vi "main.vi"() -> ()   [LabVIEW 2019]
uses:
  <vilib>/Utility/error.llb/DialogType.ctl
  <vilib>/userDefined/High Color/IMAQdx.ctl
  <vilib>/measure/mamon.llb/Trigger Detection for 1 Channel.vi
  <userlib>/DAQNavi Polymorphic VI/create/DAQNavi Create Channel(AO-Voltage).vi
  <userlib>/DAQNavi Polymorphic VI/create/DAQNavi Create Channel(DO-Digital Output).vi
  <userlib>/DAQNavi Polymorphic VI/create/DAQNavi Create Channel(DI-Digital Input).vi
  <userlib>/DAQNavi Polymorphic VI/read/DAQNavi Read (Digital 1D U8 NChan 1Samp).vi
  Setting Lib.lvlib
  detectedPellet.lvlib
  D03.lvlib
  D04.lvlib
  D05.lvlib
  database.lvlib
  <vilib>/measure/NI_MAPro.lvlib
  User Lib.lvlib
  <vilib>/addons/Fuzzy Logic/NI_Fuzzy_Logic_API.lvlib
  Maintenance.lvlib
  D01.lvlib
  D02.lvlib
  D06.lvlib
panel:
  out "error out 2":errorcluster
  out "task out digital":i32
  out "task out analog":i32
  out "last error 06":dbl
  out "slope D06":dbl
  out "decrease D06":bool
  out "no change D06":bool
  out "increase D06":bool
  out "sudden change D06":bool
  out "In Range":dbl format="%#.2g"
  out "Warning array 06":bool[](array[boolean])
  out "speed  min 06":bool
  out "speed max 06":bool
  out "10-14 6":dbl(slide) caption="10-14 mm" scale=0.0..100.0 scale format="%#.1f"
  out "8-16mm 6":dbl format="%.1g"
  out "AUTO/MAN 06":bool
  out "DISC 06":bool
  out "SPEED 07":dbl caption="SPEED" format="%#.2g"
  out "AVG 07":dbl caption="AVG" format="%#.2g"
  in  "Info 07":bool
  out "Warning 07":bool
  out "disc name 07":string="DISC 07"
  in  "Graph 07":bool
  in  "Live 07":bool
  out "AUTO/MAN 07":bool
  out "projector 07":bool
  out "cam 07":bool
  out "8-12.5 32":dbl(slide) caption="9-12.5 mm" scale=0.0..100.0 scale format="%#.1f"
  out "12.5-16 32":dbl(slide) caption="12.5-16 mm" scale=0.0..100.0 scale format="%#.1f"
  out "DISC 07":bool
  out "SPEED 06":dbl caption="SPEED" format="%.2g"
  out "AVG 06":dbl caption="AVG" format="%#.2g"
  in  "Info 06":bool
  out "Warning 06":bool
  out "disc name 06":string="DISC 06"
  in  "Graph 06":bool
  in  "Live 06":bool
  out "projector 06":bool
  out "cam 06":bool
  out "9.5-12.7 06":dbl(slide) caption="9.5-12.7 mm" scale=0.0..100.0 scale format="%#.1f"
  out "12.7-16 06":dbl(slide) caption="12.7-16 mm" scale=0.0..100.0 scale format="%#.1f"
  out "sudden change D05":bool
  out "slope D05":dbl
  out "increase D05":bool
  out "decrease D05":bool
  out "sudden change D04":bool
  out "slope D04":dbl
  out "increase D04":bool
  out "decrease D04":bool
  out "slope D03":dbl
  out "sudden change D03":bool
  out "increase D03":bool
  out "decrease D03":bool
  out "sudden change D02":bool
  out "slope D02":dbl
  out "increase D02":bool
  out "decrease D02":bool
  out "decrease D01":bool
  out "increase D01":bool
  out "last error 05":dbl
  out "no change D05":bool
  out "last error 04":dbl
  out "no change D04":bool
  out "last error 03":dbl
  out "no change D03":bool
  out "last error 02":dbl
  out "no change D02":bool
  out "sudden change D01":bool
  out "speed  min 05":bool
  out "speed max 05":bool
  out "speed  min 03":bool
  out "speed max 03":bool
  out "speed  min 04":bool
  out "speed max 04":bool
  out "speed  min 02":bool
  out "speed max 02":bool
  out "speed max 01":bool
  out "speed  min 01":bool
  out "no change D01":bool
  out "SPEED 05":dbl caption="SPEED" format="%.2g"
  out "SPEED 04":dbl caption="SPEED" format="%.2g"
  out "SPEED 03":dbl caption="SPEED" format="%.2g"
  out "SPEED 02":dbl caption="SPEED" format="%.2g"
  out "SPEED 01":dbl caption="SPEED" format="%.2g"
  out "AVG 05":dbl caption="AVG" format="%#.2g"
  out "AVG 04":dbl caption="AVG" format="%#.2g"
  out "AVG 03":dbl caption="AVG" format="%#.2g"
  out "AVG 02":dbl caption="AVG" format="%#.2g"
  out "AVG 01":dbl caption="AVG" format="%#.2g"
  out "8-16mm 05":dbl format="%.1g"
  out "8-16mm 04":dbl format="%.1g"
  out "8-16mm 03":dbl format="%.1g"
  out "8-16mm 27":dbl format="%.1g"
  out "8-16mm 26":dbl format="%.1g"
  out "10-14 05":dbl(slide) caption="10-14 mm" scale=0.0..100.0 scale format="%#.1f"
  out "10-14 04":dbl(slide) caption="10-14 mm" scale=0.0..100.0 scale format="%#.1f"
  out "10-14 03":dbl(slide) caption="10-14 mm" scale=0.0..100.0 scale format="%#.1f"
  out "10-14 02":dbl(slide) caption="10-14 mm" scale=0.0..100.0 scale format="%#.1f"
  out "10-14 01":dbl(slide) caption="10-14 mm" scale=0.0..100.0 scale format="%#.1f"
  out "error out 14":errorcluster
  out "error out 12":errorcluster
  in  "Info 05":bool
  in  "Info 04":bool
  in  "Info 03":bool
  in  "Info 02":bool
  in  "Info 01":bool
  out "error out":errorcluster
  out "avg grading array size":i32=4000
  out "live grading array size":i32=2000
  out "2D array out":dbl[][](array[numeric])
  out "Warning array 01":bool[](array[boolean])
  out "Warning array 02":bool[](array[boolean])
  out "Warning array 03":bool[](array[boolean])
  out "Warning array 04":bool[](array[boolean])
  out "Warning array 05":bool[](array[boolean])
  out "Warning 05":bool
  in  "speed disc 30":i32
  in  "speed disc 29":i32
  in  "Error in 18":errorcluster
  in  "speed disc 28":i32
  in  "speed disc 27":i32
  in  "speed disc 26":i32
  out "Warning 04":bool
  out "Warning 03":bool
  out "Warning 02":bool
  out "Warning 01":bool
  out "overal result":string="Overal Result"
  out "disc name 05":string="DISC 05"
  out "disc name 04":string="DISC 04"
  out "disc name 03":string="DISC 03"
  out "disc name 02":string="DISC 02"
  in  "Setting":bool
  out "disc name 01":string="DISC 01"
  in  "Graph 05":bool
  in  "Live 05":bool
  in  "Graph 04":bool
  in  "Live 04":bool
  in  "Graph 03":bool
  in  "Live 03":bool
  in  "Graph 02":bool
  in  "Live 02":bool
  out "Software name":string="DORSA Smart Grading System (DSGS)"
  out "time&date":string="2020/11/22"
  in  "Maintenance":bool
  in  "Shutdown":bool
  in  "Restart":bool
  in  "Close":bool
  in  "View":bool
  in  "Report":bool
  in  "Login":bool=TRUE
  in  "Graph 01":bool
  in  "Live 01":bool
  out "9.5-12.7 02":dbl(slide) caption="9.5-12.7 mm" scale=0.0..100.0 scale format="%#.1f"
  out "12.7-16 02":dbl(slide) caption="12.7-16 mm" scale=0.0..100.0 scale format="%#.1f"
  out "AUTO/MAN 05":bool
  out "projector 05":bool
  out "cam 05":bool
  out "9.5-12.7 05":dbl(slide) caption="9.5-12.7 mm" scale=0.0..100.0 scale format="%#.1f"
  out "12.7-16 05":dbl(slide) caption="12.7-16 mm" scale=0.0..100.0 scale format="%#.1f"
  out "DISC 05":bool
  out "AUTO/MAN 04":bool
  out "projector 04":bool
  out "cam 04":bool
  out "9.5-12.7 04":dbl(slide) caption="9.5-12.7 mm" scale=0.0..100.0 scale format="%#.1f"
  out "12.7-16 04":dbl(slide) caption="12.7-16 mm" scale=0.0..100.0 scale format="%#.1f"
  out "DISC 04":bool
  out "AUTO/MAN 03":bool
  out "projector 03":bool
  out "cam 03":bool
  out "9.5-12.7 03":dbl(slide) caption="9.5-12.7 mm" scale=0.0..100.0 scale format="%#.1f"
  out "12.7-16 03":dbl(slide) caption="12.7-16 mm" scale=0.0..100.0 scale format="%#.1f"
  out "DISC 03":bool
  out "AUTO/MAN 02":bool
  out "projector 02":bool
  out "cam 02":bool
  out "DISC 02":bool
  out "AUTO/MAN 01":bool
  out "projector 01":bool
  out "cam 01":bool
  out "9.5-12.7 01":dbl(slide) caption="9.5-12.7 mm" scale=0.0..100.0 scale format="%#.1f"
  out "12.7-16 01":dbl(slide) caption="12.7-16 mm" scale=0.0..100.0 scale format="%#.1f"
  out "DISC 01":bool
  out "12.7-16 total":dbl(slide) caption="12.7-16 mm" scale=0.0..100.0 scale format="%#.1f"
  out "9.5-12.7 total":dbl(slide) caption="9.5-12.7mm" scale=0.0..100.0 scale format="%#.1f"
  out "Over Size":dbl format="%#.2g"
  out "AVG":dbl format="%#.2g"
  out "Under Size":dbl format="%#.2g"
types:
  T1 = typedef "Image Type" = u32
  T2 = cluster{"disc 06":bool, "auto/man 06":bool, "projector 06":bool, "cam 06":bool}
  T3 = cluster{"disc 05":bool, "auto/man 05":bool, "projector 05":bool, "cam 05":bool}
  T4 = cluster{"disc 04":bool, "auto/man 04":bool, "projector 04":bool, "cam 04":bool}
  T5 = cluster{"disc 03":bool, "auto/man 03":bool, "projector 03":bool, "cam 03":bool}
  T6 = cluster{"disc 02":bool, "auto/man 02":bool, "projector 02":bool, "cam 02":bool}
  T7 = cluster{"disc 01":bool, "auto/man 01":bool, "projector 01":bool, "cam 01":bool}
  T8 = typedef "DialogType.ctl" = u16
  T9 = typedef "IMAQ Image.ctl" = refnum<image>
  T10 = cluster{"disc 01":bool, "auto/man 01":bool, "projector 01":bool, "cam 01":bool}[]
  T11 = cluster{"disc 02":bool, "auto/man 02":bool, "projector 02":bool, "cam 02":bool}[]
  T12 = cluster{"disc 06":bool, "auto/man 06":bool, "projector 06":bool, "cam 06":bool}[]
  T13 = cluster{"disc 05":bool, "auto/man 05":bool, "projector 05":bool, "cam 05":bool}[]
  T14 = cluster{"disc 03":bool, "auto/man 03":bool, "projector 03":bool, "cam 03":bool}[]
  T15 = cluster{"disc 04":bool, "auto/man 04":bool, "projector 04":bool, "cam 04":bool}[]
  T16 = enum32{"Invalid", "Standard", "Closed", "Hidden", "Minimized", "Maximized"}
  T17 = typedef "IMAQdx.ctl" = refnum<k21>
  T18 = enum8{"Enabled", "Disabled", "Disabled and Grayed Out"}
  T19 = cluster{string, "date/time string":string, "date/time string":string, string}
  T20 = cluster{i32, "date/time string":string, "date/time string":string, string}
  T21 = typedef "NI_Fuzzy_Logic_API.lvlib/FL System.ctl" = cluster{"input variables":T22[], "output variables":T22[], "rules":T25[], "defuzzification method":T31, "description":string, "user MF interpolating polynomials":T32[]}
  T22 = typedef "NI_Fuzzy_Logic_API.lvlib/FL Variable.ctl" = cluster{"name":string, "range":dbl[], "MFs":T23[]}
  T23 = typedef "NI_Fuzzy_Logic_API.lvlib/FL Membership Function.ctl" = cluster{"name":string, "shape":T24, "points":dbl[], "color":u32, "user-defined shape index":i32}
  T24 = typedef "NI_Fuzzy_Logic_API.lvlib/FL Membership Function Shape.ctl" = u16
  T25 = typedef "NI_Fuzzy_Logic_API.lvlib/FL Rule.ctl" = cluster{"antecedents":T26[], "antecedent connective":T28, "consequents":T29[], "consequent implication":T30, "degree of support":dbl}
  T26 = typedef "NI_Fuzzy_Logic_API.lvlib/FL Antecedent.ctl" = cluster{"Var Index":i32, "MF Index":i32, "Cond":T27}
  T27 = typedef "NI_Fuzzy_Logic_API.lvlib/FL Modifier.ctl" = u16
  T28 = typedef "NI_Fuzzy_Logic_API.lvlib/FL Antecedent Connective.ctl" = u16
  T29 = typedef "NI_Fuzzy_Logic_API.lvlib/FL Consequent.ctl" = cluster{"Var Index":i32, "MF Index":i32, "Cond":T27}
  T30 = typedef "NI_Fuzzy_Logic_API.lvlib/FL Consequent Implication.ctl" = u16
  T31 = typedef "NI_Fuzzy_Logic_API.lvlib/FL Defuzzification.ctl" = u16
  T32 = typedef "NI_Fuzzy_Logic_API.lvlib/FL Interpolating polynomials.ctl" = cluster{"X":dbl[], "Y":dbl[], "Y(x) coeff":dbl[][], "X(y) coeff":dbl[][], "Area(y) coeff":dbl[][], "coa_x(y) coeff":dbl[][]}
  T33 = cluster{"dec":bool, "inc":bool, "no change":bool, "Value":bool, "last error ":dbl, "Value":dbl, "output value":dbl, "slope ":dbl}
  T34 = cluster{"dec":bool, "inc":bool, "no change":bool, "sudden change":bool, "last error ":dbl, "Value":dbl, "output value":dbl, "slope ":dbl}
  T35 = typedef "LVDateTimeRec.ctl" = cluster{"fractional second":dbl, "second":i32, "minute":i32, "hour":i32, "day of month":i32, "month":i32, "year":i32, "day of week":i32, "day of year":i32, "DST":i32}
  T36 = cluster{"date/time string":string, "date/time string":string, dbl, dbl, dbl, dbl, dbl, dbl, dbl, dbl, "f":string, "f":string, "time format string (%c)":string, "time format string (%c)":string}
  T37 = cluster{"date/time string":string, "date/time string":string, dbl, dbl, "f":string, "f":string, "time format string (%c)":string, "time format string (%c)":string}
  T38 = cluster{"date/time string":string, "date/time string":string, string, "spreadsheet string":string}
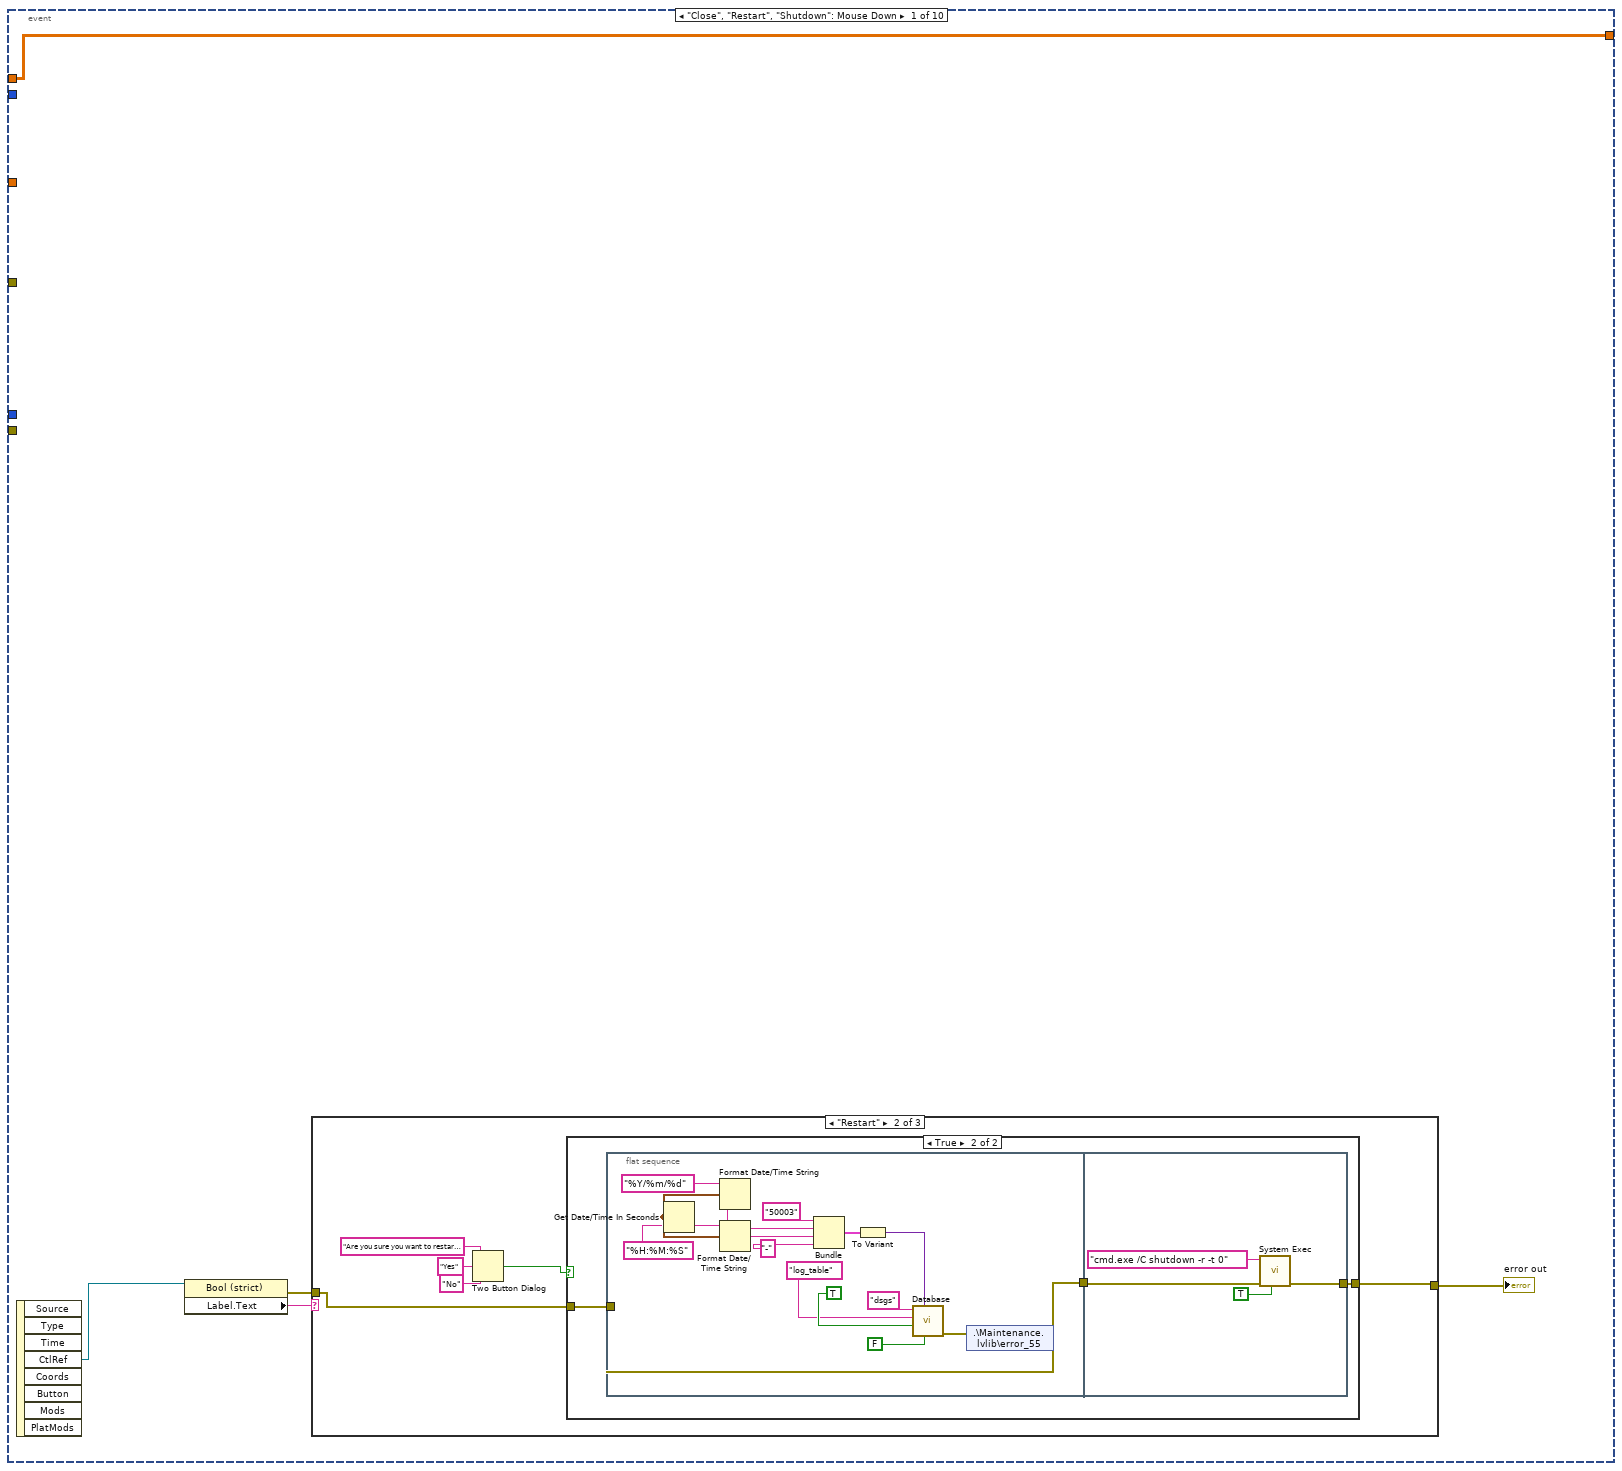
[diagram p14: hidden frame]
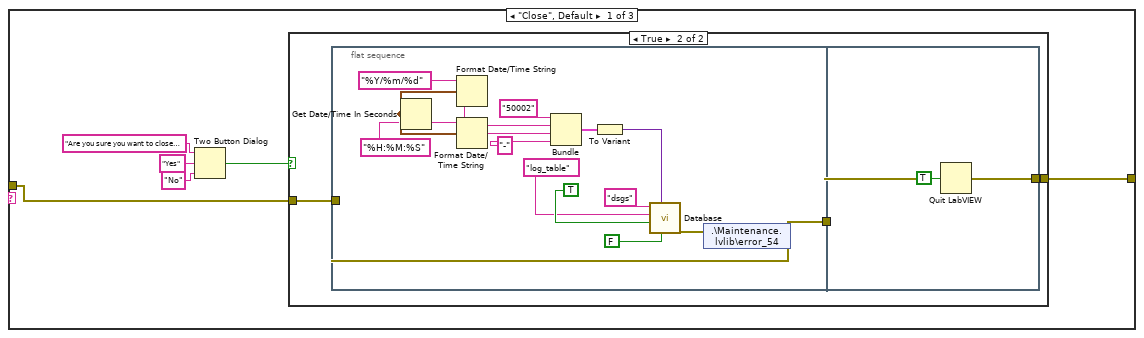
[diagram p15: hidden frame]
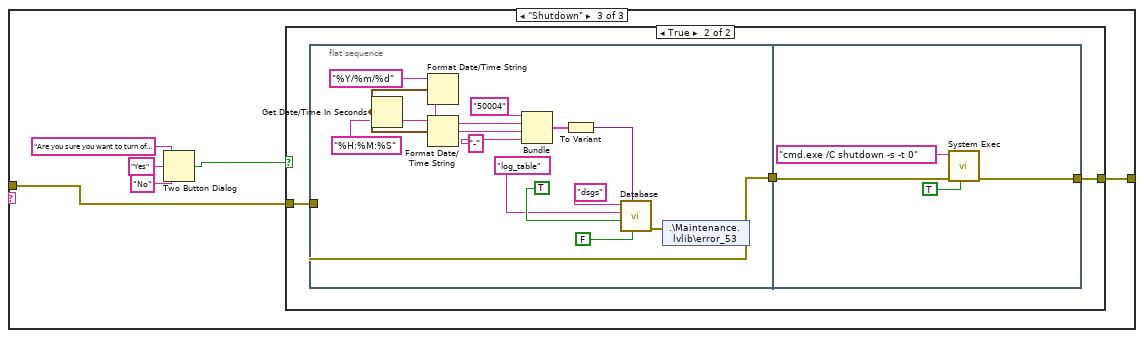
[diagram p18: hidden frame]
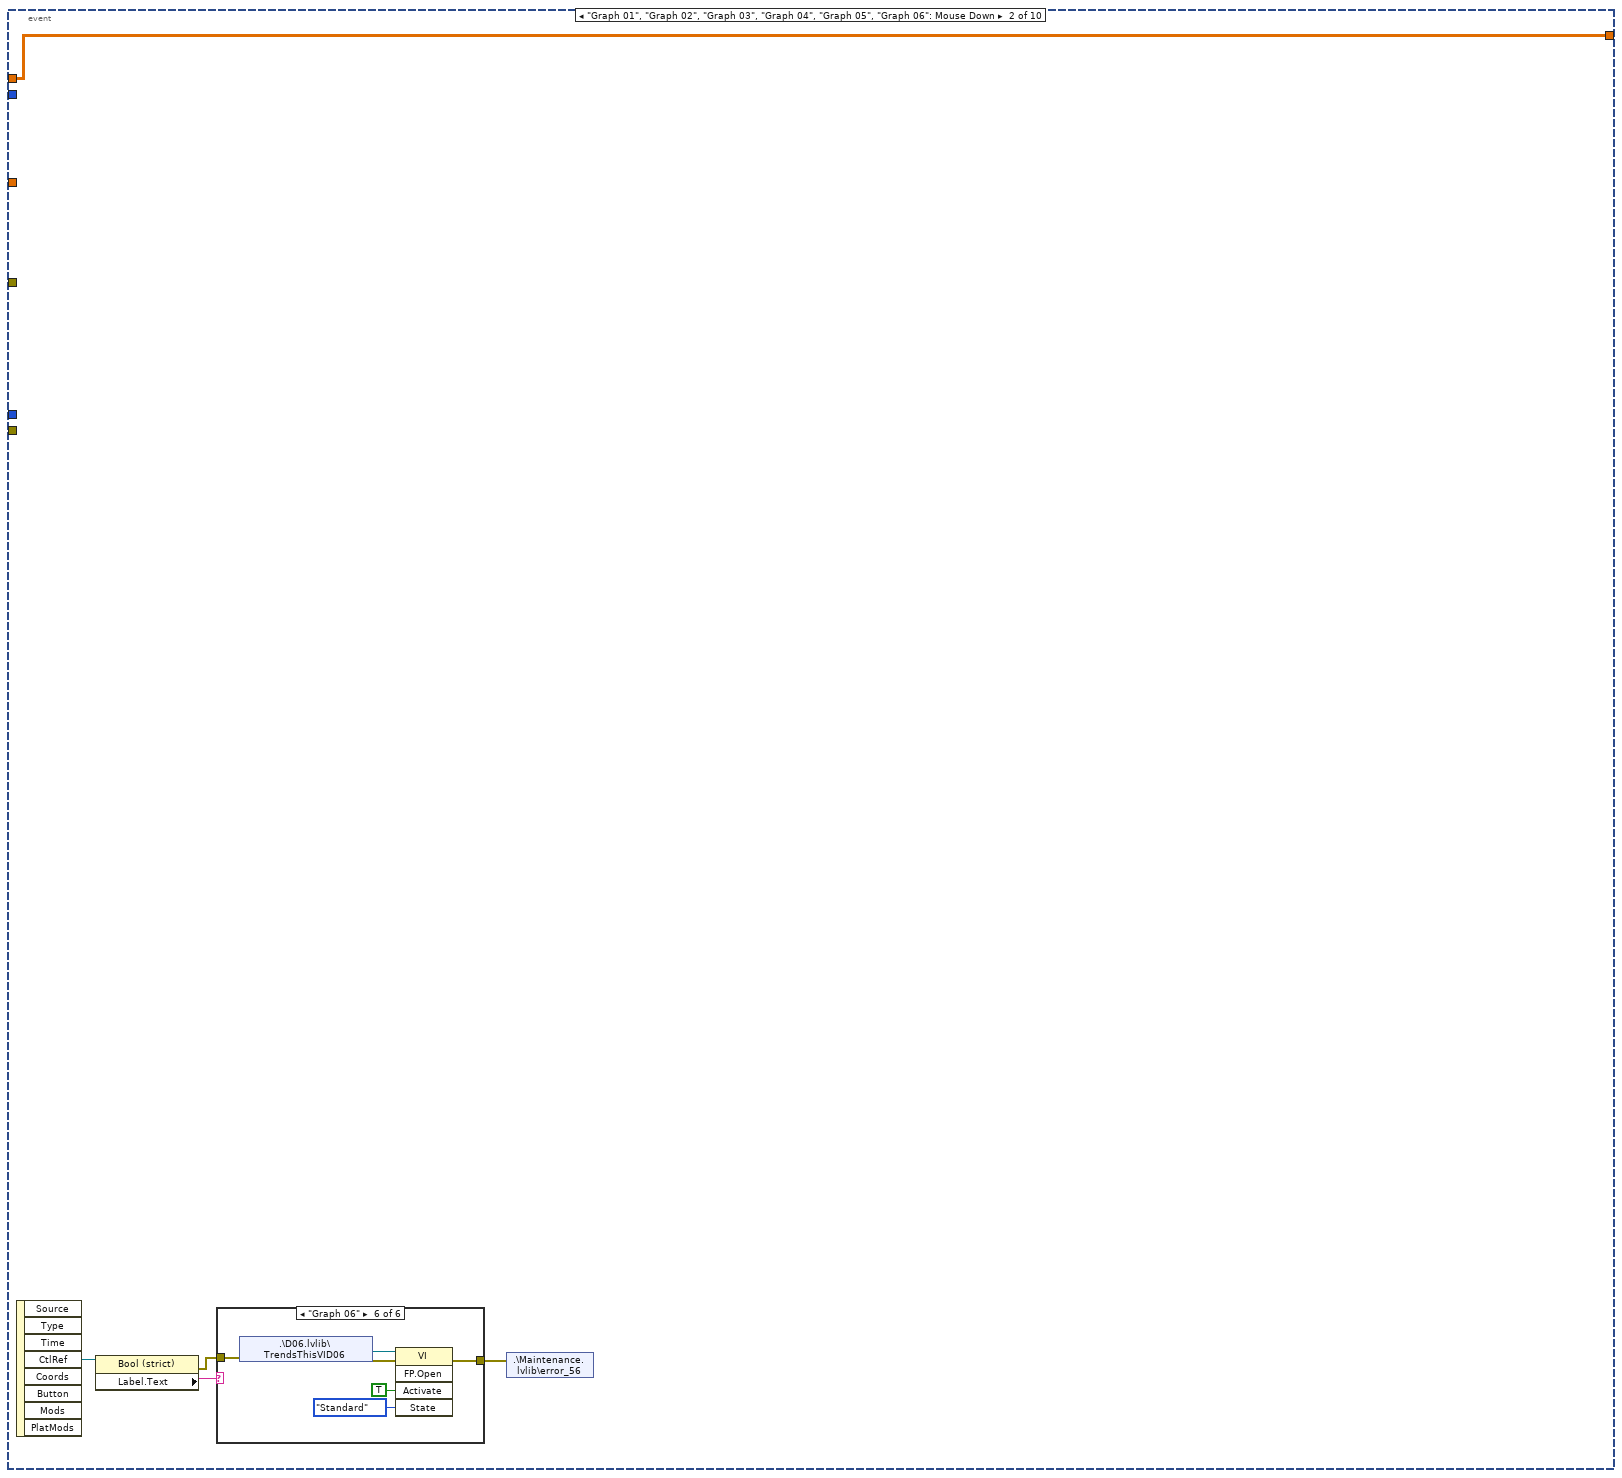
[diagram p20: hidden frame]
diagram:
  w25 = 200 ("dimension size")
  w29 = T1 0 items=["Grayscale (U8)", "Grayscale (I16)", "Grayscale (SGL)", "Complex (CSG)", "RGB (U32)", "HSL (U32)", "RGB (U64)", "Grayscale (U16)"] ("Image Type")
  w30 = T1 0 items=["Grayscale (U8)", "Grayscale (I16)", "Grayscale (SGL)", "Complex (CSG)", "RGB (U32)", "HSL (U32)", "RGB (U64)", "Grayscale (U16)"] ("Image Type")
  w31 = T1 0 items=["Grayscale (U8)", "Grayscale (I16)", "Grayscale (SGL)", "Complex (CSG)", "RGB (U32)", "HSL (U32)", "RGB (U64)", "Grayscale (U16)"] ("Image Type")
  w32 = T1 0 items=["Grayscale (U8)", "Grayscale (I16)", "Grayscale (SGL)", "Complex (CSG)", "RGB (U32)", "HSL (U32)", "RGB (U64)", "Grayscale (U16)"] ("Image Type")
  w33 = T1 0 items=["Grayscale (U8)", "Grayscale (I16)", "Grayscale (SGL)", "Complex (CSG)", "RGB (U32)", "HSL (U32)", "RGB (U64)", "Grayscale (U16)"] ("Image Type")
  w34 = T1 0 items=["Grayscale (U8)", "Grayscale (I16)", "Grayscale (SGL)", "Complex (CSG)", "RGB (U32)", "HSL (U32)", "RGB (U64)", "Grayscale (U16)"] ("Image Type")
  w100 = 4000 ("dimension size")
  w105 = 1000 ("dimension size")
  n1 = while {
    tunnel: [w137] -> w28
    tunnel: [w136] -> w23
    stop <- w125 stop-if-true
    w132 = T8 0 items=["no dialog", "OK message", "continue or stop message", "OK message + warnings", "continue/stop + warnings"] ("type of dialog (OK msg:1)")
    n2 = TCP Open Connection(address="169.254.114.6", remote port or service name=u16 502, timeout ms (60000)=-1, error in (no error)=errorcluster {"status"=FALSE, "code"=0, "source"=""}) -> (connection ID=w137:refnum<k5>, error out=w134:errorcluster)  [unwired: 1 in]
    n3 = call <vilib>:"Simple Error Handler.vi"("type of dialog (OK msg:1)"=w132, "error in (no error)"=w134) -> ("error?"=w133:bool, "error out"=w136:errorcluster)  [unwired: 3 in, 3 out]
    n4 = Not(x=w133) -> (.not. x?=w130:bool)
    n5 = Or(x=FALSE, y=w130) -> (x .or. y?=w125:bool)
    n6 = Wait (ms)(milliseconds to wait=u32 5) -> ()  [unwired: 1 out]
  }
  n7 = call "DAQNavi_Property_Assistant"() -> ("property value"=w12:string)  [unwired: 1 in]
  n8 = call "IMAQ Create"("Image Name"="img in D01", "Image Type"=w34) -> ("New Image"=w74:T9, "error out"=w65:errorcluster)  [unwired: 3 in]
  n9 = shared-variable ".\\Maintenance.lvlib\\error_2"(w65) -> ()  [unwired: 1 in, 1 out]
  n10 = call "IMAQ Create"("Image Name"="img in D02", "Image Type"=w33) -> ("New Image"=w51:T9, "error out"=w64:errorcluster)  [unwired: 3 in]
  n11 = shared-variable ".\\Maintenance.lvlib\\error_3"(w64) -> ()  [unwired: 1 in, 1 out]
  n12 = call-poly <userlib>:"DAQNavi Create Channel.vi"("physical channels"="PCI-1710,BID#0/ao0", "value range"=w12, "error in (no error)"=errorcluster {"status"=FALSE, "code"=0, "source"=""}) -> ("task out"=→"task out analog":i32, "error out"=w14:errorcluster)  [unwired: 11 in]
  n13 = call "IMAQ Create"("Image Name"="img in D03", "Image Type"=w32) -> ("New Image"=w69:T9, "error out"=w63:errorcluster)  [unwired: 3 in]
  n14 = shared-variable ".\\Maintenance.lvlib\\error_4"(w63) -> ()  [unwired: 1 in, 1 out]
  n15 = call "IMAQ Create"("Image Name"="img in D04", "Image Type"=w31) -> ("New Image"=w68:T9, "error out"=w62:errorcluster)  [unwired: 3 in]
  n16 = shared-variable ".\\Maintenance.lvlib\\error_5"(w62) -> ()  [unwired: 1 in, 1 out]
  n17 = call "IMAQ Create"("Image Name"="img in D05", "Image Type"=w30) -> ("New Image"=w67:T9, "error out"=w61:errorcluster)  [unwired: 3 in]
  n18 = call "IMAQ Create"("Image Name"="img out D01") -> ("New Image"=w116:T9, "error out"=w60:errorcluster)  [unwired: 4 in]
  n19 = shared-variable ".\\Maintenance.lvlib\\error_6"(w61) -> ()  [unwired: 1 in, 1 out]
  n20 = shared-variable ".\\Maintenance.lvlib\\error_7"(w60) -> ()  [unwired: 1 in, 1 out]
  n21 = call-poly <userlib>:"DAQNavi Create Channel.vi"("physical channels"="PCI-1710,BID#0/port0", "error in (no error)"=w14) -> ("task out"=→"task out digital":i32, "error out"=w17:errorcluster)  [unwired: 12 in]
  n22 = call "IMAQ Create"("Image Name"="img out D02") -> ("New Image"=w114:T9, "error out"=w59:errorcluster)  [unwired: 4 in]
  n23 = call "IMAQ Create"("Image Name"="img in D06", "Image Type"=w29) -> ("New Image"=w49:T9)  [unwired: 3 in, 1 out]
  n24 = shared-variable ".\\Maintenance.lvlib\\error_8"(w59) -> ()  [unwired: 1 in, 1 out]
  n25 = call "IMAQ Create"("Image Name"="img out D03") -> ("New Image"=w112:T9, "error out"=w58:errorcluster)  [unwired: 4 in]
  n26 = shared-variable ".\\Maintenance.lvlib\\error_9"(w58) -> ()  [unwired: 1 in, 1 out]
  n27 = call "IMAQ Create"("Image Name"="img out D04") -> ("New Image"=w109:T9, "error out"=w57:errorcluster)  [unwired: 4 in]
  n28 = shared-variable ".\\Maintenance.lvlib\\error_10"(w57) -> ()  [unwired: 1 in, 1 out]
  n29 = Initialize Array(0.0 ("element"), w100, 6 ("dimension size")) -> (w101:dbl[][])
  n30 = call "IMAQ Create"("Image Name"="img out D05") -> ("New Image"=w108:T9, "error out"=w56:errorcluster)  [unwired: 4 in]
  n31 = call-poly <userlib>:"DAQNavi Create Channel.vi"("physical channels"="PCI-1710,BID#0/port0:1", "error in (no error)"=w17) -> ("task out"=w18:i32, "error out"=w7:errorcluster)  [unwired: 12 in]
  n32 = shared-variable ".\\Maintenance.lvlib\\error_11"(w56) -> ()  [unwired: 1 in, 1 out]
  n33 = Wait (ms)(milliseconds to wait=u32 5) -> ()  [unwired: 1 out]
  n34 = Initialize Array(0.0 ("element"), w105, 6 ("dimension size")) -> (w106:dbl[][])
  n35 = Open Python Session(python version="3.6" ("Python version"), 3:errorcluster {"status"=FALSE, "code"=0, "source"=""} ("error in (no error)")) -> (session out=w123:refnum<k35>, error out=w66:errorcluster)  [unwired: 1 in]
  n36 = shared-variable ".\\Maintenance.lvlib\\error_1"(w66) -> ()  [unwired: 1 in, 1 out]
  n37 = Initialize Array(12.0 ("element"), 60 ("dimension size"), 6 ("dimension size")) -> (w99:dbl[][])
  n38 = Initialize Array(0.0 ("element"), 600 ("dimension size"), 3 ("dimension size")) -> (w118:dbl[][])
  n39 = call "IMAQ Create"("Image Name"="img out D06") -> ("New Image"=w47:T9)  [unwired: 4 in, 1 out]
  n40 = Initialize Array(T7 {"disc 01"=FALSE, "auto/man 01"=FALSE, "projector 01"=FALSE, "cam 01"=FALSE}, 2 ("dimension size")) -> (w92:T10)
  n41 = Initialize Array(T6 {"disc 02"=FALSE, "auto/man 02"=FALSE, "projector 02"=FALSE, "cam 02"=FALSE}, 2 ("dimension size")) -> (w89:T11)
  n42 = Initialize Array(T2 {"disc 06"=FALSE, "auto/man 06"=FALSE, "projector 06"=FALSE, "cam 06"=FALSE}, 2 ("dimension size")) -> (w44:T12)
  n43 = Initialize Array(T3 {"disc 05"=FALSE, "auto/man 05"=FALSE, "projector 05"=FALSE, "cam 05"=FALSE}, 2 ("dimension size")) -> (w80:T13)
  n44 = Initialize Array(T5 {"disc 03"=FALSE, "auto/man 03"=FALSE, "projector 03"=FALSE, "cam 03"=FALSE}, 2 ("dimension size")) -> (w84:T14)
  n45 = Initialize Array(T4 {"disc 04"=FALSE, "auto/man 04"=FALSE, "projector 04"=FALSE, "cam 04"=FALSE}, 2 ("dimension size")) -> (w83:T15)
  n46 = Initialize Array(0.0 ("element"), w25, 6 ("dimension size")) -> (w24:dbl[][])
  n47 = while {
    tunnel: w23 -> [w145]
    tunnel: w18 -> [w142]
    tunnel: w28 -> [w146]
    shift-right: [w148] -> _
    shift-left: w24 -> [w147]
    tunnel: w25 -> [w149]
    tunnel: w7 -> [w139]
    tunnel: [w138] -> w6
    stop <- FALSE stop-if-true
    n48 = call "adamread.vi"("TCP Connection Refnum in"=w146, "error in (no error)"=w145) -> ("Slave Input Registers 2"=w144:dbl[], "error out 2"=w143:errorcluster)  [unwired: 11 in, 1 out]
    n49 = call-poly <userlib>:"DAQNavi Read.vi"("error in (no error)"=w139, "task in"=w142) -> ("error out"=w140:errorcluster, "data"=w141:u8[], "task out"=w138:i32)  [unwired: 7 in]
    n50 = event shown="[9] Timeout" {
      selector: _ -> [_ _ _ _ _ _ _ _ _ _]
      dyn-events: _ -> [_ _ _ _ _ _ _ _ _ _]
      timeout: 0 -> [_ _ _ _ _ _ _ _ _ _]
      tunnel: w147 -> [w153 w243 w284 w328 w336 w344 w354 w403 w418 w646]
      tunnel: w149 -> [_ _ _ _ _ _ _ _ _ w645]
      tunnel: [w153 w243 w284 w328 w336 w344 w354 w403 w418 w643] -> w148
      tunnel: w144 -> [_ _ _ _ _ _ _ _ _ w642]
      tunnel: w143 -> [_ _ _ _ _ _ _ _ _ w641]
      tunnel: w141 -> [_ _ _ _ _ _ _ _ _ w640]
      tunnel: w140 -> [_ _ _ _ _ _ _ _ _ w639]
      event "Close", "Restart", "Shutdown": Mouse Down {
        n51 = event-data() -> ("CtlRef"=w156:refnum<vi>)  [unwired: 1 in, 7 out]
        n52 = property class="Bool (strict)"(reference=w156) -> (error out=w155:errorcluster, "Label.Text"=w157:string)  [unwired: 1 in, 1 out]
        n53 = case shown="\"Restart\"" w157 {
          tunnel: [w158 w185 w215] -> w154
          tunnel: w155 -> [w159 w186 w214]
          frame "Close", Default {
            n54 = Two Button Dialog(message="Are you sure you want to close the application?", 1:"No" ("F button name (\"Cancel\")"), 2:"Yes" ("T button name (\"OK\")")) -> (T button?=w160:bool)
            n55 = case shown="True" w160 {
              tunnel: w159 -> [w164 w165]
              tunnel: [w164 w167] -> w158
              frame False {
              }
              frame True {
                n56 = flat-sequence {
                  tunnel: [w168] -> w166
                  tunnel: w165 -> [w168]
                  tunnel: [w183] -> w167
                  tunnel: w166 -> [w183]
                  frame #0 {
                    n57 = Get Date/Time In Seconds() -> (seconds since 1Jan1904=w178:timestamp)
                    n58 = Format Date/Time String(time format string (%c)="%Y/%m/%d", seconds (now)=w178) -> (date/time string=w179:string)  [unwired: 1 in]
                    n59 = Format Date/Time String(time format string (%c)="%H:%M:%S", seconds (now)=w178) -> (date/time string=w180:string)  [unwired: 1 in]
                    n60 = Bundle("50002", "date/time string"=w179, "date/time string"=w180, "-") -> (w181:T19)  [unwired: 1 in]
                    n61 = To Variant(anything=w181) -> (Variant=w182:variant)
                    n62 = call "Database.vi"("Delete row?"=FALSE, "Data"=w182, "Auto Increment ID?"=TRUE, "Table"="log_table", "Connection"="dsgs") -> ("Error out"=w169:errorcluster)  [unwired: 6 in]
                    n63 = shared-variable ".\\Maintenance.lvlib\\error_54"(w169) -> ()  [unwired: 1 in, 1 out]
                  }
                  frame #1 {
                    n64 = Quit LabVIEW(quit? (T)=TRUE) -> ()
                  }
                }
              }
            }
          }
          frame "Restart" {
            n65 = Two Button Dialog(message="Are you sure you want to restart the system?", 1:"No" ("F button name (\"Cancel\")"), 2:"Yes" ("T button name (\"OK\")")) -> (T button?=w187:bool)
            n66 = case shown="True" w187 {
              tunnel: w186 -> [w191 w194]
              tunnel: [w191 w192] -> w185
              frame False {
              }
              frame True {
                n67 = flat-sequence {
                  tunnel: w194 -> [w196]
                  tunnel: [w196] -> w193
                  tunnel: w193 -> [w211]
                  tunnel: [w210] -> w192
                  frame #0 {
                    n68 = Get Date/Time In Seconds() -> (seconds since 1Jan1904=w205:timestamp)
                    n69 = Format Date/Time String(time format string (%c)="%Y/%m/%d", seconds (now)=w205) -> (date/time string=w206:string)  [unwired: 1 in]
                    n70 = Format Date/Time String(time format string (%c)="%H:%M:%S", seconds (now)=w205) -> (date/time string=w207:string)  [unwired: 1 in]
                    n71 = Bundle("50003", "date/time string"=w206, "date/time string"=w207, "-") -> (w208:T19)  [unwired: 1 in]
                    n72 = To Variant(anything=w208) -> (Variant=w209:variant)
                    n73 = call "Database.vi"("Delete row?"=FALSE, "Data"=w209, "Auto Increment ID?"=TRUE, "Table"="log_table", "Connection"="dsgs") -> ("Error out"=w195:errorcluster)  [unwired: 6 in]
                    n74 = shared-variable ".\\Maintenance.lvlib\\error_55"(w195) -> ()  [unwired: 1 in, 1 out]
                  }
                  frame #1 {
                    n75 = call <vilib>:"System Exec.vi"("run minimized? (F)"=TRUE, "error in (no error)"=w211, "command line"="cmd.exe /C shutdown -r -t 0") -> ("error out"=w210:errorcluster)  [unwired: 5 in, 3 out]
                  }
                }
              }
            }
          }
          frame "Shutdown" {
            n76 = Two Button Dialog(message="Are you sure you want to turn off the system?", 1:"No" ("F button name (\"Cancel\")"), 2:"Yes" ("T button name (\"OK\")")) -> (T button?=w216:bool)
            n77 = case shown="True" w216 {
              tunnel: [w220 w223] -> w215
              tunnel: w214 -> [w220 w222]
              frame False {
              }
              frame True {
                n78 = flat-sequence {
                  tunnel: w222 -> [w224]
                  tunnel: [w224] -> w221
                  tunnel: [w240] -> w223
                  tunnel: w221 -> [w239]
                  frame #0 {
                    n79 = Get Date/Time In Seconds() -> (seconds since 1Jan1904=w234:timestamp)
                    n80 = Format Date/Time String(time format string (%c)="%Y/%m/%d", seconds (now)=w234) -> (date/time string=w235:string)  [unwired: 1 in]
                    n81 = Format Date/Time String(time format string (%c)="%H:%M:%S", seconds (now)=w234) -> (date/time string=w236:string)  [unwired: 1 in]
                    n82 = Bundle("50004", "date/time string"=w235, "date/time string"=w236, "-") -> (w237:T19)  [unwired: 1 in]
                    n83 = To Variant(anything=w237) -> (Variant=w238:variant)
                    n84 = call "Database.vi"("Delete row?"=FALSE, "Data"=w238, "Auto Increment ID?"=TRUE, "Table"="log_table", "Connection"="dsgs") -> ("Error out"=w225:errorcluster)  [unwired: 6 in]
                    n85 = shared-variable ".\\Maintenance.lvlib\\error_53"(w225) -> ()  [unwired: 1 in, 1 out]
                  }
                  frame #1 {
                    n86 = call <vilib>:"System Exec.vi"("run minimized? (F)"=TRUE, "error in (no error)"=w239, "command line"="cmd.exe /C shutdown -s -t 0") -> ("error out"=w240:errorcluster)  [unwired: 5 in, 3 out]
                  }
                }
              }
            }
          }
        }
        "error out" <- w154
      }
      event "Graph 01", "Graph 02", "Graph 03", "Graph 04", "Graph 05", "Graph 06": Mouse Down {
        n87 = event-data() -> ("CtlRef"=w245:refnum<vi>)  [unwired: 1 in, 7 out]
        n88 = property class="Bool (strict)"(reference=w245) -> (error out=w246:errorcluster, "Label.Text"=w247:string)  [unwired: 1 in, 1 out]
        n89 = case shown="\"Graph 06\"" w247 {
          tunnel: w246 -> [w250 w255 w261 w267 w273 w279]
          tunnel: [w248 w254 w260 w266 w272 w278] -> w244
          frame "Graph 01", Default {
            n90 = shared-variable ".\\D01.lvlib\\TrendsThisVID01"(error in=w250) -> (w253:refnum<vi>, error out=w249:errorcluster)
            n91 = invoke class="VI" method="FP.Open"(reference=w253, error in=w249, "Activate"=TRUE ("Activate?"), "State"=T16."Standard") -> (error out=w248:errorcluster)  [unwired: 1 in, 4 out]
          }
          frame "Graph 02" {
            n92 = shared-variable ".\\D02.lvlib\\TrendsThisVID02"(error in=w255) -> (w258:refnum<vi>, error out=w259:errorcluster)
            n93 = invoke class="VI" method="FP.Open"(reference=w258, error in=w259, "Activate"=TRUE ("Activate?"), "State"=T16."Standard") -> (error out=w254:errorcluster)  [unwired: 1 in, 4 out]
          }
          frame "Graph 03" {
            n94 = shared-variable ".\\D03.lvlib\\TrendsThisVID03"(error in=w261) -> (w264:refnum<vi>, error out=w265:errorcluster)
            n95 = invoke class="VI" method="FP.Open"(reference=w264, error in=w265, "Activate"=TRUE ("Activate?"), "State"=T16."Standard") -> (error out=w260:errorcluster)  [unwired: 1 in, 4 out]
          }
          frame "Graph 04" {
            n96 = shared-variable ".\\D04.lvlib\\TrendsThisVID04"(error in=w267) -> (w270:refnum<vi>, error out=w271:errorcluster)
            n97 = invoke class="VI" method="FP.Open"(reference=w270, error in=w271, "Activate"=TRUE ("Activate?"), "State"=T16."Standard") -> (error out=w266:errorcluster)  [unwired: 1 in, 4 out]
          }
          frame "Graph 05" {
            n98 = shared-variable ".\\D05.lvlib\\TrendsThisVID05"(error in=w273) -> (w276:refnum<vi>, error out=w277:errorcluster)
            n99 = invoke class="VI" method="FP.Open"(reference=w276, error in=w277, "Activate"=TRUE ("Activate?"), "State"=T16."Standard") -> (error out=w272:errorcluster)  [unwired: 1 in, 4 out]
          }
          frame "Graph 06" {
            n100 = shared-variable ".\\D06.lvlib\\TrendsThisVID06"(error in=w279) -> (w282:refnum<vi>, error out=w283:errorcluster)
            n101 = invoke class="VI" method="FP.Open"(reference=w282, error in=w283, "Activate"=TRUE ("Activate?"), "State"=T16."Standard") -> (error out=w278:errorcluster)  [unwired: 1 in, 4 out]
          }
        }
        n102 = shared-variable ".\\Maintenance.lvlib\\error_56"(w244) -> ()  [unwired: 1 in, 1 out]
      }
      event "Login": Mouse Down {
        n103 = event-data() -> ("CtlRef"=w287:refnum<vi>)  [unwired: 1 in, 7 out]
        n104 = property class="Bool (strict)"(reference=w287) -> (error out=w285:errorcluster, "Value"=w286:bool)  [unwired: 1 in, 1 out]
        n105 = case shown="True" w286 {
          tunnel: w285 -> [w288 w297]
          frame True {
            n106 = flat-sequence {
              tunnel: w288 -> [w293]
              frame #0 {
                n107 = shared-variable ".\\User Lib.lvlib\\Login"() -> (w292:refnum<vi>)  [unwired: 1 in, 1 out]
                n108 = invoke class="VI" method="FP.Open"(reference=w292, error in=w293, "Activate"=FALSE ("Activate?"), "State"=T16."Standard") -> (error out=w289:errorcluster)  [unwired: 1 in, 4 out]
                n109 = shared-variable ".\\Maintenance.lvlib\\error_58"(w289) -> ()  [unwired: 1 in, 1 out]
              }
              frame #1 {
                n110 = shared-variable ".\\User Lib.lvlib\\focus"() -> (w295:refnum<vi>)  [unwired: 1 in, 1 out]
                n111 = property class="Str"(reference=w295, "Key Focus"=TRUE) -> ()  [unwired: 1 in, 2 out]
              }
            }
          }
          frame False {
            n112 = flat-sequence {
              tunnel: w297 -> [w299]
              tunnel: [w316] -> w296
              tunnel: w296 -> [w323]
              frame #0 {
                n113 = shared-variable ".\\User Lib.lvlib\\Username"() -> (w315:string)  [unwired: 1 in, 1 out]
                n114 = Get Date/Time In Seconds() -> (seconds since 1Jan1904=w313:timestamp)
                n115 = Format Date/Time String(time format string (%c)="%Y/%m/%d", seconds (now)=w313) -> (date/time string=w312:string)  [unwired: 1 in]
                n116 = Format Date/Time String(time format string (%c)="%H:%M:%S", seconds (now)=w313) -> (date/time string=w311:string)  [unwired: 1 in]
                n117 = Concatenate Strings("Username = \"" ("string"), w315, "\" is logged out." ("string")) -> (w314:string)
                n118 = Bundle(50006, "date/time string"=w312, "date/time string"=w311, w314) -> (w310:T20)  [unwired: 1 in]
                n119 = To Variant(anything=w310) -> (Variant=w309:variant)
                n120 = call "Database.vi"("Delete row?"=FALSE, "Data"=w309, "Error in"=w299, "Auto Increment ID?"=TRUE, "Table"="log_table" ("table"), "Connection"="dsgs" ("table")) -> ("Error out"=w298:errorcluster)  [unwired: 5 in]
                n121 = shared-variable ".\\Maintenance.lvlib\\error_57"(w298) -> ()  [unwired: 1 in, 1 out]
              }
              frame #1 {
                n122 = shared-variable ".\\User Lib.lvlib\\Username"() -> (w318:string, error out=w316:errorcluster)  [unwired: 1 in]
                n123 = Concatenate Strings(w318, " is logout." ("string")) -> (w319:string)
                n124 = One Button Dialog(message=w319) -> ()  [unwired: 1 in, 1 out]
              }
              frame #2 {
                n125 = shared-variable ".\\User Lib.lvlib\\Is Admin?"(FALSE ("Is Admin?"), error in=w323) -> (error out=w322:errorcluster)
                n126 = shared-variable ".\\User Lib.lvlib\\Is Dorsa?"(FALSE ("Is Admin?")) -> ()  [unwired: 1 in, 1 out]
                n127 = property on="Login" class="Bool (strict)"("Value"=TRUE ("Login")) -> ()  [unwired: 2 in, 2 out]
                n128 = shared-variable ".\\User Lib.lvlib\\User Flag"(FALSE ("User Flag"), error in=w322) -> (error out=w321:errorcluster)
                n129 = shared-variable ".\\User Lib.lvlib\\Username"("" ("Username"), error in=w321) -> ()  [unwired: 1 out]
              }
            }
          }
        }
      }
      event "Maintenance": Mouse Down {
        n130 = event-data() -> ("CtlRef"=w330:refnum<vi>)  [unwired: 1 in, 7 out]
        n131 = property class="Bool (strict)"(reference=w330) -> ("DisabledEnum"=w329:T18)  [unwired: 1 in, 2 out]
        n132 = case shown="\"Enabled\"" w329 {
          frame "Enabled" {
            n133 = shared-variable ".\\Maintenance.lvlib\\MaintenanceThisVI"() -> (w335:refnum<vi>, error out=w334:errorcluster)  [unwired: 1 in]
            n134 = invoke class="VI" method="FP.Open"(reference=w335, error in=w334, "Activate"=FALSE ("Activate?"), "State"=T16."Standard") -> (error out=w333:errorcluster)  [unwired: 1 in, 4 out]
            n135 = shared-variable ".\\Maintenance.lvlib\\error_59"(w333) -> ()  [unwired: 1 in, 1 out]
          }
          frame "Disabled", Default {
          }
        }
      }
      event "Report": Mouse Down {
        n136 = event-data() -> ("CtlRef"=w338:refnum<vi>)  [unwired: 1 in, 7 out]
        n137 = property class="Bool (strict)"(reference=w338) -> ("DisabledEnum"=w337:T18)  [unwired: 1 in, 2 out]
        n138 = case shown="\"Enabled\"" w337 {
          frame "Enabled" {
            n139 = shared-variable ".\\database.lvlib\\ReportThisVI"() -> (w341:refnum<vi>, error out=w343:errorcluster)  [unwired: 1 in]
            n140 = invoke class="VI" method="FP.Open"(reference=w341, error in=w343, "Activate"=FALSE ("Activate?"), "State"=T16."Standard") -> (error out=w342:errorcluster)  [unwired: 1 in, 4 out]
            n141 = shared-variable ".\\Maintenance.lvlib\\error_60"(w342) -> ()  [unwired: 1 in, 1 out]
          }
          frame "Disabled", Default {
          }
        }
      }
      event "Setting": Mouse Down {
        n142 = event-data() -> ("CtlRef"=w347:refnum<vi>)  [unwired: 1 in, 7 out]
        n143 = property class="Bool (strict)"(reference=w347) -> (error out=w345:errorcluster, "DisabledEnum"=w346:T18)  [unwired: 1 in, 1 out]
        n144 = case shown="\"Enabled\"" w346 {
          tunnel: w345 -> [w348 _]
          frame "Enabled" {
            n145 = shared-variable ".\\Setting Lib.lvlib\\settingthisVI"(error in=w348) -> (w352:refnum<vi>, error out=w351:errorcluster)
            n146 = invoke class="VI" method="FP.Open"(reference=w352, error in=w351, "Activate"=FALSE ("Activate?"), "State"=T16."Standard") -> (error out=w353:errorcluster)  [unwired: 1 in, 4 out]
            n147 = shared-variable ".\\Maintenance.lvlib\\error_61"(w353) -> ()  [unwired: 1 in, 1 out]
          }
          frame "Disabled", Default {
          }
        }
      }
      event "View", "Live 01", "Live 02", "Live 03", "Live 04", "Live 05", "Live 06": Mouse Down {
        n148 = event-data() -> ("CtlRef"=w356:refnum<vi>)  [unwired: 1 in, 7 out]
        n149 = property class="Bool (strict)"(reference=w356) -> (error out=w357:errorcluster, "Label.Text"=w358:string)  [unwired: 1 in, 1 out]
        n150 = case shown="\"Live 06\"" w358 {
          tunnel: w357 -> [w361 w370 w372 w378 w384 w390 w397]
          tunnel: [w359 w365 w371 w377 w383 w389 w398] -> w355
          frame "Live 01", Default {
            n151 = shared-variable ".\\D01.lvlib\\D01thisVI"(error in=w361) -> (w364:refnum<vi>, error out=w360:errorcluster)
            n152 = invoke class="VI" method="FP.Open"(reference=w364, error in=w360, "Activate"=FALSE ("Activate?"), "State"=T16."Standard") -> (error out=w359:errorcluster)  [unwired: 1 in, 4 out]
          }
          frame "Live 02" {
            n153 = shared-variable ".\\D02.lvlib\\D02thisVI"(error in=w370) -> (w369:refnum<vi>, error out=w368:errorcluster)
            n154 = invoke class="VI" method="FP.Open"(reference=w369, error in=w368, "Activate"=TRUE ("Activate?"), "State"=T16."Standard") -> (error out=w365:errorcluster)  [unwired: 1 in, 4 out]
          }
          frame "Live 03" {
            n155 = shared-variable ".\\D03.lvlib\\D03thisVI"(error in=w372) -> (w374:refnum<vi>, error out=w373:errorcluster)
            n156 = invoke class="VI" method="FP.Open"(reference=w374, error in=w373, "Activate"=TRUE ("Activate?"), "State"=T16."Standard") -> (error out=w371:errorcluster)  [unwired: 1 in, 4 out]
          }
          frame "Live 04" {
            n157 = shared-variable ".\\D04.lvlib\\D04thisVI"(error in=w378) -> (w380:refnum<vi>, error out=w379:errorcluster)
            n158 = invoke class="VI" method="FP.Open"(reference=w380, error in=w379, "Activate"=TRUE ("Activate?"), "State"=T16."Standard") -> (error out=w377:errorcluster)  [unwired: 1 in, 4 out]
          }
          frame "Live 05" {
            n159 = shared-variable ".\\D05.lvlib\\D05thisVI"(error in=w384) -> (w388:refnum<vi>, error out=w387:errorcluster)
            n160 = invoke class="VI" method="FP.Open"(reference=w388, error in=w387, "Activate"=TRUE ("Activate?"), "State"=T16."Standard") -> (error out=w383:errorcluster)  [unwired: 1 in, 4 out]
          }
          frame "Live 06" {
            n161 = shared-variable ".\\D06.lvlib\\D06thisVI"(error in=w390) -> (w394:refnum<vi>, error out=w393:errorcluster)
            n162 = invoke class="VI" method="FP.Open"(reference=w394, error in=w393, "Activate"=TRUE ("Activate?"), "State"=T16."Standard") -> (error out=w389:errorcluster)  [unwired: 1 in, 4 out]
          }
          frame "View" {
            n163 = shared-variable ".\\detectedPellet.lvlib\\open flag"(TRUE ("open flag"), error in=w397) -> (error out=w396:errorcluster)
            n164 = shared-variable ".\\detectedPellet.lvlib\\DetectedPelletThisVi"(error in=w396) -> (w399:refnum<vi>, error out=w400:errorcluster)
            n165 = invoke class="VI" method="FP.Open"(reference=w399, error in=w400, "Activate"=TRUE ("Activate?"), "State"=T16."Standard") -> (error out=w398:errorcluster)  [unwired: 1 in, 4 out]
          }
        }
        n166 = shared-variable ".\\Maintenance.lvlib\\error_62"(w355) -> ()  [unwired: 1 in, 1 out]
      }
      event "Info 01", "Info 02", "Info 03", "Info 04", "Info 05", "Info 06": Mouse Down {
        n167 = event-data() -> ("CtlRef"=w405:refnum<vi>)  [unwired: 1 in, 7 out]
        n168 = property class="Bool (strict)"(reference=w405) -> ("Label.Text"=w404:string)  [unwired: 1 in, 2 out]
        n169 = case shown="\"Info 01\", Default" w404 {
          frame "Info 01", Default {
            n170 = call "camera info.vi"("Disc Number"="Disc 01", "Camera Name"=T17 "cam0" ("Session In")) -> ()  [unwired: 10 in]
          }
          frame "Info 02" {
            n171 = call "camera info.vi"("Disc Number"="Disc 02", "Camera Name"=T17 "cam1" ("Session In")) -> ()  [unwired: 10 in]
          }
          frame "Info 03" {
            n172 = call "camera info.vi"("Disc Number"="Disc 03", "Camera Name"=T17 "cam2" ("Session In")) -> ()  [unwired: 10 in]
          }
          frame "Info 04" {
            n173 = call "camera info.vi"("Disc Number"="Disc 04", "Camera Name"=T17 "cam3" ("Session In")) -> ()  [unwired: 10 in]
          }
          frame "Info 05" {
            n174 = call "camera info.vi"("Disc Number"="Disc 05", "Camera Name"=T17 "cam4" ("Session In")) -> ()  [unwired: 10 in]
          }
          frame "Info 06" {
            n175 = call "camera info.vi"("Disc Number"="Disc 06", "Camera Name"=T17 "cam5" ("Session In")) -> ()  [unwired: 10 in]
          }
        }
      }
      event "Warning 01", "Warning 02", "Warning 03", "Warning 04", "Warning 05", "Warning 06": Mouse Down {
        n176 = event-data() -> ("CtlRef"=w421:refnum<vi>)  [unwired: 1 in, 7 out]
        n177 = property class="Bool (strict)"(reference=w421) -> (error out=w419:errorcluster, "Label.Text"=w420:string)  [unwired: 1 in, 1 out]
        n178 = case shown="\"Warning 06\"" w420 {
          tunnel: w419 -> [w422 w457 w492 w527 w562 w598]
          frame "Warning 01", Default {
            n179 = property on="Warning array 01" class="Arr (strict)"(error in=w422) -> ("Value"=w424:bool[])  [unwired: 1 in, 2 out]
            n180 = Boolean Array To Number(Boolean array=w424) -> (number=w423:u32)
            n181 = case shown="15" w423 {
              frame 0, Default {
              }
              frame 1 {
                n182 = One Button Dialog(message="Warning1: Camera of disc 1 is off.") -> ()  [unwired: 1 in, 1 out]
              }
              frame 2 {
                n183 = One Button Dialog(message="Warning2: Projector of disc 1 is off.") -> ()  [unwired: 1 in, 1 out]
              }
              frame 3 {
                n184 = flat-sequence {
                  frame #0 {
                    n185 = One Button Dialog(message="Warning1: Camera of disc 1 is off.") -> ()  [unwired: 1 in, 1 out]
                  }
                  frame #1 {
                    n186 = One Button Dialog(message="Warning2: Projector of disc 1 is off.") -> ()  [unwired: 1 in, 1 out]
                  }
                }
              }
              frame 4 {
                n187 = One Button Dialog(message="Warning3: control mode of disc 1 is manual.") -> ()  [unwired: 1 in, 1 out]
              }
              frame 5 {
                n188 = flat-sequence {
                  frame #0 {
                    n189 = One Button Dialog(message="Warning1: Camera of disc 1 is off.") -> ()  [unwired: 1 in, 1 out]
                  }
                  frame #1 {
                    n190 = One Button Dialog(message="Warning3: Control mode of disc 1 is manual.") -> ()  [unwired: 1 in, 1 out]
                  }
                }
              }
              frame 6 {
                n191 = flat-sequence {
                  frame #0 {
                    n192 = One Button Dialog(message="Warning2: Projector of disc 1 is off.") -> ()  [unwired: 1 in, 1 out]
                  }
                  frame #1 {
                    n193 = One Button Dialog(message="Warning3: Control mode of disc 1 is manual.") -> ()  [unwired: 1 in, 1 out]
                  }
                }
              }
              frame 7 {
                n194 = flat-sequence {
                  frame #0 {
                    n195 = One Button Dialog(message="Warning1: Camera of disc 1 is off.") -> ()  [unwired: 1 in, 1 out]
                  }
                  frame #1 {
                    n196 = One Button Dialog(message="Warning2: Projector of disc 1 is off.") -> ()  [unwired: 1 in, 1 out]
                  }
                  frame #2 {
                    n197 = One Button Dialog(message="Warning3: Control mode of disc 1 is manual.") -> ()  [unwired: 1 in, 1 out]
                  }
                }
              }
              frame 8 {
                n198 = One Button Dialog(message="Warning4: Disc 1 is stop.") -> ()  [unwired: 1 in, 1 out]
              }
              frame 9 {
                n199 = flat-sequence {
                  frame #0 {
                    n200 = One Button Dialog(message="Warning1: Camera of disc 1 is off.") -> ()  [unwired: 1 in, 1 out]
                  }
                  frame #1 {
                    n201 = One Button Dialog(message="Warning4: Disc 1 is stop.") -> ()  [unwired: 1 in, 1 out]
                  }
                }
              }
              frame 10 {
                n202 = flat-sequence {
                  frame #0 {
                    n203 = One Button Dialog(message="Warning2: Projector of disc 1 is off.") -> ()  [unwired: 1 in, 1 out]
                  }
                  frame #1 {
                    n204 = One Button Dialog(message="Warning4: Disc 1 is stop.") -> ()  [unwired: 1 in, 1 out]
                  }
                }
              }
              frame 11 {
                n205 = flat-sequence {
                  frame #0 {
                    n206 = One Button Dialog(message="Warning1: Camera of disc 1 is off.") -> ()  [unwired: 1 in, 1 out]
                  }
                  frame #1 {
                    n207 = One Button Dialog(message="Warning2: Projector of disc 1 is off.") -> ()  [unwired: 1 in, 1 out]
                  }
                  frame #2 {
                    n208 = One Button Dialog(message="Warning4: Disc 1 is stop.") -> ()  [unwired: 1 in, 1 out]
                  }
                }
              }
              frame 12 {
                n209 = flat-sequence {
                  frame #0 {
                    n210 = One Button Dialog(message="Warning3: control mode of disc 1 is manual.") -> ()  [unwired: 1 in, 1 out]
                  }
                  frame #1 {
                    n211 = One Button Dialog(message="Warning4: Disc 1 is stop.") -> ()  [unwired: 1 in, 1 out]
                  }
                }
              }
              frame 13 {
                n212 = flat-sequence {
                  frame #0 {
                    n213 = One Button Dialog(message="Warning1: Camera of disc 1 is off.") -> ()  [unwired: 1 in, 1 out]
                  }
                  frame #1 {
                    n214 = One Button Dialog(message="Warning3: control mode of disc 1 is manual.") -> ()  [unwired: 1 in, 1 out]
                  }
                  frame #2 {
                    n215 = One Button Dialog(message="Warning4: Disc 1 is stop.") -> ()  [unwired: 1 in, 1 out]
                  }
                }
              }
              frame 14 {
                n216 = flat-sequence {
                  frame #0 {
                    n217 = One Button Dialog(message="Warning2: Projector of disc 1 is off.") -> ()  [unwired: 1 in, 1 out]
                  }
                  frame #1 {
                    n218 = One Button Dialog(message="Warning3: control mode of disc 1 is manual.") -> ()  [unwired: 1 in, 1 out]
                  }
                  frame #2 {
                    n219 = One Button Dialog(message="Warning4: Disc 1 is stop.") -> ()  [unwired: 1 in, 1 out]
                  }
                }
              }
              frame 15 {
                n220 = flat-sequence {
                  frame #0 {
                    n221 = One Button Dialog(message="Warning1: Camera of disc 1 is off.") -> ()  [unwired: 1 in, 1 out]
                  }
                  frame #1 {
                    n222 = One Button Dialog(message="Warning2: Projector of disc 1 is off.") -> ()  [unwired: 1 in, 1 out]
                  }
                  frame #2 {
                    n223 = One Button Dialog(message="Warning3: control mode of disc 1 is manual.") -> ()  [unwired: 1 in, 1 out]
                  }
                  frame #3 {
                    n224 = One Button Dialog(message="Warning4: Disc 1 is stop.") -> ()  [unwired: 1 in, 1 out]
                  }
                }
              }
            }
          }
          frame "Warning 02" {
            n225 = property on="Warning array 02" class="Arr (strict)"(error in=w457) -> ("Value"=w459:bool[])  [unwired: 1 in, 2 out]
            n226 = Boolean Array To Number(Boolean array=w459) -> (number=w458:u32)
            n227 = case shown="0, Default" w458 {
              frame 0, Default {
              }
              frame 1 {
                n228 = One Button Dialog(message="Warning1: Camera of disc 2 is off.") -> ()  [unwired: 1 in, 1 out]
              }
              frame 2 {
                n229 = One Button Dialog(message="Warning2: Projector of disc 2 is off.") -> ()  [unwired: 1 in, 1 out]
              }
              frame 3 {
                n230 = flat-sequence {
                  frame #0 {
                    n231 = One Button Dialog(message="Warning1: Camera of disc 2 is off.") -> ()  [unwired: 1 in, 1 out]
                  }
                  frame #1 {
                    n232 = One Button Dialog(message="Warning2: Projector of disc 2 is off.") -> ()  [unwired: 1 in, 1 out]
                  }
                }
              }
              frame 4 {
                n233 = One Button Dialog(message="Warning3: control mode of disc 2 is manual.") -> ()  [unwired: 1 in, 1 out]
              }
              frame 5 {
                n234 = flat-sequence {
                  frame #0 {
                    n235 = One Button Dialog(message="Warning1: Camera of disc 2 is off.") -> ()  [unwired: 1 in, 1 out]
                  }
                  frame #1 {
                    n236 = One Button Dialog(message="Warning3: Control mode of disc 2 is manual.") -> ()  [unwired: 1 in, 1 out]
                  }
                }
              }
              frame 6 {
                n237 = flat-sequence {
                  frame #0 {
                    n238 = One Button Dialog(message="Warning2: Projector of disc 2 is off.") -> ()  [unwired: 1 in, 1 out]
                  }
                  frame #1 {
                    n239 = One Button Dialog(message="Warning3: Control mode of disc 2 is manual.") -> ()  [unwired: 1 in, 1 out]
                  }
                }
              }
              frame 7 {
                n240 = flat-sequence {
                  frame #0 {
                    n241 = One Button Dialog(message="Warning1: Camera of disc 2 is off.") -> ()  [unwired: 1 in, 1 out]
                  }
                  frame #1 {
                    n242 = One Button Dialog(message="Warning2: Projector of disc 2 is off.") -> ()  [unwired: 1 in, 1 out]
                  }
                  frame #2 {
                    n243 = One Button Dialog(message="Warning3: Control mode of disc 2 is manual.") -> ()  [unwired: 1 in, 1 out]
                  }
                }
              }
              frame 8 {
                n244 = One Button Dialog(message="Warning4: Disc 2 is stop.") -> ()  [unwired: 1 in, 1 out]
              }
              frame 9 {
                n245 = flat-sequence {
                  frame #0 {
                    n246 = One Button Dialog(message="Warning1: Camera of disc 2 is off.") -> ()  [unwired: 1 in, 1 out]
                  }
                  frame #1 {
                    n247 = One Button Dialog(message="Warning4: Disc 2 is stop.") -> ()  [unwired: 1 in, 1 out]
                  }
                }
              }
              frame 10 {
                n248 = flat-sequence {
                  frame #0 {
                    n249 = One Button Dialog(message="Warning2: Projector of disc 2 is off.") -> ()  [unwired: 1 in, 1 out]
                  }
                  frame #1 {
                    n250 = One Button Dialog(message="Warning4: Disc 2 is stop.") -> ()  [unwired: 1 in, 1 out]
                  }
                }
              }
              frame 11 {
                n251 = flat-sequence {
                  frame #0 {
                    n252 = One Button Dialog(message="Warning1: Camera of disc 2 is off.") -> ()  [unwired: 1 in, 1 out]
                  }
                  frame #1 {
                    n253 = One Button Dialog(message="Warning2: Projector of disc 2 is off.") -> ()  [unwired: 1 in, 1 out]
                  }
                  frame #2 {
                    n254 = One Button Dialog(message="Warning4: Disc 2 is stop.") -> ()  [unwired: 1 in, 1 out]
                  }
                }
              }
              frame 12 {
                n255 = flat-sequence {
                  frame #0 {
                    n256 = One Button Dialog(message="Warning3: control mode of disc 2 is manual.") -> ()  [unwired: 1 in, 1 out]
                  }
                  frame #1 {
                    n257 = One Button Dialog(message="Warning4: Disc 2 is stop.") -> ()  [unwired: 1 in, 1 out]
                  }
                }
              }
              frame 13 {
                n258 = flat-sequence {
                  frame #0 {
                    n259 = One Button Dialog(message="Warning1: Camera of disc 2 is off.") -> ()  [unwired: 1 in, 1 out]
                  }
                  frame #1 {
                    n260 = One Button Dialog(message="Warning3: control mode of disc 2 is manual.") -> ()  [unwired: 1 in, 1 out]
                  }
                  frame #2 {
                    n261 = One Button Dialog(message="Warning4: Disc 2 is stop.") -> ()  [unwired: 1 in, 1 out]
                  }
                }
              }
              frame 14 {
                n262 = flat-sequence {
                  frame #0 {
                    n263 = One Button Dialog(message="Warning2: Projector of disc 2 is off.") -> ()  [unwired: 1 in, 1 out]
                  }
                  frame #1 {
                    n264 = One Button Dialog(message="Warning3: control mode of disc 2 is manual.") -> ()  [unwired: 1 in, 1 out]
                  }
                  frame #2 {
                    n265 = One Button Dialog(message="Warning4: Disc 2 is stop.") -> ()  [unwired: 1 in, 1 out]
                  }
                }
              }
              frame 15 {
                n266 = flat-sequence {
                  frame #0 {
                    n267 = One Button Dialog(message="Warning1: Camera of disc 2 is off.") -> ()  [unwired: 1 in, 1 out]
                  }
                  frame #1 {
                    n268 = One Button Dialog(message="Warning2: Projector of disc 2 is off.") -> ()  [unwired: 1 in, 1 out]
                  }
                  frame #2 {
                    n269 = One Button Dialog(message="Warning3: control mode of disc 2 is manual.") -> ()  [unwired: 1 in, 1 out]
                  }
                  frame #3 {
                    n270 = One Button Dialog(message="Warning4: Disc 2 is stop.") -> ()  [unwired: 1 in, 1 out]
                  }
                }
              }
            }
          }
          frame "Warning 03" {
            n271 = property on="Warning array 03" class="Arr (strict)"(error in=w492) -> ("Value"=w494:bool[])  [unwired: 1 in, 2 out]
            n272 = Boolean Array To Number(Boolean array=w494) -> (number=w493:u32)
            n273 = case shown="0, Default" w493 {
              frame 0, Default {
              }
              frame 1 {
                n274 = One Button Dialog(message="Warning1: Camera of disc 3 is off.") -> ()  [unwired: 1 in, 1 out]
              }
              frame 2 {
                n275 = One Button Dialog(message="Warning2: Projector of disc 3 is off.") -> ()  [unwired: 1 in, 1 out]
              }
              frame 3 {
                n276 = flat-sequence {
                  frame #0 {
                    n277 = One Button Dialog(message="Warning1: Camera of disc 3 is off.") -> ()  [unwired: 1 in, 1 out]
                  }
                  frame #1 {
                    n278 = One Button Dialog(message="Warning2: Projector of disc 3 is off.") -> ()  [unwired: 1 in, 1 out]
                  }
                }
              }
              frame 4 {
                n279 = One Button Dialog(message="Warning3: control mode of disc 3 is manual.") -> ()  [unwired: 1 in, 1 out]
              }
              frame 5 {
                n280 = flat-sequence {
                  frame #0 {
                    n281 = One Button Dialog(message="Warning1: Camera of disc 3 is off.") -> ()  [unwired: 1 in, 1 out]
                  }
                  frame #1 {
                    n282 = One Button Dialog(message="Warning3: Control mode of disc 3 is manual.") -> ()  [unwired: 1 in, 1 out]
                  }
                }
              }
              frame 6 {
                n283 = flat-sequence {
                  frame #0 {
                    n284 = One Button Dialog(message="Warning2: Projector of disc 3 is off.") -> ()  [unwired: 1 in, 1 out]
                  }
                  frame #1 {
                    n285 = One Button Dialog(message="Warning3: Control mode of disc 3 is manual.") -> ()  [unwired: 1 in, 1 out]
                  }
                }
              }
              frame 7 {
                n286 = flat-sequence {
                  frame #0 {
                    n287 = One Button Dialog(message="Warning1: Camera of disc 3 is off.") -> ()  [unwired: 1 in, 1 out]
                  }
                  frame #1 {
                    n288 = One Button Dialog(message="Warning2: Projector of disc 3 is off.") -> ()  [unwired: 1 in, 1 out]
                  }
                  frame #2 {
                    n289 = One Button Dialog(message="Warning3: Control mode of disc 3 is manual.") -> ()  [unwired: 1 in, 1 out]
                  }
                }
              }
              frame 8 {
                n290 = One Button Dialog(message="Warning4: Disc 3 is stop.") -> ()  [unwired: 1 in, 1 out]
              }
              frame 9 {
                n291 = flat-sequence {
                  frame #0 {
                    n292 = One Button Dialog(message="Warning1: Camera of disc 3 is off.") -> ()  [unwired: 1 in, 1 out]
                  }
                  frame #1 {
                    n293 = One Button Dialog(message="Warning4: Disc 3 is stop.") -> ()  [unwired: 1 in, 1 out]
                  }
                }
              }
              frame 10 {
                n294 = flat-sequence {
                  frame #0 {
                    n295 = One Button Dialog(message="Warning2: Projector of disc 3 is off.") -> ()  [unwired: 1 in, 1 out]
                  }
                  frame #1 {
                    n296 = One Button Dialog(message="Warning4: Disc 3 is stop.") -> ()  [unwired: 1 in, 1 out]
                  }
                }
              }
              frame 11 {
                n297 = flat-sequence {
                  frame #0 {
                    n298 = One Button Dialog(message="Warning1: Camera of disc 3 is off.") -> ()  [unwired: 1 in, 1 out]
                  }
                  frame #1 {
                    n299 = One Button Dialog(message="Warning2: Projector of disc 3 is off.") -> ()  [unwired: 1 in, 1 out]
                  }
                  frame #2 {
                    n300 = One Button Dialog(message="Warning4: Disc 3 is stop.") -> ()  [unwired: 1 in, 1 out]
                  }
                }
              }
              frame 12 {
                n301 = flat-sequence {
                  frame #0 {
                    n302 = One Button Dialog(message="Warning3: control mode of disc 3 is manual.") -> ()  [unwired: 1 in, 1 out]
                  }
                  frame #1 {
                    n303 = One Button Dialog(message="Warning4: Disc 3 is stop.") -> ()  [unwired: 1 in, 1 out]
                  }
                }
              }
              frame 13 {
                n304 = flat-sequence {
                  frame #0 {
                    n305 = One Button Dialog(message="Warning1: Camera of disc 3 is off.") -> ()  [unwired: 1 in, 1 out]
                  }
                  frame #1 {
                    n306 = One Button Dialog(message="Warning3: control mode of disc 3 is manual.") -> ()  [unwired: 1 in, 1 out]
                  }
                  frame #2 {
                    n307 = One Button Dialog(message="Warning4: Disc 3 is stop.") -> ()  [unwired: 1 in, 1 out]
                  }
                }
              }
              frame 14 {
                n308 = flat-sequence {
                  frame #0 {
                    n309 = One Button Dialog(message="Warning2: Projector of disc 3 is off.") -> ()  [unwired: 1 in, 1 out]
                  }
                  frame #1 {
                    n310 = One Button Dialog(message="Warning3: control mode of disc 3 is manual.") -> ()  [unwired: 1 in, 1 out]
                  }
                  frame #2 {
                    n311 = One Button Dialog(message="Warning4: Disc 3 is stop.") -> ()  [unwired: 1 in, 1 out]
                  }
                }
              }
              frame 15 {
                n312 = flat-sequence {
                  frame #0 {
                    n313 = One Button Dialog(message="Warning1: Camera of disc 3 is off.") -> ()  [unwired: 1 in, 1 out]
                  }
                  frame #1 {
                    n314 = One Button Dialog(message="Warning2: Projector of disc 3 is off.") -> ()  [unwired: 1 in, 1 out]
                  }
                  frame #2 {
                    n315 = One Button Dialog(message="Warning3: control mode of disc 3 is manual.") -> ()  [unwired: 1 in, 1 out]
                  }
                  frame #3 {
                    n316 = One Button Dialog(message="Warning4: Disc 3 is stop.") -> ()  [unwired: 1 in, 1 out]
                  }
                }
              }
            }
          }
          frame "Warning 04" {
            n317 = property on="Warning array 04" class="Arr (strict)"(error in=w527) -> ("Value"=w529:bool[])  [unwired: 1 in, 2 out]
            n318 = Boolean Array To Number(Boolean array=w529) -> (number=w528:u32)
            n319 = case shown="15" w528 {
              frame 0, Default {
              }
              frame 1 {
                n320 = One Button Dialog(message="Warning1: Camera of disc 4 is off.") -> ()  [unwired: 1 in, 1 out]
              }
              frame 2 {
                n321 = One Button Dialog(message="Warning2: Projector of disc 4 is off.") -> ()  [unwired: 1 in, 1 out]
              }
              frame 3 {
                n322 = flat-sequence {
                  frame #0 {
                    n323 = One Button Dialog(message="Warning1: Camera of disc 4 is off.") -> ()  [unwired: 1 in, 1 out]
                  }
                  frame #1 {
                    n324 = One Button Dialog(message="Warning2: Projector of disc 4 is off.") -> ()  [unwired: 1 in, 1 out]
                  }
                }
              }
              frame 4 {
                n325 = One Button Dialog(message="Warning3: control mode of disc 4 is manual.") -> ()  [unwired: 1 in, 1 out]
              }
              frame 5 {
                n326 = flat-sequence {
                  frame #0 {
                    n327 = One Button Dialog(message="Warning1: Camera of disc 4 is off.") -> ()  [unwired: 1 in, 1 out]
                  }
                  frame #1 {
                    n328 = One Button Dialog(message="Warning3: Control mode of disc 4 is manual.") -> ()  [unwired: 1 in, 1 out]
                  }
                }
              }
              frame 6 {
                n329 = flat-sequence {
                  frame #0 {
                    n330 = One Button Dialog(message="Warning2: Projector of disc 4 is off.") -> ()  [unwired: 1 in, 1 out]
                  }
                  frame #1 {
                    n331 = One Button Dialog(message="Warning3: Control mode of disc 4 is manual.") -> ()  [unwired: 1 in, 1 out]
                  }
                }
              }
              frame 7 {
                n332 = flat-sequence {
                  frame #0 {
                    n333 = One Button Dialog(message="Warning1: Camera of disc 4 is off.") -> ()  [unwired: 1 in, 1 out]
                  }
                  frame #1 {
                    n334 = One Button Dialog(message="Warning2: Projector of disc 4 is off.") -> ()  [unwired: 1 in, 1 out]
                  }
                  frame #2 {
                    n335 = One Button Dialog(message="Warning3: Control mode of disc 4 is manual.") -> ()  [unwired: 1 in, 1 out]
                  }
                }
              }
              frame 8 {
                n336 = One Button Dialog(message="Warning4: Disc 4 is stop.") -> ()  [unwired: 1 in, 1 out]
              }
              frame 9 {
                n337 = flat-sequence {
                  frame #0 {
                    n338 = One Button Dialog(message="Warning1: Camera of disc 4 is off.") -> ()  [unwired: 1 in, 1 out]
                  }
                  frame #1 {
                    n339 = One Button Dialog(message="Warning4: Disc 4 is stop.") -> ()  [unwired: 1 in, 1 out]
                  }
                }
              }
              frame 10 {
                n340 = flat-sequence {
                  frame #0 {
                    n341 = One Button Dialog(message="Warning2: Projector of disc 4 is off.") -> ()  [unwired: 1 in, 1 out]
                  }
                  frame #1 {
                    n342 = One Button Dialog(message="Warning4: Disc 4 is stop.") -> ()  [unwired: 1 in, 1 out]
                  }
                }
              }
              frame 11 {
                n343 = flat-sequence {
                  frame #0 {
                    n344 = One Button Dialog(message="Warning1: Camera of disc 4 is off.") -> ()  [unwired: 1 in, 1 out]
                  }
                  frame #1 {
                    n345 = One Button Dialog(message="Warning2: Projector of disc 4 is off.") -> ()  [unwired: 1 in, 1 out]
                  }
                  frame #2 {
                    n346 = One Button Dialog(message="Warning4: Disc 4 is stop.") -> ()  [unwired: 1 in, 1 out]
                  }
                }
              }
              frame 12 {
                n347 = flat-sequence {
                  frame #0 {
                    n348 = One Button Dialog(message="Warning3: control mode of disc 4 is manual.") -> ()  [unwired: 1 in, 1 out]
                  }
                  frame #1 {
                    n349 = One Button Dialog(message="Warning4: Disc 4 is stop.") -> ()  [unwired: 1 in, 1 out]
                  }
                }
              }
              frame 13 {
                n350 = flat-sequence {
                  frame #0 {
                    n351 = One Button Dialog(message="Warning1: Camera of disc 4 is off.") -> ()  [unwired: 1 in, 1 out]
                  }
                  frame #1 {
                    n352 = One Button Dialog(message="Warning3: control mode of disc 4 is manual.") -> ()  [unwired: 1 in, 1 out]
                  }
                  frame #2 {
                    n353 = One Button Dialog(message="Warning4: Disc 4 is stop.") -> ()  [unwired: 1 in, 1 out]
                  }
                }
              }
              frame 14 {
                n354 = flat-sequence {
                  frame #0 {
                    n355 = One Button Dialog(message="Warning2: Projector of disc 4 is off.") -> ()  [unwired: 1 in, 1 out]
                  }
                  frame #1 {
                    n356 = One Button Dialog(message="Warning3: control mode of disc 4 is manual.") -> ()  [unwired: 1 in, 1 out]
                  }
                  frame #2 {
                    n357 = One Button Dialog(message="Warning4: Disc 4 is stop.") -> ()  [unwired: 1 in, 1 out]
                  }
                }
              }
              frame 15 {
                n358 = flat-sequence {
                  frame #0 {
                    n359 = One Button Dialog(message="Warning1: Camera of disc 4 is off.") -> ()  [unwired: 1 in, 1 out]
                  }
                  frame #1 {
                    n360 = One Button Dialog(message="Warning2: Projector of disc 4 is off.") -> ()  [unwired: 1 in, 1 out]
                  }
                  frame #2 {
                    n361 = One Button Dialog(message="Warning3: control mode of disc 4 is manual.") -> ()  [unwired: 1 in, 1 out]
                  }
                  frame #3 {
                    n362 = One Button Dialog(message="Warning4: Disc 4 is stop.") -> ()  [unwired: 1 in, 1 out]
                  }
                }
              }
            }
          }
          frame "Warning 05" {
            n363 = property on="Warning array 05" class="Arr (strict)"(error in=w562) -> ("Value"=w564:bool[])  [unwired: 1 in, 2 out]
            n364 = Boolean Array To Number(Boolean array=w564) -> (number=w563:u32)
            n365 = case shown="15" w563 {
              frame 0, Default {
              }
              frame 1 {
                n366 = One Button Dialog(message="Warning1: Camera of disc 5 is off.") -> ()  [unwired: 1 in, 1 out]
              }
              frame 2 {
                n367 = One Button Dialog(message="Warning2: Projector of disc 5 is off.") -> ()  [unwired: 1 in, 1 out]
              }
              frame 3 {
                n368 = flat-sequence {
                  frame #0 {
                    n369 = One Button Dialog(message="Warning1: Camera of disc 5 is off.") -> ()  [unwired: 1 in, 1 out]
                  }
                  frame #1 {
                    n370 = One Button Dialog(message="Warning2: Projector of disc 5 is off.") -> ()  [unwired: 1 in, 1 out]
                  }
                }
              }
              frame 4 {
                n371 = One Button Dialog(message="Warning3: control mode of disc 5 is manual.") -> ()  [unwired: 1 in, 1 out]
              }
              frame 5 {
                n372 = flat-sequence {
                  frame #0 {
                    n373 = One Button Dialog(message="Warning1: Camera of disc 5 is off.") -> ()  [unwired: 1 in, 1 out]
                  }
                  frame #1 {
                    n374 = One Button Dialog(message="Warning3: Control mode of disc 5 is manual.") -> ()  [unwired: 1 in, 1 out]
                  }
                }
              }
              frame 6 {
                n375 = flat-sequence {
                  frame #0 {
                    n376 = One Button Dialog(message="Warning2: Projector of disc 5 is off.") -> ()  [unwired: 1 in, 1 out]
                  }
                  frame #1 {
                    n377 = One Button Dialog(message="Warning3: Control mode of disc 5 is manual.") -> ()  [unwired: 1 in, 1 out]
                  }
                }
              }
              frame 7 {
                n378 = flat-sequence {
                  frame #0 {
                    n379 = One Button Dialog(message="Warning1: Camera of disc 5 is off.") -> ()  [unwired: 1 in, 1 out]
                  }
                  frame #1 {
                    n380 = One Button Dialog(message="Warning2: Projector of disc 5 is off.") -> ()  [unwired: 1 in, 1 out]
                  }
                  frame #2 {
                    n381 = One Button Dialog(message="Warning3: Control mode of disc 5 is manual.") -> ()  [unwired: 1 in, 1 out]
                  }
                }
              }
              frame 8 {
                n382 = One Button Dialog(message="Warning4: Disc 5 is stop.") -> ()  [unwired: 1 in, 1 out]
              }
              frame 9 {
                n383 = flat-sequence {
                  frame #0 {
                    n384 = One Button Dialog(message="Warning1: Camera of disc 5 is off.") -> ()  [unwired: 1 in, 1 out]
                  }
                  frame #1 {
                    n385 = One Button Dialog(message="Warning4: Disc 5 is stop.") -> ()  [unwired: 1 in, 1 out]
                  }
                }
              }
              frame 10 {
                n386 = flat-sequence {
                  frame #0 {
                    n387 = One Button Dialog(message="Warning2: Projector of disc 5 is off.") -> ()  [unwired: 1 in, 1 out]
                  }
                  frame #1 {
                    n388 = One Button Dialog(message="Warning4: Disc 5 is stop.") -> ()  [unwired: 1 in, 1 out]
                  }
                }
              }
              frame 11 {
                n389 = flat-sequence {
                  frame #0 {
                    n390 = One Button Dialog(message="Warning1: Camera of disc 5 is off.") -> ()  [unwired: 1 in, 1 out]
                  }
                  frame #1 {
                    n391 = One Button Dialog(message="Warning2: Projector of disc 5 is off.") -> ()  [unwired: 1 in, 1 out]
                  }
                  frame #2 {
                    n392 = One Button Dialog(message="Warning4: Disc 5 is stop.") -> ()  [unwired: 1 in, 1 out]
                  }
                }
              }
              frame 12 {
                n393 = flat-sequence {
                  frame #0 {
                    n394 = One Button Dialog(message="Warning3: control mode of disc 5 is manual.") -> ()  [unwired: 1 in, 1 out]
                  }
                  frame #1 {
                    n395 = One Button Dialog(message="Warning4: Disc 5 is stop.") -> ()  [unwired: 1 in, 1 out]
                  }
                }
              }
              frame 13 {
                n396 = flat-sequence {
                  frame #0 {
                    n397 = One Button Dialog(message="Warning1: Camera of disc 5 is off.") -> ()  [unwired: 1 in, 1 out]
                  }
                  frame #1 {
                    n398 = One Button Dialog(message="Warning3: control mode of disc 5 is manual.") -> ()  [unwired: 1 in, 1 out]
                  }
                  frame #2 {
                    n399 = One Button Dialog(message="Warning4: Disc 5 is stop.") -> ()  [unwired: 1 in, 1 out]
                  }
                }
              }
              frame 14 {
                n400 = flat-sequence {
                  frame #0 {
                    n401 = One Button Dialog(message="Warning2: Projector of disc 5 is off.") -> ()  [unwired: 1 in, 1 out]
                  }
                  frame #1 {
                    n402 = One Button Dialog(message="Warning3: control mode of disc 5 is manual.") -> ()  [unwired: 1 in, 1 out]
                  }
                  frame #2 {
                    n403 = One Button Dialog(message="Warning4: Disc 5 is stop.") -> ()  [unwired: 1 in, 1 out]
                  }
                }
              }
              frame 15 {
                n404 = flat-sequence {
                  frame #0 {
                    n405 = One Button Dialog(message="Warning1: Camera of disc 5 is off.") -> ()  [unwired: 1 in, 1 out]
                  }
                  frame #1 {
                    n406 = One Button Dialog(message="Warning2: Projector of disc 5 is off.") -> ()  [unwired: 1 in, 1 out]
                  }
                  frame #2 {
                    n407 = One Button Dialog(message="Warning3: control mode of disc 5 is manual.") -> ()  [unwired: 1 in, 1 out]
                  }
                  frame #3 {
                    n408 = One Button Dialog(message="Warning4: Disc 5 is stop.") -> ()  [unwired: 1 in, 1 out]
                  }
                }
              }
            }
          }
          frame "Warning 06" {
            n409 = property on="Warning array 06" class="Arr (strict)"(error in=w598) -> ("Value"=w599:bool[])  [unwired: 1 in, 2 out]
            n410 = Boolean Array To Number(Boolean array=w599) -> (number=w597:u32)
            n411 = case shown="15" w597 {
              frame 0, Default {
              }
              frame 1 {
                n412 = One Button Dialog(message="Warning1: Camera of disc 6 is off.") -> ()  [unwired: 1 in, 1 out]
              }
              frame 2 {
                n413 = One Button Dialog(message="Warning2: Projector of disc 6 is off.") -> ()  [unwired: 1 in, 1 out]
              }
              frame 3 {
                n414 = flat-sequence {
                  frame #0 {
                    n415 = One Button Dialog(message="Warning1: Camera of disc 6 is off.") -> ()  [unwired: 1 in, 1 out]
                  }
                  frame #1 {
                    n416 = One Button Dialog(message="Warning2: Projector of disc 6 is off.") -> ()  [unwired: 1 in, 1 out]
                  }
                }
              }
              frame 4 {
                n417 = One Button Dialog(message="Warning3: control mode of disc 6 is manual.") -> ()  [unwired: 1 in, 1 out]
              }
              frame 5 {
                n418 = flat-sequence {
                  frame #0 {
                    n419 = One Button Dialog(message="Warning1: Camera of disc 6 is off.") -> ()  [unwired: 1 in, 1 out]
                  }
                  frame #1 {
                    n420 = One Button Dialog(message="Warning3: Control mode of disc 6 is manual.") -> ()  [unwired: 1 in, 1 out]
                  }
                }
              }
              frame 6 {
                n421 = flat-sequence {
                  frame #0 {
                    n422 = One Button Dialog(message="Warning2: Projector of disc 6 is off.") -> ()  [unwired: 1 in, 1 out]
                  }
                  frame #1 {
                    n423 = One Button Dialog(message="Warning3: Control mode of disc 6 is manual.") -> ()  [unwired: 1 in, 1 out]
                  }
                }
              }
              frame 7 {
                n424 = flat-sequence {
                  frame #0 {
                    n425 = One Button Dialog(message="Warning1: Camera of disc 6 is off.") -> ()  [unwired: 1 in, 1 out]
                  }
                  frame #1 {
                    n426 = One Button Dialog(message="Warning2: Projector of disc 6 is off.") -> ()  [unwired: 1 in, 1 out]
                  }
                  frame #2 {
                    n427 = One Button Dialog(message="Warning3: Control mode of disc 6 is manual.") -> ()  [unwired: 1 in, 1 out]
                  }
                }
              }
              frame 8 {
                n428 = One Button Dialog(message="Warning4: Disc 6 is stop.") -> ()  [unwired: 1 in, 1 out]
              }
              frame 9 {
                n429 = flat-sequence {
                  frame #0 {
                    n430 = One Button Dialog(message="Warning1: Camera of disc 6 is off.") -> ()  [unwired: 1 in, 1 out]
                  }
                  frame #1 {
                    n431 = One Button Dialog(message="Warning4: Disc 6 is stop.") -> ()  [unwired: 1 in, 1 out]
                  }
                }
              }
              frame 10 {
                n432 = flat-sequence {
                  frame #0 {
                    n433 = One Button Dialog(message="Warning2: Projector of disc 6 is off.") -> ()  [unwired: 1 in, 1 out]
                  }
                  frame #1 {
                    n434 = One Button Dialog(message="Warning4: Disc 6 is stop.") -> ()  [unwired: 1 in, 1 out]
                  }
                }
              }
              frame 11 {
                n435 = flat-sequence {
                  frame #0 {
                    n436 = One Button Dialog(message="Warning1: Camera of disc 6 is off.") -> ()  [unwired: 1 in, 1 out]
                  }
                  frame #1 {
                    n437 = One Button Dialog(message="Warning2: Projector of disc 6 is off.") -> ()  [unwired: 1 in, 1 out]
                  }
                  frame #2 {
                    n438 = One Button Dialog(message="Warning4: Disc 6 is stop.") -> ()  [unwired: 1 in, 1 out]
                  }
                }
              }
              frame 12 {
                n439 = flat-sequence {
                  frame #0 {
                    n440 = One Button Dialog(message="Warning3: control mode of disc 6 is manual.") -> ()  [unwired: 1 in, 1 out]
                  }
                  frame #1 {
                    n441 = One Button Dialog(message="Warning4: Disc 6 is stop.") -> ()  [unwired: 1 in, 1 out]
                  }
                }
              }
              frame 13 {
                n442 = flat-sequence {
                  frame #0 {
                    n443 = One Button Dialog(message="Warning1: Camera of disc 6 is off.") -> ()  [unwired: 1 in, 1 out]
                  }
                  frame #1 {
                    n444 = One Button Dialog(message="Warning3: control mode of disc 6 is manual.") -> ()  [unwired: 1 in, 1 out]
                  }
                  frame #2 {
                    n445 = One Button Dialog(message="Warning4: Disc 6 is stop.") -> ()  [unwired: 1 in, 1 out]
                  }
                }
              }
              frame 14 {
                n446 = flat-sequence {
                  frame #0 {
                    n447 = One Button Dialog(message="Warning2: Projector of disc 6 is off.") -> ()  [unwired: 1 in, 1 out]
                  }
                  frame #1 {
                    n448 = One Button Dialog(message="Warning3: control mode of disc 6 is manual.") -> ()  [unwired: 1 in, 1 out]
                  }
                  frame #2 {
                    n449 = One Button Dialog(message="Warning4: Disc 6 is stop.") -> ()  [unwired: 1 in, 1 out]
                  }
                }
              }
              frame 15 {
                n450 = flat-sequence {
                  frame #0 {
                    n451 = One Button Dialog(message="Warning1: Camera of disc 6 is off.") -> ()  [unwired: 1 in, 1 out]
                  }
                  frame #1 {
                    n452 = One Button Dialog(message="Warning2: Projector of disc 6 is off.") -> ()  [unwired: 1 in, 1 out]
                  }
                  frame #2 {
                    n453 = One Button Dialog(message="Warning3: control mode of disc 6 is manual.") -> ()  [unwired: 1 in, 1 out]
                  }
                  frame #3 {
                    n454 = One Button Dialog(message="Warning4: Disc 6 is stop.") -> ()  [unwired: 1 in, 1 out]
                  }
                }
              }
            }
          }
        }
      }
      event Timeout {
        w635 = 0 ("index")
        w649 = 100.0 ("y")
        n455 = event-data() -> ()  [unwired: 1 in, 3 out]
        n456 = call "speed average.vi"("initialized array"=w646, "window size"=w645, "array speed in"=w642) -> ("1D array speed"=w644:dbl[], "2D average speed"=w643:dbl[][])  [unwired: 11 in]
        n457 = shared-variable ".\\User Lib.lvlib\\Cancel Login"() -> (w698:bool, error out=w697:errorcluster)  [unwired: 1 in]
        n458 = Get Date/Time In Seconds() -> (seconds since 1Jan1904=w666:timestamp)
        n459 = Format Date/Time String(time format string (%c)="%Y/%m/%d  %H:%M", seconds (now)=w666) -> (date/time string=→"time&date":string)  [unwired: 1 in]
        n460 = Multiply(x=w644, y=0.000116) -> (x*y=w647:dbl[])
        n461 = case shown="True" w698 {
          tunnel: w697 -> [_ w705]
          frame False {
          }
          frame True {
            n462 = property on="Login" class="Bool (strict)"(error in=w705, "Value"=TRUE ("Login")) -> ()  [unwired: 1 in, 2 out]
          }
        }
        n463 = Multiply(x=w647, y=w649) -> (x*y=w650:dbl[])
        n464 = Index Array(array=w640, index #1=0 ("index")) -> (element #1=w689:u8, element #2=w693:u8)  [unwired: 1 in]
        n465 = Round To Nearest(number=w650) -> (nearest integer value=w648:dbl[])
        n466 = Number To Boolean Array(number=w689) -> (Boolean array=w692:bool[])
        n467 = Number To Boolean Array(number=w693) -> (Boolean array=w690:bool[])
        n468 = Divide(x=w648, y=w649) -> (x/y=w638:dbl[])
        n469 = shared-variable ".\\User Lib.lvlib\\Is Dorsa?"() -> (w695:bool)  [unwired: 1 in, 1 out]
        n470 = shared-variable ".\\User Lib.lvlib\\User Flag"() -> (w696:bool)  [unwired: 1 in, 1 out]
        n471 = Index Array(array=w690) -> (element #1=→"DISC 05":bool, element #2=→"AUTO/MAN 05":bool, element #3=→"DISC 06":bool, element #4=→"AUTO/MAN 06":bool)  [unwired: 4 in]
        n472 = Index Array(array=w692, index #1=0 ("index")) -> (element #1=→"DISC 01":bool, element #2=→"AUTO/MAN 01":bool, element #3=→"DISC 02":bool, element #4=→"AUTO/MAN 02":bool, element #5=→"DISC 03":bool, element #6=→"AUTO/MAN 03":bool, element #7=→"DISC 04":bool, element #8=→"AUTO/MAN 04":bool)  [unwired: 7 in]
        n473 = Index Array(array=w638, index=w635) -> (element=w634:dbl)
        n474 = Multiply(x=w634, y=1.03) -> (x*y=w633:dbl)
        n475 = case shown="False" w696 {
          frame False {
            n476 = property on="Setting" class="Bool (strict)"("DisabledEnum"=T18."Disabled and Grayed Out" ("Disabled")) -> ()  [unwired: 2 in, 2 out]
            n477 = property on="Report" class="Bool (strict)"("DisabledEnum"=T18."Disabled and Grayed Out" ("Disabled")) -> ()  [unwired: 2 in, 2 out]
          }
          frame True {
            n478 = property on="Report" class="Bool (strict)"("DisabledEnum"=T18."Enabled" ("Disabled")) -> ()  [unwired: 2 in, 2 out]
            n479 = property on="Setting" class="Bool (strict)"("DisabledEnum"=T18."Enabled" ("Disabled")) -> ()  [unwired: 2 in, 2 out]
          }
        }
        n480 = case shown="False" w695 {
          frame False {
            n481 = property on="Maintenance" class="Bool (strict)"("DisabledEnum"=T18."Disabled and Grayed Out" ("Disabled")) -> ()  [unwired: 2 in, 2 out]
          }
          frame True {
            n482 = property on="Maintenance" class="Bool (strict)"("DisabledEnum"=T18."Enabled" ("Disabled")) -> ()  [unwired: 2 in, 2 out]
          }
        }
        n483 = Replace Array Subset(array=w638, new element=w633, index=w635) -> (w632:dbl[])
        n484 = shared-variable ".\\trends.lvlib\\SpeedArray"(w632) -> ()  [unwired: 1 in, 1 out]
        n485 = Index Array(array=w632, index #1=0 ("index")) -> (element #1=w636:dbl, element #2=w683:dbl, element #3=w682:dbl, element #4=w681:dbl, element #5=w680:dbl, element #6=w669:dbl)  [unwired: 5 in]
        "SPEED 01" <- w636
        "SPEED 02" <- w683
        "SPEED 03" <- w682
        "SPEED 04" <- w681
        "SPEED 05" <- w680
        "SPEED 06" <- w669
        n486 = shared-variable ".\\control setting.lvlib\\SpeedLimit"() -> (w687:dbl[])  [unwired: 1 in, 1 out]
        n487 = Index Array(array=w687, index #1=0 ("index")) -> (element #1=w667:dbl, element #2=w668:dbl)  [unwired: 1 in]
        n488 = Less Or Equal?(x=w636, y=w668) -> (x <= y?=→"speed  min 01":bool)
        n489 = Greater Or Equal?(x=w636, y=w667) -> (x >= y?=→"speed max 01":bool)
        n490 = Less Or Equal?(x=w683, y=w668) -> (x <= y?=→"speed  min 02":bool)
        n491 = Greater Or Equal?(x=w683, y=w667) -> (x >= y?=→"speed max 02":bool)
        n492 = Less Or Equal?(x=w682, y=w668) -> (x <= y?=→"speed  min 03":bool)
        n493 = Greater Or Equal?(x=w682, y=w667) -> (x >= y?=→"speed max 03":bool)
        n494 = Less Or Equal?(x=w681, y=w668) -> (x <= y?=→"speed  min 04":bool)
        n495 = Greater Or Equal?(x=w681, y=w667) -> (x >= y?=→"speed max 04":bool)
        n496 = Less Or Equal?(x=w680, y=w668) -> (x <= y?=→"speed  min 05":bool)
        n497 = Greater Or Equal?(x=w680, y=w667) -> (x >= y?=→"speed max 05":bool)
        n498 = Less Or Equal?(x=w669, y=w668) -> (x <= y?=→"speed  min 06":bool)
        n499 = Greater Or Equal?(x=w669, y=w667) -> (x >= y?=→"speed max 06":bool)
        "error out 14" <- w639
        "error out 12" <- w641
      }
    }
    n500 = Wait (ms)(milliseconds to wait=u32 10) -> ()  [unwired: 1 out]
  }
  n501 = while {
    tunnel: [w708] -> w19
    stop <- w709 stop-if-true
    n502 = Wait (ms)(milliseconds to wait=u32 5) -> ()  [unwired: 1 out]
    n503 = call "Elapsed Time3"() -> ("Elapsed Time (s)"=w711:dbl, "error out"=w708:errorcluster)  [unwired: 12 in, 6 out]
    n504 = Greater Or Equal?(x=w711, y=60.0) -> (x >= y?=w709:bool)
  }
  n505 = call "maintenance.vi"() -> ()  [unwired: 12 in]
  n506 = call "report.vi"() -> ()  [unwired: 12 in]
  n507 = call "DetectedPelletPage.vi"() -> ()  [unwired: 12 in]
  n508 = call "setting.vi"() -> ()  [unwired: 12 in]
  n509 = property on="Login" class="Bool (strict)"("Value"=TRUE ("Login")) -> ()  [unwired: 2 in, 2 out]
  n510 = call "live view D01.vi"() -> ()  [unwired: 16 in]
  n511 = call "live view D02.vi"() -> ()  [unwired: 16 in]
  n512 = call "live view D03.vi"() -> ()  [unwired: 16 in]
  n513 = call "live view D04.vi"() -> ()  [unwired: 16 in]
  n514 = Initialize Array(i8 0 ("element"), 60 ("dimension size")) -> (w76:i8[])
  n515 = call "live view D05.vi"() -> ()  [unwired: 16 in]
  n516 = call <vilib>:"FL Load Fuzzy System.vi"("error in (no error)"=w19, "file path"=path "C:/Users/Dorsa co/Desktop/dsgs pasargad siterun/software/fuzzy pasargad.fs") -> ("error out"=w20:errorcluster, "fuzzy system out"=w53:T21)  [unwired: 8 in]
  n517 = for {
    tunnel: w76 -> [w715] mode=indexing
    tunnel: [w712] -> w52 mode=indexing
    i -> [w714]
    n518 = Increment(x=w714) -> (x+1=w713:i32)
    n519 = Add(x=w715, y=w713) -> (x+y=w712:i32)
  }
  n520 = call "live view D06.vi"() -> ()  [unwired: 16 in]
  n521 = call "TrendsD01.vi"() -> ()  [unwired: 12 in]
  n522 = property on="task out analog" class="DigNum (strict)"() -> ("Value"=w22:i32)  [unwired: 2 in, 2 out]
  n523 = call "TrendsD02.vi"() -> ()  [unwired: 12 in]
  n524 = call "TrendsD03.vi"() -> ()  [unwired: 12 in]
  n525 = property on="task out digital" class="DigNum (strict)"() -> ("Value"=w21:i32)  [unwired: 2 in, 2 out]
  n526 = call "TrendsD04.vi"() -> ()  [unwired: 12 in]
  n527 = call "TrendsD05.vi"() -> ()  [unwired: 12 in]
  n528 = call "TrendsD06.vi"() -> ()  [unwired: 12 in]
  n529 = call <userlib>:"DAQNavi Stop Task.vi"("task in"=w6) -> ()  [unwired: 1 in, 2 out]
  n530 = call "Login.vi"() -> ()  [unwired: 12 in]
  n531 = while {
    tunnel: w53 -> [w747]
    tunnel: w52 -> [w746]
    tunnel: w21 -> [w718]
    tunnel: w20 -> [w719]
    tunnel: w22 -> [w745]
    tunnel: [w718] -> w5
    tunnel: [w717] -> w4
    tunnel: [w716] -> w3
    stop <- FALSE stop-if-true
    # "Control Loop"
    n532 = flat-sequence {
      tunnel: w719 -> [w760]
      tunnel: w747 -> [w759]
      tunnel: w746 -> [w758]
      tunnel: w718 -> [w757]
      tunnel: w745 -> [w751]
      tunnel: [w756] -> w744
      tunnel: [w755] -> w743
      tunnel: [w754] -> w742
      tunnel: [w753] -> w741
      tunnel: [w752] -> w740
      tunnel: [w751] -> w717
      tunnel: w744 -> [w907]
      tunnel: w743 -> [w906]
      tunnel: w742 -> [w905]
      tunnel: w741 -> [w904]
      tunnel: w740 -> [w903]
      tunnel: [w900] -> w739
      tunnel: [w899] -> w738
      tunnel: [w898] -> w737
      tunnel: [w897] -> w736
      tunnel: [w896] -> w735
      tunnel: w739 -> [w1056]
      tunnel: w738 -> [w1055]
      tunnel: w737 -> [w1054]
      tunnel: w736 -> [w1053]
      tunnel: w735 -> [w1052]
      tunnel: [w1049] -> w734
      tunnel: [w1048] -> w733
      tunnel: [w1047] -> w732
      tunnel: [w1046] -> w731
      tunnel: [w1045] -> w730
      tunnel: w734 -> [w1205]
      tunnel: w733 -> [w1204]
      tunnel: w732 -> [w1203]
      tunnel: w731 -> [w1202]
      tunnel: w730 -> [w1201]
      tunnel: [w1198] -> w729
      tunnel: [w1197] -> w728
      tunnel: [w1196] -> w727
      tunnel: [w1195] -> w726
      tunnel: [w1194] -> w725
      tunnel: w729 -> [w1354]
      tunnel: w728 -> [w1353]
      tunnel: w727 -> [w1352]
      tunnel: w726 -> [w1351]
      tunnel: w725 -> [w1350]
      tunnel: [w1346] -> w724
      tunnel: [w1345] -> w723
      tunnel: [w1344] -> w722
      tunnel: [w1343] -> w721
      tunnel: [w1342] -> w720
      tunnel: w724 -> [w1499]
      tunnel: w723 -> [w1498]
      tunnel: w722 -> [w1497]
      tunnel: w721 -> [w1496]
      tunnel: w720 -> [w1495]
      tunnel: [w1491] -> w716
      frame #0 {
        n533 = property on="AUTO/MAN 01" class="Bool (strict)"() -> ("Value"=w750:bool)  [unwired: 2 in, 2 out]
        n534 = property on="DISC 01" class="Bool (strict)"() -> ("Value"=w762:bool)  [unwired: 2 in, 2 out]
        n535 = And(x=w750, y=w762) -> (x .and. y?=w761:bool)
        n536 = case shown="True" w761 {
          tunnel: w759 -> [w764 w800]
          tunnel: w760 -> [w767 w799]
          tunnel: w758 -> [w763 w791]
          tunnel: w757 -> [w765 w787]
          tunnel: w751 -> [w766 w785]
          tunnel: [w767 w783] -> w753
          tunnel: [w766 w781] -> w756
          tunnel: [w765 w779] -> w755
          tunnel: [w764 w777] -> w754
          tunnel: [w763 w775] -> w752
          frame False {
          }
          frame True {
            n537 = flat-sequence {
              tunnel: w800 -> [w815]
              tunnel: w799 -> [w816]
              tunnel: w791 -> [w817]
              tunnel: [w817] -> w798
              tunnel: [w816] -> w797
              tunnel: [w815] -> w796
              tunnel: [w804] -> w790
              tunnel: [w803] -> w788
              tunnel: w787 -> [w803]
              tunnel: [w802] -> w786
              tunnel: w785 -> [w802]
              tunnel: [w826] -> w795
              tunnel: [w820] -> w794
              tunnel: [w832] -> w793
              tunnel: [w819] -> w792
              tunnel: w798 -> [w819]
              tunnel: w797 -> [w834]
              tunnel: w796 -> [w820]
              tunnel: w790 -> [w823]
              tunnel: [w821] -> w789
              tunnel: w788 -> [w821]
              tunnel: w786 -> [w822]
              tunnel: [w822] -> w784
              tunnel: [w822] -> w782
              tunnel: [w821] -> w780
              tunnel: [w820] -> w778
              tunnel: [w819] -> w776
              tunnel: [w818] -> w774
              tunnel: w795 -> [w851]
              tunnel: w794 -> [w849]
              tunnel: w793 -> [w850]
              tunnel: w792 -> [w848]
              tunnel: w789 -> [w847]
              tunnel: w784 -> [w846]
              tunnel: w782 -> [w844]
              tunnel: w780 -> [w843]
              tunnel: w778 -> [w842]
              tunnel: w776 -> [w841]
              tunnel: w774 -> [w840]
              tunnel: [w845] -> w773
              tunnel: [w844] -> w772
              tunnel: [w843] -> w771
              tunnel: [w842] -> w770
              tunnel: [w841] -> w769
              tunnel: [w839] -> w768
              tunnel: [w890] -> w775
              tunnel: [w891] -> w777
              tunnel: [w892] -> w779
              tunnel: [w893] -> w781
              tunnel: [w894] -> w783
              tunnel: w773 -> [w894]
              tunnel: w772 -> [w893]
              tunnel: w771 -> [w892]
              tunnel: w770 -> [w891]
              tunnel: w769 -> [w890]
              tunnel: w768 -> [w889]
              frame #0 {
                n538 = shared-variable ".\\control setting.lvlib\\SetPoints"() -> (w810:dbl[])  [unwired: 1 in, 1 out]
                n539 = property on="2D array out" class="Arr (strict)"() -> ("Value"=w814:dbl[][])  [unwired: 2 in, 2 out]
                n540 = shared-variable ".\\control setting.lvlib\\ErrorThr"() -> (w801:dbl)  [unwired: 1 in, 1 out]
                n541 = property on="speed max 01" class="Bool (strict)"() -> ("Value"=w806:bool)  [unwired: 2 in, 2 out]
                n542 = property on="no change D01" class="Bool (strict)"() -> ("Value"=w805:bool)  [unwired: 2 in, 2 out]
                n543 = property on="speed  min 01" class="Bool (strict)"() -> ("Value"=w807:bool)  [unwired: 2 in, 2 out]
                n544 = Index Array(array=w814, index (row)=0, index (col)=0 ("disabled index (col)")) -> (element=w809:dbl)
                n545 = Index Array(array=w810, index=0) -> (element=w808:dbl)
                n546 = call "sudden change.vi"("error in"=w809, "set point"=w808, "speed min"=w807, "speed max"=w806, "no change"=w805, "sudden threshould"=w801) -> ("sudden change"=w804:bool)  [unwired: 13 in]
                "sudden change D01" <- w804
              }
              frame #1 {
                # "D26 Tick count to reach the pulse time (defult : 5min)"
                n547 = Boolean To (0,1)(Boolean=w823) -> (0, 1=w827:i16)
                n548 = shared-variable ".\\control setting.lvlib\\PlsePeriod"() -> (w830:i16)  [unwired: 1 in, 1 out]
                n549 = Build Array(w827) -> (w828:i16[])
                n550 = call-poly <vilib>:"Basic Level Trigger Detection.vi"("signal in"=w828, "level"=0.5) -> ("trigger detected?"=w824:bool)  [unwired: 11 in, 2 out]
                n551 = call "Elapsed Time"("Time Target (s)"=w830, "Reset"=w824, "error in (no error)"=w834) -> ("Elapsed Time (s)"=w825:dbl, "error out"=w833:errorcluster)  [unwired: 9 in, 6 out]
                n552 = In Range and Coerce(upper limit=10.0, x=w825, lower limit=0.1) -> (In Range?=w818:bool)  [unwired: 1 out]
                n553 = Boolean To (0,1)(Boolean=w818) -> (0, 1=w831:i16)
                n554 = Build Array(w831) -> (w838:i16[])
                n555 = call-poly <vilib>:"Basic Level Trigger Detection.vi"("signal in"=w838, "level"=0.5, "error in (no error)"=w833) -> ("trigger detected?"=w826:bool, "error out"=w832:errorcluster)  [unwired: 10 in, 1 out]
              }
              frame #2 {
                n556 = case shown="True" w851 {
                  tunnel: w849 -> [_ w881]
                  tunnel: w850 -> [w853 w887]
                  tunnel: [w853 w865] -> w845
                  tunnel: w848 -> [_ w864]
                  tunnel: w847 -> [_ w876]
                  tunnel: w846 -> [_ w867]
                  tunnel: w840 -> [w852 w854]
                  tunnel: [w852 w854] -> w839
                  frame False {
                  }
                  frame True {
                    n557 = property on="2D array out" class="Arr (strict)"(error in=w887) -> (error out=w877:errorcluster, "Value"=w883:dbl[][])  [unwired: 1 in, 1 out]
                    n558 = shared-variable ".\\control setting.lvlib\\SetPoints"() -> (w885:dbl[])  [unwired: 1 in, 1 out]
                    n559 = Index Array(array=w885, index=0) -> (element=w879:dbl)
                    n560 = Index Array(array=w883, index (row)=0 ("disabled index (row)"), index (col)=0 ("disabled index (col)")) -> (element=w880:dbl)
                    n561 = Index Array(array=w883, index (col)=0 ("disabled index (col)")) -> (element=w878:dbl[])  [unwired: 1 in]
                    n562 = shared-variable ".\\control setting.lvlib\\SpeedLimit"() -> (w872:dbl[])  [unwired: 1 in, 1 out]
                    n563 = call "fuzzy rules.vi"("error"=w880, "set point"=w879, "error array"=w878, "X"=w864, "error in (no error)"=w877, "fuzzy system in"=w881) -> ("last error"=w859:dbl, "slope"=w856:dbl, "output value"=w857:dbl, "error out"=w866:errorcluster)  [unwired: 9 in, 1 out]
                    n564 = property on="SPEED 01" class="DigNum (strict)"() -> ("Value"=w858:dbl)  [unwired: 2 in, 2 out]
                    n565 = Index Array(array=w872, index #1=0 ("index")) -> (element #1=w870:dbl, element #2=w869:dbl)  [unwired: 1 in]
                    n566 = Build Array(1) -> (w874:i32[])
                    n567 = property on="sudden change D01" class="Bool (strict)"() -> ("Value"=w860:bool)  [unwired: 2 in, 2 out]
                    n568 = call "speed to disc.vi"("task in digital"=w876, "data"=w874, "speed change"=w857, "change limit"=0.025, "speed max limit"=w870, "speed min limit"=w869, "speed in"=w858, "wait time"=u32 1000, "task inAnalog"=w867, "error in (no error)"=w866) -> ("inc"=w862:bool, "dec"=w863:bool, "no change"=w861:bool, "error out"=w865:errorcluster)  [unwired: 13 in, 1 out]
                    "no change D01" <- w861
                    "increase D01" <- w862
                    "decrease D01" <- w863
                    n569 = Bundle("dec"=w863, "inc"=w862, "no change"=w861, "Value"=w860, "last error"=w859, "Value"=w858, "output value"=w857, "slope"=w856) -> (w855:T33)  [unwired: 1 in]
                    n570 = shared-variable ".\\control setting.lvlib\\ControlInfoD01"(w855) -> ()  [unwired: 1 in, 1 out]
                  }
                }
              }
              frame #3 {
                n571 = shared-variable ".\\D01.lvlib\\change D01"(w889) -> ()  [unwired: 1 in, 1 out]
              }
            }
          }
        }
      }
      frame #1 {
        n572 = property on="DISC 02" class="Bool (strict)"() -> ("Value"=w902:bool)  [unwired: 2 in, 2 out]
        n573 = property on="AUTO/MAN 02" class="Bool (strict)"() -> ("Value"=w895:bool)  [unwired: 2 in, 2 out]
        n574 = And(x=w895, y=w902) -> (x .and. y?=w901:bool)
        n575 = case shown="True" w901 {
          tunnel: w905 -> [w909 w947]
          tunnel: w904 -> [w912 w946]
          tunnel: w903 -> [w908 w938]
          tunnel: w906 -> [w910 w934]
          tunnel: w907 -> [w911 w932]
          tunnel: [w912 w930] -> w897
          tunnel: [w911 w928] -> w900
          tunnel: [w910 w926] -> w899
          tunnel: [w909 w924] -> w898
          tunnel: [w908 w922] -> w896
          frame False {
          }
          frame True {
            n576 = flat-sequence {
              tunnel: w947 -> [w962]
              tunnel: w946 -> [w963]
              tunnel: w938 -> [w964]
              tunnel: [w964] -> w945
              tunnel: [w963] -> w944
              tunnel: [w962] -> w943
              tunnel: [w948] -> w937
              tunnel: [w952] -> w935
              tunnel: w934 -> [w952]
              tunnel: [w951] -> w933
              tunnel: w932 -> [w951]
              tunnel: [w948] -> w920
              tunnel: [w974] -> w942
              tunnel: [w968] -> w941
              tunnel: [w980] -> w940
              tunnel: [w967] -> w939
              tunnel: w945 -> [w967]
              tunnel: w944 -> [w982]
              tunnel: w943 -> [w968]
              tunnel: w937 -> [w971]
              tunnel: [w969] -> w936
              tunnel: w935 -> [w969]
              tunnel: w933 -> [w970]
              tunnel: [w970] -> w931
              tunnel: [w970] -> w929
              tunnel: [w969] -> w927
              tunnel: [w968] -> w925
              tunnel: [w967] -> w923
              tunnel: [w966] -> w921
              tunnel: w920 -> [w966]
              tunnel: [w965] -> w919
              tunnel: w942 -> [w1000]
              tunnel: w941 -> [w998]
              tunnel: w940 -> [w999]
              tunnel: w939 -> [w997]
              tunnel: w936 -> [w996]
              tunnel: w931 -> [w995]
              tunnel: w929 -> [w993]
              tunnel: w927 -> [w992]
              tunnel: w925 -> [w991]
              tunnel: w923 -> [w990]
              tunnel: w921 -> [w989]
              tunnel: w919 -> [w988]
              tunnel: [w994] -> w918
              tunnel: [w993] -> w917
              tunnel: [w992] -> w916
              tunnel: [w991] -> w915
              tunnel: [w990] -> w914
              tunnel: [w987] -> w913
              tunnel: [w1039] -> w922
              tunnel: [w1040] -> w924
              tunnel: [w1041] -> w926
              tunnel: [w1042] -> w928
              tunnel: [w1043] -> w930
              tunnel: w918 -> [w1043]
              tunnel: w917 -> [w1042]
              tunnel: w916 -> [w1041]
              tunnel: w915 -> [w1040]
              tunnel: w914 -> [w1039]
              tunnel: w913 -> [w1038]
              frame #0 {
                n577 = shared-variable ".\\control setting.lvlib\\SetPoints"() -> (w957:dbl[])  [unwired: 1 in, 1 out]
                n578 = property on="2D array out" class="Arr (strict)"() -> ("Value"=w961:dbl[][])  [unwired: 2 in, 2 out]
                n579 = shared-variable ".\\control setting.lvlib\\ErrorThr"() -> (w949:dbl)  [unwired: 1 in, 1 out]
                n580 = property on="speed max 02" class="Bool (strict)"() -> ("Value"=w953:bool)  [unwired: 2 in, 2 out]
                n581 = property on="speed  min 02" class="Bool (strict)"() -> ("Value"=w954:bool)  [unwired: 2 in, 2 out]
                n582 = property on="no change D02" class="Bool (strict)"() -> ("Value"=w950:bool)  [unwired: 2 in, 2 out]
                n583 = Index Array(array=w961, index (row)=0, index (col)=1 ("disabled index (col)")) -> (element=w956:dbl)
                n584 = Index Array(array=w957, index=1) -> (element=w955:dbl)
                n585 = call "sudden change.vi"("error in"=w956, "set point"=w955, "speed min"=w954, "speed max"=w953, "no change"=w950, "sudden threshould"=w949) -> ("sudden change"=w948:bool)  [unwired: 13 in]
                "sudden change D02" <- w948
              }
              frame #1 {
                # "D26 Tick count to reach the pulse time (defult : 5min)"
                n586 = Boolean To (0,1)(Boolean=w971) -> (0, 1=w975:i16)
                n587 = shared-variable ".\\control setting.lvlib\\PlsePeriod"() -> (w978:i16)  [unwired: 1 in, 1 out]
                n588 = Build Array(w975) -> (w976:i16[])
                n589 = call-poly <vilib>:"Basic Level Trigger Detection.vi"("signal in"=w976, "level"=0.5) -> ("trigger detected?"=w972:bool)  [unwired: 11 in, 2 out]
                n590 = call "Elapsed Time2"("Time Target (s)"=w978, "Reset"=w972, "error in (no error)"=w982) -> ("Elapsed Time (s)"=w973:dbl, "error out"=w981:errorcluster)  [unwired: 9 in, 6 out]
                n591 = In Range and Coerce(upper limit=10.0, x=w973, lower limit=0.1) -> (In Range?=w965:bool)  [unwired: 1 out]
                n592 = Boolean To (0,1)(Boolean=w965) -> (0, 1=w979:i16)
                n593 = Build Array(w979) -> (w986:i16[])
                n594 = call-poly <vilib>:"Basic Level Trigger Detection.vi"("signal in"=w986, "level"=0.5, "error in (no error)"=w981) -> ("trigger detected?"=w974:bool, "error out"=w980:errorcluster)  [unwired: 10 in, 1 out]
              }
              frame #2 {
                n595 = case shown="True" w1000 {
                  tunnel: w998 -> [_ w1030]
                  tunnel: w999 -> [w1002 w1036]
                  tunnel: [w1002 w1015] -> w994
                  tunnel: w997 -> [_ w1014]
                  tunnel: w996 -> [_ w1025]
                  tunnel: w995 -> [_ w1016]
                  tunnel: w989 -> [_ w1010]
                  tunnel: w988 -> [w1001 w1003]
                  tunnel: [w1001 w1003] -> w987
                  frame False {
                  }
                  frame True {
                    n596 = property on="2D array out" class="Arr (strict)"(error in=w1036) -> (error out=w1026:errorcluster, "Value"=w1032:dbl[][])  [unwired: 1 in, 1 out]
                    n597 = shared-variable ".\\control setting.lvlib\\SetPoints"() -> (w1034:dbl[])  [unwired: 1 in, 1 out]
                    n598 = Index Array(array=w1034, index=1) -> (element=w1028:dbl)
                    n599 = Index Array(array=w1032, index (row)=0 ("disabled index (row)"), index (col)=1 ("disabled index (col)")) -> (element=w1029:dbl)
                    n600 = Index Array(array=w1032, index (col)=1 ("disabled index (col)")) -> (element=w1027:dbl[])  [unwired: 1 in]
                    n601 = shared-variable ".\\control setting.lvlib\\SpeedLimit"() -> (w1021:dbl[])  [unwired: 1 in, 1 out]
                    n602 = call "fuzzy rules.vi"("error"=w1029, "set point"=w1028, "error array"=w1027, "X"=w1014, "error in (no error)"=w1026, "fuzzy system in"=w1030) -> ("last error"=w1009:dbl, "slope"=w1006:dbl, "output value"=w1007:dbl, "error out"=w1013:errorcluster)  [unwired: 9 in, 1 out]
                    "last error 02" <- w1009
                    "slope D02" <- w1006
                    n603 = property on="SPEED 02" class="DigNum (strict)"() -> ("Value"=w1008:dbl)  [unwired: 2 in, 2 out]
                    n604 = Index Array(array=w1021, index #1=0 ("index")) -> (element #1=w1019:dbl, element #2=w1018:dbl)  [unwired: 1 in]
                    n605 = Build Array(2) -> (w1023:i32[])
                    n606 = call "speed to disc.vi"("task in digital"=w1025, "data"=w1023, "speed change"=w1007, "change limit"=0.025, "speed max limit"=w1019, "speed min limit"=w1018, "speed in"=w1008, "wait time"=u32 1000, "task inAnalog"=w1016, "error in (no error)"=w1013) -> ("inc"=w1004:bool, "dec"=w1012:bool, "no change"=w1011:bool, "error out"=w1015:errorcluster)  [unwired: 13 in, 1 out]
                    "increase D02" <- w1004
                    "decrease D02" <- w1012
                    "no change D02" <- w1011
                    n607 = Bundle("dec"=w1012, "inc"=w1004, "no change"=w1011, "sudden change"=w1010, "last error"=w1009, "Value"=w1008, "output value"=w1007, "slope"=w1006) -> (w1005:T34)  [unwired: 1 in]
                    n608 = shared-variable ".\\control setting.lvlib\\ControlInfoD02"(w1005) -> ()  [unwired: 1 in, 1 out]
                  }
                }
              }
              frame #3 {
                n609 = shared-variable ".\\D02.lvlib\\change D02"(w1038) -> ()  [unwired: 1 in, 1 out]
              }
            }
          }
        }
      }
      frame #2 {
        n610 = property on="AUTO/MAN 03" class="Bool (strict)"() -> ("Value"=w1044:bool)  [unwired: 2 in, 2 out]
        n611 = property on="DISC 03" class="Bool (strict)"() -> ("Value"=w1051:bool)  [unwired: 2 in, 2 out]
        n612 = And(x=w1044, y=w1051) -> (x .and. y?=w1050:bool)
        n613 = case shown="True" w1050 {
          tunnel: w1054 -> [w1058 w1096]
          tunnel: w1053 -> [w1061 w1095]
          tunnel: w1052 -> [w1057 w1087]
          tunnel: w1055 -> [w1059 w1083]
          tunnel: w1056 -> [w1060 w1081]
          tunnel: [w1061 w1079] -> w1046
          tunnel: [w1060 w1077] -> w1049
          tunnel: [w1059 w1075] -> w1048
          tunnel: [w1058 w1073] -> w1047
          tunnel: [w1057 w1071] -> w1045
          frame False {
          }
          frame True {
            n614 = flat-sequence {
              tunnel: w1096 -> [w1111]
              tunnel: w1095 -> [w1112]
              tunnel: w1087 -> [w1113]
              tunnel: [w1113] -> w1094
              tunnel: [w1112] -> w1093
              tunnel: [w1111] -> w1092
              tunnel: [w1097] -> w1086
              tunnel: [w1101] -> w1084
              tunnel: w1083 -> [w1101]
              tunnel: [w1100] -> w1082
              tunnel: w1081 -> [w1100]
              tunnel: [w1097] -> w1069
              tunnel: [w1123] -> w1091
              tunnel: [w1117] -> w1090
              tunnel: [w1129] -> w1089
              tunnel: [w1116] -> w1088
              tunnel: w1094 -> [w1116]
              tunnel: w1093 -> [w1131]
              tunnel: w1092 -> [w1117]
              tunnel: w1086 -> [w1120]
              tunnel: [w1118] -> w1085
              tunnel: w1084 -> [w1118]
              tunnel: w1082 -> [w1119]
              tunnel: [w1119] -> w1080
              tunnel: [w1119] -> w1078
              tunnel: [w1118] -> w1076
              tunnel: [w1117] -> w1074
              tunnel: [w1116] -> w1072
              tunnel: [w1115] -> w1070
              tunnel: w1069 -> [w1115]
              tunnel: [w1114] -> w1068
              tunnel: w1091 -> [w1149]
              tunnel: w1090 -> [w1147]
              tunnel: w1089 -> [w1148]
              tunnel: w1088 -> [w1146]
              tunnel: w1085 -> [w1145]
              tunnel: w1080 -> [w1144]
              tunnel: w1078 -> [w1142]
              tunnel: w1076 -> [w1141]
              tunnel: w1074 -> [w1140]
              tunnel: w1072 -> [w1139]
              tunnel: w1070 -> [w1138]
              tunnel: w1068 -> [w1137]
              tunnel: [w1143] -> w1067
              tunnel: [w1142] -> w1066
              tunnel: [w1141] -> w1065
              tunnel: [w1140] -> w1064
              tunnel: [w1139] -> w1063
              tunnel: [w1136] -> w1062
              tunnel: [w1188] -> w1071
              tunnel: [w1189] -> w1073
              tunnel: [w1190] -> w1075
              tunnel: [w1191] -> w1077
              tunnel: [w1192] -> w1079
              tunnel: w1067 -> [w1192]
              tunnel: w1066 -> [w1191]
              tunnel: w1065 -> [w1190]
              tunnel: w1064 -> [w1189]
              tunnel: w1063 -> [w1188]
              tunnel: w1062 -> [w1187]
              frame #0 {
                n615 = shared-variable ".\\control setting.lvlib\\SetPoints"() -> (w1106:dbl[])  [unwired: 1 in, 1 out]
                n616 = property on="2D array out" class="Arr (strict)"() -> ("Value"=w1110:dbl[][])  [unwired: 2 in, 2 out]
                n617 = property on="speed max 03" class="Bool (strict)"() -> ("Value"=w1102:bool)  [unwired: 2 in, 2 out]
                n618 = shared-variable ".\\control setting.lvlib\\ErrorThr"() -> (w1098:dbl)  [unwired: 1 in, 1 out]
                n619 = property on="speed  min 03" class="Bool (strict)"() -> ("Value"=w1103:bool)  [unwired: 2 in, 2 out]
                n620 = property on="no change D03" class="Bool (strict)"() -> ("Value"=w1099:bool)  [unwired: 2 in, 2 out]
                n621 = Index Array(array=w1110, index (row)=0, index (col)=2 ("disabled index (col)")) -> (element=w1105:dbl)
                n622 = Index Array(array=w1106, index=2) -> (element=w1104:dbl)
                n623 = call "sudden change.vi"("error in"=w1105, "set point"=w1104, "speed min"=w1103, "speed max"=w1102, "no change"=w1099, "sudden threshould"=w1098) -> ("sudden change"=w1097:bool)  [unwired: 13 in]
                "sudden change D03" <- w1097
              }
              frame #1 {
                # "D26 Tick count to reach the pulse time (defult : 5min)"
                n624 = Boolean To (0,1)(Boolean=w1120) -> (0, 1=w1124:i16)
                n625 = shared-variable ".\\control setting.lvlib\\PlsePeriod"() -> (w1127:i16)  [unwired: 1 in, 1 out]
                n626 = Build Array(w1124) -> (w1125:i16[])
                n627 = call-poly <vilib>:"Basic Level Trigger Detection.vi"("signal in"=w1125, "level"=0.5) -> ("trigger detected?"=w1121:bool)  [unwired: 11 in, 2 out]
                n628 = call "Elapsed Time11"("Time Target (s)"=w1127, "Reset"=w1121, "error in (no error)"=w1131) -> ("Elapsed Time (s)"=w1122:dbl, "error out"=w1130:errorcluster)  [unwired: 9 in, 6 out]
                n629 = In Range and Coerce(upper limit=10.0, x=w1122, lower limit=0.1) -> (In Range?=w1114:bool)  [unwired: 1 out]
                n630 = Boolean To (0,1)(Boolean=w1114) -> (0, 1=w1128:i16)
                n631 = Build Array(w1128) -> (w1135:i16[])
                n632 = call-poly <vilib>:"Basic Level Trigger Detection.vi"("signal in"=w1135, "level"=0.5, "error in (no error)"=w1130) -> ("trigger detected?"=w1123:bool, "error out"=w1129:errorcluster)  [unwired: 10 in, 1 out]
              }
              frame #2 {
                n633 = case shown="True" w1149 {
                  tunnel: w1147 -> [_ w1179]
                  tunnel: w1148 -> [w1151 w1185]
                  tunnel: [w1151 w1162] -> w1143
                  tunnel: w1146 -> [_ w1163]
                  tunnel: w1145 -> [_ w1174]
                  tunnel: w1144 -> [_ w1165]
                  tunnel: w1138 -> [_ w1158]
                  tunnel: w1137 -> [w1150 w1152]
                  tunnel: [w1150 w1152] -> w1136
                  frame False {
                  }
                  frame True {
                    n634 = property on="2D array out" class="Arr (strict)"(error in=w1185) -> (error out=w1175:errorcluster, "Value"=w1181:dbl[][])  [unwired: 1 in, 1 out]
                    n635 = shared-variable ".\\control setting.lvlib\\SetPoints"() -> (w1183:dbl[])  [unwired: 1 in, 1 out]
                    n636 = Index Array(array=w1183, index=2) -> (element=w1177:dbl)
                    n637 = Index Array(array=w1181, index (row)=0 ("disabled index (row)"), index (col)=2 ("disabled index (col)")) -> (element=w1178:dbl)
                    n638 = Index Array(array=w1181, index (col)=2 ("disabled index (col)")) -> (element=w1176:dbl[])  [unwired: 1 in]
                    n639 = shared-variable ".\\control setting.lvlib\\SpeedLimit"() -> (w1170:dbl[])  [unwired: 1 in, 1 out]
                    n640 = call "fuzzy rules.vi"("error"=w1178, "set point"=w1177, "error array"=w1176, "X"=w1163, "error in (no error)"=w1175, "fuzzy system in"=w1179) -> ("last error"=w1157:dbl, "slope"=w1154:dbl, "output value"=w1155:dbl, "error out"=w1164:errorcluster)  [unwired: 9 in, 1 out]
                    "last error 03" <- w1157
                    "slope D03" <- w1154
                    n641 = property on="SPEED 03" class="DigNum (strict)"() -> ("Value"=w1156:dbl)  [unwired: 2 in, 2 out]
                    n642 = Index Array(array=w1170, index #1=0 ("index")) -> (element #1=w1168:dbl, element #2=w1167:dbl)  [unwired: 1 in]
                    n643 = Build Array(3) -> (w1172:i32[])
                    n644 = call "speed to disc.vi"("task in digital"=w1174, "data"=w1172, "speed change"=w1155, "change limit"=0.025, "speed max limit"=w1168, "speed min limit"=w1167, "speed in"=w1156, "wait time"=u32 1000, "task inAnalog"=w1165, "error in (no error)"=w1164) -> ("inc"=w1160:bool, "dec"=w1161:bool, "no change"=w1159:bool, "error out"=w1162:errorcluster)  [unwired: 13 in, 1 out]
                    "increase D03" <- w1160
                    "decrease D03" <- w1161
                    "no change D03" <- w1159
                    n645 = Bundle("dec"=w1161, "inc"=w1160, "no change"=w1159, "sudden change"=w1158, "last error"=w1157, "Value"=w1156, "output value"=w1155, "slope"=w1154) -> (w1153:T34)  [unwired: 1 in]
                    n646 = shared-variable ".\\control setting.lvlib\\ControlInfoD03"(w1153) -> ()  [unwired: 1 in, 1 out]
                  }
                }
              }
              frame #3 {
                n647 = shared-variable ".\\D03.lvlib\\change D03"(w1187) -> ()  [unwired: 1 in, 1 out]
              }
            }
          }
        }
      }
      frame #3 {
        n648 = property on="AUTO/MAN 04" class="Bool (strict)"() -> ("Value"=w1193:bool)  [unwired: 2 in, 2 out]
        n649 = property on="DISC 04" class="Bool (strict)"() -> ("Value"=w1200:bool)  [unwired: 2 in, 2 out]
        n650 = And(x=w1193, y=w1200) -> (x .and. y?=w1199:bool)
        n651 = case shown="True" w1199 {
          tunnel: w1203 -> [w1207 w1245]
          tunnel: w1202 -> [w1210 w1244]
          tunnel: w1201 -> [w1206 w1236]
          tunnel: w1204 -> [w1208 w1232]
          tunnel: w1205 -> [w1209 w1230]
          tunnel: [w1210 w1228] -> w1195
          tunnel: [w1209 w1226] -> w1198
          tunnel: [w1208 w1224] -> w1197
          tunnel: [w1207 w1222] -> w1196
          tunnel: [w1206 w1220] -> w1194
          frame False {
          }
          frame True {
            n652 = flat-sequence {
              tunnel: w1245 -> [w1260]
              tunnel: w1244 -> [w1261]
              tunnel: w1236 -> [w1262]
              tunnel: [w1262] -> w1243
              tunnel: [w1261] -> w1242
              tunnel: [w1260] -> w1241
              tunnel: [w1246] -> w1235
              tunnel: [w1250] -> w1233
              tunnel: w1232 -> [w1250]
              tunnel: [w1249] -> w1231
              tunnel: w1230 -> [w1249]
              tunnel: [w1246] -> w1218
              tunnel: [w1272] -> w1240
              tunnel: [w1266] -> w1239
              tunnel: [w1278] -> w1238
              tunnel: [w1265] -> w1237
              tunnel: w1243 -> [w1265]
              tunnel: w1242 -> [w1280]
              tunnel: w1241 -> [w1266]
              tunnel: w1235 -> [w1269]
              tunnel: [w1267] -> w1234
              tunnel: w1233 -> [w1267]
              tunnel: w1231 -> [w1268]
              tunnel: [w1268] -> w1229
              tunnel: [w1268] -> w1227
              tunnel: [w1267] -> w1225
              tunnel: [w1266] -> w1223
              tunnel: [w1265] -> w1221
              tunnel: [w1264] -> w1219
              tunnel: w1218 -> [w1264]
              tunnel: [w1263] -> w1217
              tunnel: w1240 -> [w1298]
              tunnel: w1239 -> [w1296]
              tunnel: w1238 -> [w1297]
              tunnel: w1237 -> [w1295]
              tunnel: w1234 -> [w1294]
              tunnel: w1229 -> [w1293]
              tunnel: w1227 -> [w1291]
              tunnel: w1225 -> [w1290]
              tunnel: w1223 -> [w1289]
              tunnel: w1221 -> [w1288]
              tunnel: w1219 -> [w1287]
              tunnel: w1217 -> [w1286]
              tunnel: [w1292] -> w1216
              tunnel: [w1291] -> w1215
              tunnel: [w1290] -> w1214
              tunnel: [w1289] -> w1213
              tunnel: [w1288] -> w1212
              tunnel: [w1285] -> w1211
              tunnel: [w1337] -> w1220
              tunnel: [w1338] -> w1222
              tunnel: [w1339] -> w1224
              tunnel: [w1340] -> w1226
              tunnel: [w1341] -> w1228
              tunnel: w1216 -> [w1341]
              tunnel: w1215 -> [w1340]
              tunnel: w1214 -> [w1339]
              tunnel: w1213 -> [w1338]
              tunnel: w1212 -> [w1337]
              tunnel: w1211 -> [w1336]
              frame #0 {
                n653 = shared-variable ".\\control setting.lvlib\\SetPoints"() -> (w1255:dbl[])  [unwired: 1 in, 1 out]
                n654 = property on="2D array out" class="Arr (strict)"() -> ("Value"=w1259:dbl[][])  [unwired: 2 in, 2 out]
                n655 = shared-variable ".\\control setting.lvlib\\ErrorThr"() -> (w1247:dbl)  [unwired: 1 in, 1 out]
                n656 = property on="speed max 04" class="Bool (strict)"() -> ("Value"=w1251:bool)  [unwired: 2 in, 2 out]
                n657 = property on="speed  min 04" class="Bool (strict)"() -> ("Value"=w1252:bool)  [unwired: 2 in, 2 out]
                n658 = property on="no change D04" class="Bool (strict)"() -> ("Value"=w1248:bool)  [unwired: 2 in, 2 out]
                n659 = Index Array(array=w1259, index (row)=0, index (col)=3 ("disabled index (col)")) -> (element=w1254:dbl)
                n660 = Index Array(array=w1255, index=3) -> (element=w1253:dbl)
                n661 = call "sudden change.vi"("error in"=w1254, "set point"=w1253, "speed min"=w1252, "speed max"=w1251, "no change"=w1248, "sudden threshould"=w1247) -> ("sudden change"=w1246:bool)  [unwired: 13 in]
                "sudden change D04" <- w1246
              }
              frame #1 {
                # "D26 Tick count to reach the pulse time (defult : 5min)"
                n662 = Boolean To (0,1)(Boolean=w1269) -> (0, 1=w1273:i16)
                n663 = shared-variable ".\\control setting.lvlib\\PlsePeriod"() -> (w1276:i16)  [unwired: 1 in, 1 out]
                n664 = Build Array(w1273) -> (w1274:i16[])
                n665 = call-poly <vilib>:"Basic Level Trigger Detection.vi"("signal in"=w1274, "level"=0.5) -> ("trigger detected?"=w1270:bool)  [unwired: 11 in, 2 out]
                n666 = call "Elapsed Time12"("Time Target (s)"=w1276, "Reset"=w1270, "error in (no error)"=w1280) -> ("Elapsed Time (s)"=w1271:dbl, "error out"=w1279:errorcluster)  [unwired: 9 in, 6 out]
                n667 = In Range and Coerce(upper limit=10.0, x=w1271, lower limit=0.1) -> (In Range?=w1263:bool)  [unwired: 1 out]
                n668 = Boolean To (0,1)(Boolean=w1263) -> (0, 1=w1277:i16)
                n669 = Build Array(w1277) -> (w1284:i16[])
                n670 = call-poly <vilib>:"Basic Level Trigger Detection.vi"("signal in"=w1284, "level"=0.5, "error in (no error)"=w1279) -> ("trigger detected?"=w1272:bool, "error out"=w1278:errorcluster)  [unwired: 10 in, 1 out]
              }
              frame #2 {
                n671 = case shown="True" w1298 {
                  tunnel: w1296 -> [_ w1328]
                  tunnel: w1297 -> [w1300 w1334]
                  tunnel: [w1300 w1312] -> w1292
                  tunnel: w1295 -> [_ w1311]
                  tunnel: w1294 -> [_ w1323]
                  tunnel: w1293 -> [_ w1314]
                  tunnel: w1287 -> [_ w1307]
                  tunnel: w1286 -> [w1299 w1301]
                  tunnel: [w1299 w1301] -> w1285
                  frame False {
                  }
                  frame True {
                    n672 = property on="2D array out" class="Arr (strict)"(error in=w1334) -> (error out=w1324:errorcluster, "Value"=w1330:dbl[][])  [unwired: 1 in, 1 out]
                    n673 = shared-variable ".\\control setting.lvlib\\SetPoints"() -> (w1332:dbl[])  [unwired: 1 in, 1 out]
                    n674 = Index Array(array=w1332, index=3) -> (element=w1326:dbl)
                    n675 = Index Array(array=w1330, index (row)=0 ("disabled index (row)"), index (col)=3 ("disabled index (col)")) -> (element=w1327:dbl)
                    n676 = Index Array(array=w1330, index (col)=3 ("disabled index (col)")) -> (element=w1325:dbl[])  [unwired: 1 in]
                    n677 = shared-variable ".\\control setting.lvlib\\SpeedLimit"() -> (w1319:dbl[])  [unwired: 1 in, 1 out]
                    n678 = call "fuzzy rules.vi"("error"=w1327, "set point"=w1326, "error array"=w1325, "X"=w1311, "error in (no error)"=w1324, "fuzzy system in"=w1328) -> ("last error"=w1306:dbl, "slope"=w1303:dbl, "output value"=w1304:dbl, "error out"=w1313:errorcluster)  [unwired: 9 in, 1 out]
                    "last error 04" <- w1306
                    "slope D04" <- w1303
                    n679 = property on="SPEED 04" class="DigNum (strict)"() -> ("Value"=w1305:dbl)  [unwired: 2 in, 2 out]
                    n680 = Index Array(array=w1319, index #1=0 ("index")) -> (element #1=w1317:dbl, element #2=w1316:dbl)  [unwired: 1 in]
                    n681 = Build Array(4) -> (w1321:i32[])
                    n682 = call "speed to disc.vi"("task in digital"=w1323, "data"=w1321, "speed change"=w1304, "change limit"=0.025, "speed max limit"=w1317, "speed min limit"=w1316, "speed in"=w1305, "wait time"=u32 1000, "task inAnalog"=w1314, "error in (no error)"=w1313) -> ("inc"=w1309:bool, "dec"=w1310:bool, "no change"=w1308:bool, "error out"=w1312:errorcluster)  [unwired: 13 in, 1 out]
                    "no change D04" <- w1308
                    "increase D04" <- w1309
                    "decrease D04" <- w1310
                    n683 = Bundle("dec"=w1310, "inc"=w1309, "no change"=w1308, "sudden change"=w1307, "last error"=w1306, "Value"=w1305, "output value"=w1304, "slope"=w1303) -> (w1302:T34)  [unwired: 1 in]
                    n684 = shared-variable ".\\control setting.lvlib\\ControlInfoD04"(w1302) -> ()  [unwired: 1 in, 1 out]
                  }
                }
              }
              frame #3 {
                n685 = shared-variable ".\\D04.lvlib\\change D04"(w1336) -> ()  [unwired: 1 in, 1 out]
              }
            }
          }
        }
      }
      frame #4 {
        n686 = property on="DISC 05" class="Bool (strict)"() -> ("Value"=w1349:bool)  [unwired: 2 in, 2 out]
        n687 = property on="AUTO/MAN 05" class="Bool (strict)"() -> ("Value"=w1348:bool)  [unwired: 2 in, 2 out]
        n688 = And(x=w1348, y=w1349) -> (x .and. y?=w1347:bool)
        n689 = case shown="True" w1347 {
          tunnel: w1352 -> [w1356 w1394]
          tunnel: w1351 -> [w1359 w1393]
          tunnel: w1350 -> [w1355 w1385]
          tunnel: w1353 -> [w1357 w1381]
          tunnel: w1354 -> [w1358 w1379]
          tunnel: [w1359 w1377] -> w1343
          tunnel: [w1358 w1375] -> w1346
          tunnel: [w1357 w1373] -> w1345
          tunnel: [w1356 w1371] -> w1344
          tunnel: [w1355 w1369] -> w1342
          frame False {
          }
          frame True {
            n690 = flat-sequence {
              tunnel: w1394 -> [w1409]
              tunnel: w1393 -> [w1410]
              tunnel: w1385 -> [w1411]
              tunnel: [w1411] -> w1392
              tunnel: [w1410] -> w1391
              tunnel: [w1409] -> w1390
              tunnel: [w1395] -> w1384
              tunnel: [w1399] -> w1382
              tunnel: w1381 -> [w1399]
              tunnel: [w1398] -> w1380
              tunnel: w1379 -> [w1398]
              tunnel: [w1395] -> w1367
              tunnel: [w1421] -> w1389
              tunnel: [w1415] -> w1388
              tunnel: [w1427] -> w1387
              tunnel: [w1414] -> w1386
              tunnel: w1392 -> [w1414]
              tunnel: w1391 -> [w1429]
              tunnel: w1390 -> [w1415]
              tunnel: w1384 -> [w1418]
              tunnel: [w1416] -> w1383
              tunnel: w1382 -> [w1416]
              tunnel: w1380 -> [w1417]
              tunnel: [w1417] -> w1378
              tunnel: [w1417] -> w1376
              tunnel: [w1416] -> w1374
              tunnel: [w1415] -> w1372
              tunnel: [w1414] -> w1370
              tunnel: [w1413] -> w1368
              tunnel: w1367 -> [w1413]
              tunnel: [w1412] -> w1360
              tunnel: w1389 -> [w1447]
              tunnel: w1388 -> [w1445]
              tunnel: w1387 -> [w1446]
              tunnel: w1386 -> [w1444]
              tunnel: w1383 -> [w1443]
              tunnel: w1378 -> [w1442]
              tunnel: w1376 -> [w1440]
              tunnel: w1374 -> [w1439]
              tunnel: w1372 -> [w1438]
              tunnel: w1370 -> [w1437]
              tunnel: w1368 -> [w1436]
              tunnel: [w1441] -> w1366
              tunnel: [w1440] -> w1365
              tunnel: [w1439] -> w1364
              tunnel: [w1438] -> w1363
              tunnel: [w1437] -> w1362
              tunnel: [w1435] -> w1361
              tunnel: w1360 -> [w1434]
              tunnel: [w1486] -> w1369
              tunnel: [w1487] -> w1371
              tunnel: [w1488] -> w1373
              tunnel: [w1489] -> w1375
              tunnel: [w1490] -> w1377
              tunnel: w1366 -> [w1490]
              tunnel: w1365 -> [w1489]
              tunnel: w1364 -> [w1488]
              tunnel: w1363 -> [w1487]
              tunnel: w1362 -> [w1486]
              tunnel: w1361 -> [w1485]
              frame #0 {
                n691 = shared-variable ".\\control setting.lvlib\\SetPoints"() -> (w1404:dbl[])  [unwired: 1 in, 1 out]
                n692 = property on="2D array out" class="Arr (strict)"() -> ("Value"=w1408:dbl[][])  [unwired: 2 in, 2 out]
                n693 = property on="speed  min 05" class="Bool (strict)"() -> ("Value"=w1401:bool)  [unwired: 2 in, 2 out]
                n694 = property on="speed max 05" class="Bool (strict)"() -> ("Value"=w1400:bool)  [unwired: 2 in, 2 out]
                n695 = property on="no change D05" class="Bool (strict)"() -> ("Value"=w1397:bool)  [unwired: 2 in, 2 out]
                n696 = shared-variable ".\\control setting.lvlib\\ErrorThr"() -> (w1396:dbl)  [unwired: 1 in, 1 out]
                n697 = Index Array(array=w1408, index (row)=0, index (col)=4 ("disabled index (col)")) -> (element=w1403:dbl)
                n698 = Index Array(array=w1404, index=4) -> (element=w1402:dbl)
                n699 = call "sudden change.vi"("error in"=w1403, "set point"=w1402, "speed min"=w1401, "speed max"=w1400, "no change"=w1397, "sudden threshould"=w1396) -> ("sudden change"=w1395:bool)  [unwired: 13 in]
                "sudden change D05" <- w1395
              }
              frame #1 {
                # "D26 Tick count to reach the pulse time (defult : 5min)"
                n700 = Boolean To (0,1)(Boolean=w1418) -> (0, 1=w1422:i16)
                n701 = shared-variable ".\\control setting.lvlib\\PlsePeriod"() -> (w1425:i16)  [unwired: 1 in, 1 out]
                n702 = Build Array(w1422) -> (w1423:i16[])
                n703 = call-poly <vilib>:"Basic Level Trigger Detection.vi"("signal in"=w1423, "level"=0.5) -> ("trigger detected?"=w1419:bool)  [unwired: 11 in, 2 out]
                n704 = call "Elapsed Time13"("Time Target (s)"=w1425, "Reset"=w1419, "error in (no error)"=w1429) -> ("Elapsed Time (s)"=w1420:dbl, "error out"=w1428:errorcluster)  [unwired: 9 in, 6 out]
                n705 = In Range and Coerce(upper limit=10.0, x=w1420, lower limit=0.1) -> (In Range?=w1412:bool)  [unwired: 1 out]
                n706 = Boolean To (0,1)(Boolean=w1412) -> (0, 1=w1426:i16)
                n707 = Build Array(w1426) -> (w1433:i16[])
                n708 = call-poly <vilib>:"Basic Level Trigger Detection.vi"("signal in"=w1433, "level"=0.5, "error in (no error)"=w1428) -> ("trigger detected?"=w1421:bool, "error out"=w1427:errorcluster)  [unwired: 10 in, 1 out]
              }
              frame #2 {
                n709 = case shown="True" w1447 {
                  tunnel: w1445 -> [_ w1477]
                  tunnel: w1446 -> [w1449 w1483]
                  tunnel: [w1449 w1461] -> w1441
                  tunnel: w1444 -> [_ w1460]
                  tunnel: w1443 -> [_ w1472]
                  tunnel: w1442 -> [_ w1463]
                  tunnel: w1436 -> [_ w1456]
                  tunnel: [w1448 w1450] -> w1435
                  tunnel: w1434 -> [w1448 w1450]
                  frame False {
                  }
                  frame True {
                    n710 = property on="2D array out" class="Arr (strict)"(error in=w1483) -> (error out=w1473:errorcluster, "Value"=w1479:dbl[][])  [unwired: 1 in, 1 out]
                    n711 = shared-variable ".\\control setting.lvlib\\SetPoints"() -> (w1481:dbl[])  [unwired: 1 in, 1 out]
                    n712 = Index Array(array=w1481, index=4) -> (element=w1475:dbl)
                    n713 = Index Array(array=w1479, index (row)=0 ("disabled index (row)"), index (col)=4 ("disabled index (col)")) -> (element=w1476:dbl)
                    n714 = Index Array(array=w1479, index (col)=4 ("disabled index (col)")) -> (element=w1474:dbl[])  [unwired: 1 in]
                    n715 = shared-variable ".\\control setting.lvlib\\SpeedLimit"() -> (w1468:dbl[])  [unwired: 1 in, 1 out]
                    n716 = call "fuzzy rules.vi"("error"=w1476, "set point"=w1475, "error array"=w1474, "X"=w1460, "error in (no error)"=w1473, "fuzzy system in"=w1477) -> ("last error"=w1455:dbl, "slope"=w1452:dbl, "output value"=w1453:dbl, "error out"=w1462:errorcluster)  [unwired: 9 in, 1 out]
                    "last error 05" <- w1455
                    "slope D05" <- w1452
                    n717 = property on="SPEED 05" class="DigNum (strict)"() -> ("Value"=w1454:dbl)  [unwired: 2 in, 2 out]
                    n718 = Index Array(array=w1468, index #1=0 ("index")) -> (element #1=w1466:dbl, element #2=w1465:dbl)  [unwired: 1 in]
                    n719 = Build Array(5) -> (w1470:i32[])
                    n720 = call "speed to disc.vi"("task in digital"=w1472, "data"=w1470, "speed change"=w1453, "change limit"=0.025, "speed max limit"=w1466, "speed min limit"=w1465, "speed in"=w1454, "wait time"=u32 1000, "task inAnalog"=w1463, "error in (no error)"=w1462) -> ("inc"=w1458:bool, "dec"=w1459:bool, "no change"=w1457:bool, "error out"=w1461:errorcluster)  [unwired: 13 in, 1 out]
                    "decrease D05" <- w1459
                    "no change D05" <- w1457
                    "increase D05" <- w1458
                    n721 = Bundle("dec"=w1459, "inc"=w1458, "no change"=w1457, "sudden change"=w1456, "last error"=w1455, "Value"=w1454, "output value"=w1453, "slope"=w1452) -> (w1451:T34)  [unwired: 1 in]
                    n722 = shared-variable ".\\control setting.lvlib\\ControlInfoD05"(w1451) -> ()  [unwired: 1 in, 1 out]
                  }
                }
              }
              frame #3 {
                n723 = shared-variable ".\\D05.lvlib\\change D05"(w1485) -> ()  [unwired: 1 in, 1 out]
              }
            }
          }
        }
      }
      frame #5 {
        n724 = property on="DISC 06" class="Bool (strict)"() -> ("Value"=w1494:bool)  [unwired: 2 in, 2 out]
        n725 = property on="AUTO/MAN 06" class="Bool (strict)"() -> ("Value"=w1493:bool)  [unwired: 2 in, 2 out]
        n726 = And(x=w1493, y=w1494) -> (x .and. y?=w1492:bool)
        n727 = case shown="True" w1492 {
          tunnel: w1497 -> [w1501 w1539]
          tunnel: w1496 -> [w1504 w1538]
          tunnel: w1495 -> [w1500 w1530]
          tunnel: w1498 -> [w1502 w1526]
          tunnel: w1499 -> [w1503 w1524]
          tunnel: [w1504 w1522] -> w1491
          tunnel: [w1503 w1520] -> _
          tunnel: [w1502 w1518] -> _
          tunnel: [w1501 w1516] -> _
          tunnel: [w1500 w1514] -> _
          frame False {
          }
          frame True {
            n728 = flat-sequence {
              tunnel: w1539 -> [w1554]
              tunnel: w1538 -> [w1555]
              tunnel: w1530 -> [w1556]
              tunnel: [w1556] -> w1537
              tunnel: [w1555] -> w1536
              tunnel: [w1554] -> w1535
              tunnel: [w1540] -> w1529
              tunnel: [w1544] -> w1527
              tunnel: w1526 -> [w1544]
              tunnel: [w1543] -> w1525
              tunnel: w1524 -> [w1543]
              tunnel: [w1540] -> w1512
              tunnel: [w1566] -> w1534
              tunnel: [w1560] -> w1533
              tunnel: [w1572] -> w1532
              tunnel: [w1559] -> w1531
              tunnel: w1537 -> [w1559]
              tunnel: w1536 -> [w1574]
              tunnel: w1535 -> [w1560]
              tunnel: w1529 -> [w1563]
              tunnel: [w1561] -> w1528
              tunnel: w1527 -> [w1561]
              tunnel: w1525 -> [w1562]
              tunnel: [w1562] -> w1523
              tunnel: [w1562] -> w1521
              tunnel: [w1561] -> w1519
              tunnel: [w1560] -> w1517
              tunnel: [w1559] -> w1515
              tunnel: [w1558] -> w1513
              tunnel: w1512 -> [w1558]
              tunnel: [w1557] -> w1505
              tunnel: w1534 -> [w1592]
              tunnel: w1533 -> [w1590]
              tunnel: w1532 -> [w1591]
              tunnel: w1531 -> [w1589]
              tunnel: w1528 -> [w1588]
              tunnel: w1523 -> [w1587]
              tunnel: w1521 -> [w1585]
              tunnel: w1519 -> [w1584]
              tunnel: w1517 -> [w1583]
              tunnel: w1515 -> [w1582]
              tunnel: w1513 -> [w1581]
              tunnel: [w1586] -> w1511
              tunnel: [w1585] -> w1510
              tunnel: [w1584] -> w1509
              tunnel: [w1583] -> w1508
              tunnel: [w1582] -> w1507
              tunnel: [w1580] -> w1506
              tunnel: w1505 -> [w1579]
              tunnel: [w1631] -> w1514
              tunnel: [w1632] -> w1516
              tunnel: [w1633] -> w1518
              tunnel: [w1634] -> w1520
              tunnel: [w1635] -> w1522
              tunnel: w1511 -> [w1635]
              tunnel: w1510 -> [w1634]
              tunnel: w1509 -> [w1633]
              tunnel: w1508 -> [w1632]
              tunnel: w1507 -> [w1631]
              tunnel: w1506 -> [w1630]
              frame #0 {
                n729 = shared-variable ".\\control setting.lvlib\\SetPoints"() -> (w1549:dbl[])  [unwired: 1 in, 1 out]
                n730 = property on="2D array out" class="Arr (strict)"() -> ("Value"=w1553:dbl[][])  [unwired: 2 in, 2 out]
                n731 = property on="speed  min 06" class="Bool (strict)"() -> ("Value"=w1546:bool)  [unwired: 2 in, 2 out]
                n732 = property on="speed max 06" class="Bool (strict)"() -> ("Value"=w1545:bool)  [unwired: 2 in, 2 out]
                n733 = property on="no change D06" class="Bool (strict)"() -> ("Value"=w1542:bool)  [unwired: 2 in, 2 out]
                n734 = shared-variable ".\\control setting.lvlib\\ErrorThr"() -> (w1541:dbl)  [unwired: 1 in, 1 out]
                n735 = Index Array(array=w1553, index (row)=0, index (col)=5 ("disabled index (col)")) -> (element=w1548:dbl)
                n736 = Index Array(array=w1549, index=5) -> (element=w1547:dbl)
                n737 = call "sudden change.vi"("error in"=w1548, "set point"=w1547, "speed min"=w1546, "speed max"=w1545, "no change"=w1542, "sudden threshould"=w1541) -> ("sudden change"=w1540:bool)  [unwired: 13 in]
                "sudden change D06" <- w1540
              }
              frame #1 {
                # "D26 Tick count to reach the pulse time (defult : 5min)"
                n738 = Boolean To (0,1)(Boolean=w1563) -> (0, 1=w1567:i16)
                n739 = shared-variable ".\\control setting.lvlib\\PlsePeriod"() -> (w1570:i16)  [unwired: 1 in, 1 out]
                n740 = Build Array(w1567) -> (w1568:i16[])
                n741 = call-poly <vilib>:"Basic Level Trigger Detection.vi"("signal in"=w1568, "level"=0.5) -> ("trigger detected?"=w1564:bool)  [unwired: 11 in, 2 out]
                n742 = call "Elapsed Time14"("Time Target (s)"=w1570, "Reset"=w1564, "error in (no error)"=w1574) -> ("Elapsed Time (s)"=w1565:dbl, "error out"=w1573:errorcluster)  [unwired: 9 in, 6 out]
                n743 = In Range and Coerce(upper limit=10.0, x=w1565, lower limit=0.1) -> (In Range?=w1557:bool)  [unwired: 1 out]
                n744 = Boolean To (0,1)(Boolean=w1557) -> (0, 1=w1571:i16)
                n745 = Build Array(w1571) -> (w1578:i16[])
                n746 = call-poly <vilib>:"Basic Level Trigger Detection.vi"("signal in"=w1578, "level"=0.5, "error in (no error)"=w1573) -> ("trigger detected?"=w1566:bool, "error out"=w1572:errorcluster)  [unwired: 10 in, 1 out]
              }
              frame #2 {
                n747 = case shown="True" w1592 {
                  tunnel: w1590 -> [_ w1622]
                  tunnel: w1591 -> [w1594 w1628]
                  tunnel: [w1594 w1606] -> w1586
                  tunnel: w1589 -> [_ w1605]
                  tunnel: w1588 -> [_ w1617]
                  tunnel: w1587 -> [_ w1608]
                  tunnel: w1581 -> [_ w1601]
                  tunnel: [w1593 w1595] -> w1580
                  tunnel: w1579 -> [w1593 w1595]
                  frame False {
                  }
                  frame True {
                    n748 = property on="2D array out" class="Arr (strict)"(error in=w1628) -> (error out=w1618:errorcluster, "Value"=w1624:dbl[][])  [unwired: 1 in, 1 out]
                    n749 = shared-variable ".\\control setting.lvlib\\SetPoints"() -> (w1626:dbl[])  [unwired: 1 in, 1 out]
                    n750 = Index Array(array=w1626, index=5) -> (element=w1620:dbl)
                    n751 = Index Array(array=w1624, index (row)=0 ("disabled index (row)"), index (col)=5 ("disabled index (col)")) -> (element=w1621:dbl)
                    n752 = Index Array(array=w1624, index (col)=5 ("disabled index (col)")) -> (element=w1619:dbl[])  [unwired: 1 in]
                    n753 = shared-variable ".\\control setting.lvlib\\SpeedLimit"() -> (w1613:dbl[])  [unwired: 1 in, 1 out]
                    n754 = call "fuzzy rules.vi"("error"=w1621, "set point"=w1620, "error array"=w1619, "X"=w1605, "error in (no error)"=w1618, "fuzzy system in"=w1622) -> ("last error"=w1600:dbl, "slope"=w1597:dbl, "output value"=w1598:dbl, "error out"=w1607:errorcluster)  [unwired: 9 in, 1 out]
                    "last error 06" <- w1600
                    "slope D06" <- w1597
                    n755 = property on="SPEED 06" class="DigNum (strict)"() -> ("Value"=w1599:dbl)  [unwired: 2 in, 2 out]
                    n756 = Index Array(array=w1613, index #1=0 ("index")) -> (element #1=w1611:dbl, element #2=w1610:dbl)  [unwired: 1 in]
                    n757 = Build Array(6) -> (w1615:i32[])
                    n758 = call "speed to disc.vi"("task in digital"=w1617, "data"=w1615, "speed change"=w1598, "change limit"=0.025, "speed max limit"=w1611, "speed min limit"=w1610, "speed in"=w1599, "wait time"=u32 1000, "task inAnalog"=w1608, "error in (no error)"=w1607) -> ("inc"=w1603:bool, "dec"=w1604:bool, "no change"=w1602:bool, "error out"=w1606:errorcluster)  [unwired: 13 in, 1 out]
                    "decrease D06" <- w1604
                    "no change D06" <- w1602
                    "increase D06" <- w1603
                    n759 = Bundle("dec"=w1604, "inc"=w1603, "no change"=w1602, "sudden change"=w1601, "last error"=w1600, "Value"=w1599, "output value"=w1598, "slope"=w1597) -> (w1596:T34)  [unwired: 1 in]
                    n760 = shared-variable ".\\control setting.lvlib\\ControlInfoD06"(w1596) -> ()  [unwired: 1 in, 1 out]
                  }
                }
              }
              frame #3 {
                n761 = shared-variable ".\\D06.lvlib\\change D06"(w1630) -> ()  [unwired: 1 in, 1 out]
              }
            }
          }
        }
      }
    }
    n762 = Wait (ms)(milliseconds to wait=u32 10) -> ()  [unwired: 1 out]
  }
  n763 = while {
    tunnel: w123 -> [w2297]
    tunnel: w118 -> [w2296]
    tunnel: [w2295] -> w117
    tunnel: w116 -> [w2294]
    tunnel: w114 -> [w2293]
    tunnel: w112 -> [w2292]
    tunnel: w109 -> [w2290]
    tunnel: w108 -> [w2289]
    shift-right: [w2287] -> _
    shift-left: w106 -> [w2288]
    shift-right: [w2285] -> _
    shift-left: w101 -> [w2286]
    shift-right: [w2283] -> _
    shift-left: w99 -> [w2284]
    shift-right: [w2281] -> _
    shift-left: w92 -> [w2282]
    shift-right: [w2277] -> _
    shift-left: w89 -> [w2280]
    shift-right: [w2276] -> _
    shift-left: w83 -> [w2278]
    shift-right: [w2275] -> _
    shift-left: w84 -> [w2279]
    shift-right: [w2273] -> _
    shift-left: w80 -> [w2274]
    tunnel: w74 -> [w2021]
    tunnel: w51 -> [w2019]
    tunnel: w69 -> [w2012]
    tunnel: w68 -> [w2003]
    tunnel: w67 -> [w1989]
    tunnel: w49 -> [w1791]
    tunnel: w47 -> [w1764]
    shift-right: [w1664] -> _
    shift-left: w44 -> [w1700]
    stop <- FALSE stop-if-true
    n764 = Wait (ms)(milliseconds to wait=u32 5) -> ()  [unwired: 1 out]
    n765 = flat-sequence {
      tunnel: w2282 -> [w2386]
      tunnel: w2284 -> [w2401]
      tunnel: w2286 -> [w2402]
      tunnel: w2288 -> [w2403]
      tunnel: w2289 -> [w2404]
      tunnel: w2290 -> [w2405]
      tunnel: w2292 -> [w2406]
      tunnel: w2293 -> [w2407]
      tunnel: w2297 -> [w2408]
      tunnel: w2294 -> [w2409]
      tunnel: w2296 -> [w2410]
      tunnel: [w2410] -> w2271
      tunnel: [w2409] -> w2270
      tunnel: [w2408] -> w2269
      tunnel: [w2407] -> w2268
      tunnel: [w2406] -> w2267
      tunnel: [w2405] -> w2266
      tunnel: [w2404] -> w2265
      tunnel: [w2403] -> w2264
      tunnel: [w2402] -> w2263
      tunnel: [w2401] -> w2262
      tunnel: [w2390] -> w2261
      tunnel: [w2389] -> w2260
      tunnel: [w2388] -> w2259
      tunnel: [w2387] -> w2258
      tunnel: [w2386] -> w2257
      tunnel: w2280 -> [w2339]
      tunnel: [w2373] -> w2256
      tunnel: [w2372] -> w2255
      tunnel: [w2371] -> w2254
      tunnel: [w2370] -> w2253
      tunnel: w2279 -> [w2338]
      tunnel: w2278 -> [w2337]
      tunnel: [w2347] -> w2252
      tunnel: [w2346] -> w2251
      tunnel: [w2345] -> w2250
      tunnel: [w2344] -> w2249
      tunnel: [w2343] -> w2248
      tunnel: [w2342] -> w2247
      tunnel: [w2341] -> w2246
      tunnel: [w2340] -> w2245
      tunnel: [w2339] -> w2244
      tunnel: [w2338] -> w2243
      tunnel: [w2337] -> w2242
      tunnel: w2274 -> [w2325]
      tunnel: [w2325] -> w2241
      tunnel: [w2324] -> w2240
      tunnel: [w2323] -> w2239
      tunnel: [w2322] -> w2238
      tunnel: [w2321] -> w2237
      tunnel: [w2320] -> w2022
      tunnel: w2021 -> [w2320]
      tunnel: [w2319] -> w2020
      tunnel: w2019 -> [w2319]
      tunnel: [w2318] -> w2013
      tunnel: w2012 -> [w2318]
      tunnel: w2003 -> [w2317]
      tunnel: [w2317] -> w2002
      tunnel: [w2316] -> w1990
      tunnel: w1989 -> [w2316]
      tunnel: [w2315] -> w1792
      tunnel: w1791 -> [w2315]
      tunnel: w1764 -> [w2314]
      tunnel: [w2314] -> w1737
      tunnel: w1700 -> [w2298]
      tunnel: [w2302] -> w1699
      tunnel: [w2301] -> w1698
      tunnel: [w2300] -> w1697
      tunnel: [w2299] -> w1696
      tunnel: [w2298] -> w1694
      tunnel: w2271 -> [w2483]
      tunnel: [w2483] -> w1830
      tunnel: w2270 -> [w2482]
      tunnel: [w2482] -> w1829
      tunnel: w2269 -> [w2481]
      tunnel: [w2481] -> w1828
      tunnel: w2268 -> [w2480]
      tunnel: [w2480] -> w1827
      tunnel: w2267 -> [w2479]
      tunnel: [w2479] -> w1826
      tunnel: w2266 -> [w2478]
      tunnel: [w2478] -> w1825
      tunnel: w2265 -> [w2477]
      tunnel: [w2477] -> w1824
      tunnel: w2264 -> [w2476]
      tunnel: [w2476] -> w1823
      tunnel: w2263 -> [w2475]
      tunnel: [w2475] -> w1822
      tunnel: w2262 -> [w2474]
      tunnel: [w2474] -> w1821
      tunnel: w2261 -> [w2451]
      tunnel: w2260 -> [w2450]
      tunnel: w2259 -> [w2449]
      tunnel: w2258 -> [w2452]
      tunnel: w2257 -> [w2473]
      tunnel: [w2473] -> w1820
      tunnel: w2256 -> [w2459]
      tunnel: w2255 -> [w2457]
      tunnel: w2254 -> [w2458]
      tunnel: w2253 -> [w2460]
      tunnel: w2252 -> [w2462]
      tunnel: w2251 -> [w2464]
      tunnel: w2250 -> [w2463]
      tunnel: w2249 -> [w2461]
      tunnel: w2248 -> [w2453]
      tunnel: w2247 -> [w2456]
      tunnel: w2246 -> [w2455]
      tunnel: w2245 -> [w2454]
      tunnel: w2244 -> [w2472]
      tunnel: [w2472] -> w1819
      tunnel: w2243 -> [w2471]
      tunnel: [w2471] -> w1818
      tunnel: w2242 -> [w2470]
      tunnel: [w2470] -> w1817
      tunnel: w2241 -> [w2469]
      tunnel: [w2469] -> w1816
      tunnel: w2240 -> [w2468]
      tunnel: w2239 -> [w2467]
      tunnel: w2238 -> [w2466]
      tunnel: w2237 -> [w2465]
      tunnel: w2022 -> [w2413]
      tunnel: w2020 -> [w2433]
      tunnel: [w2433] -> w1815
      tunnel: w2013 -> [w2432]
      tunnel: [w2432] -> w1814
      tunnel: [w2431] -> w1813
      tunnel: w2002 -> [w2431]
      tunnel: w1990 -> [w2430]
      tunnel: [w2430] -> w1812
      tunnel: w1792 -> [w2429]
      tunnel: [w2429] -> w1765
      tunnel: [w2428] -> w1738
      tunnel: w1737 -> [w2428]
      tunnel: w1699 -> [w2424]
      tunnel: w1698 -> [w2423]
      tunnel: w1697 -> [w2422]
      tunnel: w1696 -> [w2421]
      tunnel: [w2420] -> w1695
      tunnel: w1694 -> [w2420]
      tunnel: [w2418] -> w1656
      tunnel: [w2414] -> w1655
      tunnel: ["get_circels" ("function name")] -> w1654
      tunnel: [w2416] -> w1653
      tunnel: [w2413] -> w1643
      tunnel: [w2412] -> w1642
      tunnel: [w2598] -> w2070
      tunnel: [w2659] -> w2068
      tunnel: [w2600] -> w2066
      tunnel: [w2658] -> w2064
      tunnel: [w2657] -> w2062
      tunnel: [w2656] -> w2060
      tunnel: [w2655] -> w2058
      tunnel: [w2654] -> w2056
      tunnel: [w2653] -> w2054
      tunnel: [w2647] -> w2052
      tunnel: [w2642] -> w2050
      tunnel: [w2630] -> w2048
      tunnel: [w2629] -> w2046
      tunnel: [w2623] -> w2044
      tunnel: [w2531] -> w2042
      tunnel: [w2596] -> w2026
      tunnel: [w2602] -> w2023
      tunnel: [w2595] -> w2014
      tunnel: [w2594] -> w2004
      tunnel: [w2593] -> w1991
      tunnel: [w2592] -> w1984
      tunnel: w1812 -> [w2592]
      tunnel: w1813 -> [w2593]
      tunnel: w1814 -> [w2594]
      tunnel: w1815 -> [w2595]
      tunnel: w1816 -> [w2625]
      tunnel: w1817 -> [w2632]
      tunnel: w1818 -> [w2631]
      tunnel: w1819 -> [w2644]
      tunnel: w1820 -> [w2651]
      tunnel: w1821 -> [w2653]
      tunnel: w1822 -> [w2654]
      tunnel: w1823 -> [w2655]
      tunnel: w1824 -> [w2656]
      tunnel: w1825 -> [w2657]
      tunnel: w1826 -> [w2658]
      tunnel: w1827 -> [w2659]
      tunnel: w1828 -> [w2599]
      tunnel: w1829 -> [w2601]
      tunnel: w1830 -> [w2600]
      tunnel: [w2555] -> w1766
      tunnel: w1765 -> [w2555]
      tunnel: [w2554] -> w1739
      tunnel: w1738 -> [w2554]
      tunnel: w1695 -> [w2538]
      tunnel: [w2537] -> w1693
      tunnel: w1656 -> [w2530]
      tunnel: w1655 -> [w2536]
      tunnel: w1654 -> [w2535]
      tunnel: w1653 -> [w2534]
      tunnel: w1643 -> [_]
      tunnel: w1642 -> [w2532]
      tunnel: w2070 -> [w2660]
      tunnel: [w2660] -> w2069
      tunnel: w2068 -> [w2694]
      tunnel: [w2694] -> w2067
      tunnel: w2066 -> [w2693]
      tunnel: [w2693] -> w2065
      tunnel: w2064 -> [w2692]
      tunnel: [w2692] -> w2063
      tunnel: w2062 -> [w2691]
      tunnel: [w2691] -> w2061
      tunnel: w2060 -> [w2690]
      tunnel: [w2690] -> w2059
      tunnel: w2058 -> [w2689]
      tunnel: [w2689] -> w2057
      tunnel: w2056 -> [w2688]
      tunnel: [w2688] -> w2055
      tunnel: w2054 -> [w2687]
      tunnel: [w2687] -> w2053
      tunnel: w2052 -> [w2686]
      tunnel: [w2686] -> w2051
      tunnel: w2050 -> [w2685]
      tunnel: [w2685] -> w2049
      tunnel: w2048 -> [w2684]
      tunnel: [w2684] -> w2047
      tunnel: w2046 -> [w2683]
      tunnel: [w2683] -> w2045
      tunnel: w2044 -> [w2682]
      tunnel: [w2682] -> w2043
      tunnel: w2042 -> [w2669]
      tunnel: w2026 -> [w2680]
      tunnel: [w2680] -> w2025
      tunnel: w2023 -> [w2661]
      tunnel: [w2678] -> w2015
      tunnel: w2014 -> [w2678]
      tunnel: [w2677] -> w2005
      tunnel: w2004 -> [w2677]
      tunnel: [w2676] -> w1992
      tunnel: w1991 -> [w2676]
      tunnel: [w2675] -> w1985
      tunnel: w1984 -> [w2675]
      tunnel: [w2674] -> w1938
      tunnel: [w2664] -> w1767
      tunnel: w1766 -> [w2664]
      tunnel: [w2663] -> w1740
      tunnel: w1739 -> [w2663]
      tunnel: w1693 -> [w2662]
      tunnel: [w2662] -> w1692
      tunnel: w2069 -> [w2746]
      tunnel: [w2746] -> w2041
      tunnel: w2067 -> [w2745]
      tunnel: [w2745] -> w2040
      tunnel: w2065 -> [w2744]
      tunnel: [w2744] -> w2039
      tunnel: w2063 -> [w2743]
      tunnel: [w2743] -> w2038
      tunnel: w2061 -> [w2742]
      tunnel: [w2742] -> w2037
      tunnel: w2059 -> [w2741]
      tunnel: [w2741] -> w2036
      tunnel: w2057 -> [w2740]
      tunnel: [w2739] -> w2035
      tunnel: w2055 -> [w2738]
      tunnel: [w2737] -> w2034
      tunnel: w2053 -> [w2736]
      tunnel: [w2735] -> w2033
      tunnel: [w2723] -> w2032
      tunnel: [w2722] -> w2031
      tunnel: w2051 -> [w2722]
      tunnel: w2049 -> [w2721]
      tunnel: [w2721] -> w2030
      tunnel: [w2720] -> w2029
      tunnel: w2047 -> [w2720]
      tunnel: w2045 -> [w2719]
      tunnel: [w2719] -> w2028
      tunnel: [w2718] -> w2027
      tunnel: w2043 -> [w2718]
      tunnel: w2025 -> [w2717]
      tunnel: [w2716] -> w2024
      tunnel: [w2715] -> w2016
      tunnel: w2015 -> [w2715]
      tunnel: [w2714] -> w2006
      tunnel: w2005 -> [w2714]
      tunnel: [w2713] -> w1993
      tunnel: w1992 -> [w2713]
      tunnel: [w2712] -> w1986
      tunnel: w1985 -> [w2712]
      tunnel: w1938 -> [w2711]
      tunnel: [w2709] -> w1840
      tunnel: [w2707] -> w1835
      tunnel: [w2706] -> w1768
      tunnel: w1767 -> [w2706]
      tunnel: [w2705] -> w1741
      tunnel: w1740 -> [w2705]
      tunnel: w1692 -> [w2704]
      tunnel: [w2704] -> w1691
      tunnel: [w2850] -> w2187
      tunnel: [w2849] -> w2185
      tunnel: [w2848] -> w2183
      tunnel: [w2847] -> w2181
      tunnel: [w2846] -> w2179
      tunnel: [w2845] -> w2177
      tunnel: [w2836] -> w2175
      tunnel: [w2844] -> w2173
      tunnel: [w2843] -> w2171
      tunnel: [w2842] -> w2169
      tunnel: [w2841] -> w2167
      tunnel: [w2840] -> w2165
      tunnel: [w2839] -> w2163
      tunnel: [w2838] -> w2161
      tunnel: [w2837] -> w2159
      tunnel: w2027 -> [w2837]
      tunnel: w2028 -> [w2838]
      tunnel: w2029 -> [w2839]
      tunnel: w2030 -> [w2840]
      tunnel: w2031 -> [w2841]
      tunnel: w2032 -> [w2842]
      tunnel: w2033 -> [w2843]
      tunnel: w2034 -> [w2844]
      tunnel: w2035 -> [w2836]
      tunnel: w2036 -> [w2845]
      tunnel: w2037 -> [w2846]
      tunnel: w2038 -> [w2847]
      tunnel: w2039 -> [w2848]
      tunnel: w2040 -> [w2849]
      tunnel: w2041 -> [w2850]
      tunnel: w2024 -> [w2828]
      tunnel: [w2825] -> w2017
      tunnel: w2016 -> [w2825]
      tunnel: [w2824] -> w2007
      tunnel: w2006 -> [w2824]
      tunnel: [w2823] -> w1994
      tunnel: w1993 -> [w2823]
      tunnel: [w2822] -> w1987
      tunnel: w1986 -> [w2822]
      tunnel: w1840 -> [w2821]
      tunnel: w1835 -> [w2820]
      tunnel: [w2818] -> w1834
      tunnel: [w2816] -> w1769
      tunnel: w1768 -> [w2816]
      tunnel: [w2815] -> w1742
      tunnel: w1741 -> [w2815]
      tunnel: w1691 -> [w2814]
      tunnel: [w2814] -> w1665
      tunnel: w2187 -> [w2964]
      tunnel: [w2964] -> w2186
      tunnel: w2185 -> [w2963]
      tunnel: [w2963] -> w2184
      tunnel: w2183 -> [w2962]
      tunnel: [w2962] -> w2182
      tunnel: w2181 -> [w2961]
      tunnel: [w2961] -> w2180
      tunnel: w2179 -> [w2960]
      tunnel: [w2960] -> w2178
      tunnel: w2177 -> [w2959]
      tunnel: [w2959] -> w2176
      tunnel: w2175 -> [w2958]
      tunnel: [w2958] -> w2174
      tunnel: w2173 -> [w2957]
      tunnel: [w2957] -> w2172
      tunnel: w2171 -> [w2956]
      tunnel: [w2956] -> w2170
      tunnel: w2169 -> [w2955]
      tunnel: [w2955] -> w2168
      tunnel: w2167 -> [w2954]
      tunnel: [w2954] -> w2166
      tunnel: w2165 -> [w2953]
      tunnel: [w2953] -> w2164
      tunnel: w2163 -> [w2952]
      tunnel: [w2952] -> w2162
      tunnel: w2161 -> [w2951]
      tunnel: [w2951] -> w2160
      tunnel: w2159 -> [w2950]
      tunnel: [w2950] -> w2158
      tunnel: [w2936] -> w2018
      tunnel: w2017 -> [w2936]
      tunnel: [w2948] -> w2008
      tunnel: w2007 -> [w2948]
      tunnel: [w2947] -> w1995
      tunnel: w1994 -> [w2947]
      tunnel: [w2946] -> w1988
      tunnel: w1987 -> [w2946]
      tunnel: w1834 -> [w2943]
      tunnel: [w2941] -> w1770
      tunnel: w1769 -> [w2941]
      tunnel: [w2940] -> w1743
      tunnel: w1742 -> [w2940]
      tunnel: [w2939] -> w1666
      tunnel: w1665 -> [w2939]
      tunnel: [w2938] -> w1663
      tunnel: [w2937] -> w1645
      tunnel: [w2932] -> w1636
      tunnel: w2186 -> [w3065]
      tunnel: w2184 -> [w3056]
      tunnel: w2182 -> [w3059]
      tunnel: [w3064] -> w1974
      tunnel: w2180 -> [w3063]
      tunnel: [w3063] -> w1973
      tunnel: [w3059] -> w1971
      tunnel: w2178 -> [w3062]
      tunnel: [w3062] -> w1969
      tunnel: w2176 -> [w3061]
      tunnel: [w3061] -> w1967
      tunnel: [w3060] -> w1965
      tunnel: w2174 -> [w3060]
      tunnel: [w3058] -> w1962
      tunnel: w2172 -> [w3058]
      tunnel: [w3057] -> w1960
      tunnel: w2170 -> [w3057]
      tunnel: [w3044] -> w1958
      tunnel: w2168 -> [w3055]
      tunnel: [w3055] -> w1957
      tunnel: [w3054] -> w1955
      tunnel: w2166 -> [w3054]
      tunnel: [w3053] -> w1953
      tunnel: w2164 -> [w3053]
      tunnel: w2162 -> [w3052]
      tunnel: [w3052] -> w1951
      tunnel: [w3051] -> w1949
      tunnel: w2160 -> [w3051]
      tunnel: w2158 -> [w3050]
      tunnel: [w3050] -> w1947
      tunnel: w2018 -> [w3049]
      tunnel: [w3048] -> w1945
      tunnel: w2008 -> [w3048]
      tunnel: [w3047] -> w1943
      tunnel: w1995 -> [w3047]
      tunnel: w1988 -> [w3046]
      tunnel: [w3046] -> w1941
      tunnel: [w3045] -> w1935
      tunnel: [w3040] -> w1771
      tunnel: w1770 -> [w3040]
      tunnel: [w3039] -> w1744
      tunnel: w1743 -> [w3039]
      tunnel: [w3038] -> w1667
      tunnel: w1666 -> [w3038]
      tunnel: w1663 -> [w3035]
      tunnel: w1645 -> [w3037]
      tunnel: [w3031] -> w1639
      tunnel: w1636 -> [w3030]
      tunnel: w1974 -> [w3069]
      tunnel: w1973 -> [w3101]
      tunnel: [w3101] -> w1972
      tunnel: w1971 -> [w3100]
      tunnel: [w3100] -> w1970
      tunnel: w1969 -> [w3099]
      tunnel: [w3099] -> w1968
      tunnel: w1967 -> [w3098]
      tunnel: [w3098] -> w1966
      tunnel: w1965 -> [w3097]
      tunnel: [w3097] -> w1964
      tunnel: [w3084] -> w1963
      tunnel: w1962 -> [w3096]
      tunnel: [w3096] -> w1961
      tunnel: w1960 -> [w3095]
      tunnel: [w3095] -> w1959
      tunnel: w1958 -> [w3070]
      tunnel: w1957 -> [w3094]
      tunnel: [w3094] -> w1956
      tunnel: w1955 -> [w3093]
      tunnel: [w3093] -> w1954
      tunnel: w1953 -> [w3092]
      tunnel: [w3092] -> w1952
      tunnel: w1951 -> [w3091]
      tunnel: [w3091] -> w1950
      tunnel: w1949 -> [w3090]
      tunnel: [w3090] -> w1948
      tunnel: w1947 -> [w3089]
      tunnel: [w3089] -> w1946
      tunnel: w1945 -> [w3088]
      tunnel: [w3088] -> w1944
      tunnel: w1943 -> [w3087]
      tunnel: [w3087] -> w1942
      tunnel: w1941 -> [w3086]
      tunnel: [w3086] -> w1940
      tunnel: [w3069] -> w1939
      tunnel: [w3083] -> w1936
      tunnel: w1935 -> [w3083]
      tunnel: [w3073] -> w1772
      tunnel: w1771 -> [w3073]
      tunnel: [w3072] -> w1745
      tunnel: w1744 -> [w3072]
      tunnel: [w3071] -> w1668
      tunnel: w1667 -> [w3071]
      tunnel: [w3068] -> w1644
      tunnel: w1639 -> [w3079]
      tunnel: [w3138] -> w2236
      tunnel: w1972 -> [w3137]
      tunnel: [w3137] -> w2235
      tunnel: w1970 -> [w3136]
      tunnel: [w3136] -> w2234
      tunnel: w1968 -> [w3135]
      tunnel: [w3135] -> w2233
      tunnel: w1966 -> [w3134]
      tunnel: [w3134] -> w2232
      tunnel: w1964 -> [w3132]
      tunnel: [w3131] -> w2231
      tunnel: w1963 -> [w3133]
      tunnel: w1961 -> [w3130]
      tunnel: [w3129] -> w2230
      tunnel: [w3127] -> w2229
      tunnel: w1959 -> [w3128]
      tunnel: [w3126] -> w2228
      tunnel: w1956 -> [w3126]
      tunnel: [w3125] -> w2227
      tunnel: w1954 -> [w3125]
      tunnel: [w3124] -> w2226
      tunnel: w1952 -> [w3124]
      tunnel: [w3123] -> w2225
      tunnel: w1950 -> [w3123]
      tunnel: w1948 -> [w3122]
      tunnel: [w3122] -> w2224
      tunnel: [w3121] -> w2223
      tunnel: w1946 -> [w3121]
      tunnel: [w3120] -> w2009
      tunnel: w1944 -> [w3120]
      tunnel: [w3119] -> w1996
      tunnel: w1942 -> [w3119]
      tunnel: [w3118] -> w1975
      tunnel: w1940 -> [w3118]
      tunnel: w1939 -> [w3138]
      tunnel: [w3117] -> w1937
      tunnel: w1936 -> [w3116]
      tunnel: [w3115] -> w1839
      tunnel: [w3114] -> w1773
      tunnel: w1772 -> [w3114]
      tunnel: [w3113] -> w1746
      tunnel: w1745 -> [w3113]
      tunnel: [w3112] -> w1669
      tunnel: w1668 -> [w3112]
      tunnel: w1644 -> [w3111]
      tunnel: w2236 -> [w3240]
      tunnel: [w3240] -> w2157
      tunnel: w2235 -> [w3239]
      tunnel: [w3239] -> w2155
      tunnel: w2234 -> [w3238]
      tunnel: [w3238] -> w2153
      tunnel: w2233 -> [w3237]
      tunnel: [w3237] -> w2151
      tunnel: w2232 -> [w3236]
      tunnel: [w3236] -> w2149
      tunnel: w2231 -> [w3213]
      tunnel: [w3213] -> w2147
      tunnel: w2230 -> [w3235]
      tunnel: [w3235] -> w2145
      tunnel: w2229 -> [w3234]
      tunnel: [w3234] -> w2143
      tunnel: w2228 -> [w3233]
      tunnel: [w3233] -> w2141
      tunnel: w2227 -> [w3232]
      tunnel: [w3232] -> w2139
      tunnel: w2226 -> [w3231]
      tunnel: [w3231] -> w2137
      tunnel: [w3230] -> w2135
      tunnel: w2225 -> [w3230]
      tunnel: [w3229] -> w2133
      tunnel: w2224 -> [w3229]
      tunnel: [w3228] -> w2131
      tunnel: w2223 -> [w3228]
      tunnel: [w3227] -> w2010
      tunnel: w2009 -> [w3227]
      tunnel: [w3226] -> w1997
      tunnel: w1996 -> [w3226]
      tunnel: [w3225] -> w1976
      tunnel: w1975 -> [w3225]
      tunnel: w1937 -> [w3224]
      tunnel: w1839 -> [w3212]
      tunnel: [w3211] -> w1833
      tunnel: [w3209] -> w1774
      tunnel: w1773 -> [w3209]
      tunnel: [w3208] -> w1747
      tunnel: w1746 -> [w3208]
      tunnel: [w3207] -> w1670
      tunnel: w1669 -> [w3207]
      tunnel: w2157 -> [w3351]
      tunnel: [w3351] -> w2156
      tunnel: w2155 -> [w3350]
      tunnel: [w3350] -> w2154
      tunnel: w2153 -> [w3349]
      tunnel: [w3349] -> w2152
      tunnel: w2151 -> [w3348]
      tunnel: [w3348] -> w2150
      tunnel: w2149 -> [w3347]
      tunnel: [w3347] -> w2148
      tunnel: w2147 -> [w3346]
      tunnel: [w3346] -> w2146
      tunnel: w2145 -> [w3345]
      tunnel: [w3345] -> w2144
      tunnel: w2143 -> [w3344]
      tunnel: [w3344] -> w2142
      tunnel: w2141 -> [w3343]
      tunnel: [w3343] -> w2140
      tunnel: w2139 -> [w3342]
      tunnel: [w3342] -> w2138
      tunnel: w2137 -> [w3341]
      tunnel: [w3341] -> w2136
      tunnel: w2135 -> [w3340]
      tunnel: [w3340] -> w2134
      tunnel: w2133 -> [w3339]
      tunnel: [w3339] -> w2132
      tunnel: w2131 -> [w3338]
      tunnel: [w3338] -> w2130
      tunnel: [w3327] -> w2011
      tunnel: w2010 -> [w3327]
      tunnel: [w3336] -> w1998
      tunnel: w1997 -> [w3336]
      tunnel: [w3335] -> w1977
      tunnel: w1976 -> [w3335]
      tunnel: w1833 -> [w3333]
      tunnel: [w3330] -> w1775
      tunnel: w1774 -> [w3330]
      tunnel: [w3329] -> w1748
      tunnel: w1747 -> [w3329]
      tunnel: [w3328] -> w1671
      tunnel: w1670 -> [w3328]
      tunnel: [w3326] -> w1641
      tunnel: [w3325] -> w1640
      tunnel: [w3321] -> w1637
      tunnel: w2156 -> [w3451]
      tunnel: w2154 -> [w3442]
      tunnel: w2152 -> [w3449]
      tunnel: [w3450] -> w1934
      tunnel: [w3449] -> w1932
      tunnel: [w3448] -> w1930
      tunnel: w2150 -> [w3448]
      tunnel: [w3447] -> w1928
      tunnel: w2148 -> [w3447]
      tunnel: [w3446] -> w1926
      tunnel: w2146 -> [w3446]
      tunnel: [w3445] -> w1924
      tunnel: [w3444] -> w1922
      tunnel: w2144 -> [w3444]
      tunnel: [w3443] -> w1920
      tunnel: w2142 -> [w3443]
      tunnel: [w3429] -> w1918
      tunnel: [w3441] -> w1917
      tunnel: w2140 -> [w3441]
      tunnel: [w3440] -> w1915
      tunnel: w2138 -> [w3440]
      tunnel: [w3439] -> w1913
      tunnel: w2136 -> [w3439]
      tunnel: w2134 -> [w3438]
      tunnel: [w3438] -> w1911
      tunnel: w2132 -> [w3437]
      tunnel: [w3437] -> w1909
      tunnel: w2130 -> [w3436]
      tunnel: [w3436] -> w1907
      tunnel: w2011 -> [w3435]
      tunnel: [w3434] -> w1905
      tunnel: w1998 -> [w3434]
      tunnel: [w3433] -> w1903
      tunnel: w1977 -> [w3433]
      tunnel: [w3432] -> w1899
      tunnel: [w3424] -> w1776
      tunnel: w1775 -> [w3424]
      tunnel: [w3423] -> w1749
      tunnel: w1748 -> [w3423]
      tunnel: [w3422] -> w1672
      tunnel: w1671 -> [w3422]
      tunnel: w1641 -> [w3419]
      tunnel: w1640 -> [w3418]
      tunnel: w1637 -> [w3417]
      tunnel: w1934 -> [w3454]
      tunnel: [w3454] -> w1933
      tunnel: w1932 -> [w3487]
      tunnel: [w3487] -> w1931
      tunnel: w1930 -> [w3486]
      tunnel: [w3486] -> w1929
      tunnel: w1928 -> [w3485]
      tunnel: [w3485] -> w1927
      tunnel: w1926 -> [w3484]
      tunnel: [w3484] -> w1925
      tunnel: w1924 -> [w3462]
      tunnel: [w3470] -> w1923
      tunnel: w1922 -> [w3483]
      tunnel: [w3483] -> w1921
      tunnel: w1920 -> [w3482]
      tunnel: [w3482] -> w1919
      tunnel: w1918 -> [w3465]
      tunnel: w1917 -> [w3481]
      tunnel: [w3481] -> w1916
      tunnel: w1915 -> [w3480]
      tunnel: [w3480] -> w1914
      tunnel: w1913 -> [w3479]
      tunnel: [w3479] -> w1912
      tunnel: w1911 -> [w3478]
      tunnel: [w3478] -> w1910
      tunnel: w1909 -> [w3477]
      tunnel: [w3477] -> w1908
      tunnel: w1907 -> [w3476]
      tunnel: [w3476] -> w1906
      tunnel: w1905 -> [w3475]
      tunnel: [w3475] -> w1904
      tunnel: w1903 -> [w3474]
      tunnel: [w3474] -> w1902
      tunnel: [w3469] -> w1900
      tunnel: w1899 -> [w3469]
      tunnel: [w3457] -> w1777
      tunnel: w1776 -> [w3457]
      tunnel: [w3456] -> w1750
      tunnel: w1749 -> [w3456]
      tunnel: [w3455] -> w1673
      tunnel: w1672 -> [w3455]
      tunnel: w1933 -> [w3521]
      tunnel: [w3521] -> w2222
      tunnel: w1931 -> [w3520]
      tunnel: [w3520] -> w2221
      tunnel: w1929 -> [w3519]
      tunnel: [w3519] -> w2220
      tunnel: w1927 -> [w3518]
      tunnel: [w3518] -> w2219
      tunnel: w1925 -> [w3516]
      tunnel: [w3515] -> w2218
      tunnel: w1923 -> [w3517]
      tunnel: w1921 -> [w3514]
      tunnel: [w3513] -> w2217
      tunnel: [w3511] -> w2216
      tunnel: w1919 -> [w3512]
      tunnel: [w3510] -> w2215
      tunnel: w1916 -> [w3510]
      tunnel: [w3509] -> w2214
      tunnel: w1914 -> [w3509]
      tunnel: w1912 -> [w3508]
      tunnel: [w3508] -> w2213
      tunnel: w1910 -> [w3507]
      tunnel: [w3507] -> w2212
      tunnel: [w3506] -> w2211
      tunnel: w1908 -> [w3506]
      tunnel: [w3505] -> w2210
      tunnel: w1906 -> [w3505]
      tunnel: [w3504] -> w1999
      tunnel: w1904 -> [w3504]
      tunnel: [w3503] -> w1978
      tunnel: w1902 -> [w3503]
      tunnel: [w3502] -> w1901
      tunnel: w1900 -> [w3501]
      tunnel: [w3500] -> w1838
      tunnel: [w3499] -> w1778
      tunnel: w1777 -> [w3499]
      tunnel: [w3498] -> w1751
      tunnel: w1750 -> [w3498]
      tunnel: [w3497] -> w1674
      tunnel: w1673 -> [w3497]
      tunnel: w2222 -> [w3619]
      tunnel: [w3619] -> w2129
      tunnel: w2221 -> [w3618]
      tunnel: [w3618] -> w2127
      tunnel: w2220 -> [w3617]
      tunnel: [w3617] -> w2125
      tunnel: w2219 -> [w3616]
      tunnel: [w3616] -> w2123
      tunnel: w2218 -> [w3594]
      tunnel: [w3594] -> w2121
      tunnel: w2217 -> [w3615]
      tunnel: [w3615] -> w2119
      tunnel: w2216 -> [w3614]
      tunnel: [w3614] -> w2117
      tunnel: w2215 -> [w3613]
      tunnel: [w3613] -> w2115
      tunnel: [w3612] -> w2113
      tunnel: w2214 -> [w3612]
      tunnel: [w3611] -> w2111
      tunnel: w2213 -> [w3611]
      tunnel: [w3610] -> w2109
      tunnel: w2212 -> [w3610]
      tunnel: w2211 -> [w3609]
      tunnel: [w3609] -> w2107
      tunnel: [w3608] -> w2105
      tunnel: w2210 -> [w3608]
      tunnel: [w3607] -> w2000
      tunnel: w1999 -> [w3607]
      tunnel: [w3606] -> w1979
      tunnel: w1978 -> [w3606]
      tunnel: w1901 -> [w3605]
      tunnel: w1838 -> [w3593]
      tunnel: [w3592] -> w1811
      tunnel: [w3591] -> w1779
      tunnel: w1778 -> [w3591]
      tunnel: [w3590] -> w1752
      tunnel: w1751 -> [w3590]
      tunnel: [w3589] -> w1675
      tunnel: w1674 -> [w3589]
      tunnel: w2129 -> [w3727]
      tunnel: [w3727] -> w2128
      tunnel: w2127 -> [w3726]
      tunnel: [w3726] -> w2126
      tunnel: w2125 -> [w3725]
      tunnel: [w3725] -> w2124
      tunnel: w2123 -> [w3724]
      tunnel: [w3724] -> w2122
      tunnel: w2121 -> [w3723]
      tunnel: [w3723] -> w2120
      tunnel: w2119 -> [w3722]
      tunnel: [w3722] -> w2118
      tunnel: w2117 -> [w3721]
      tunnel: [w3721] -> w2116
      tunnel: w2115 -> [w3720]
      tunnel: [w3720] -> w2114
      tunnel: w2113 -> [w3719]
      tunnel: [w3719] -> w2112
      tunnel: w2111 -> [w3718]
      tunnel: [w3718] -> w2110
      tunnel: w2109 -> [w3717]
      tunnel: [w3717] -> w2108
      tunnel: w2107 -> [w3716]
      tunnel: [w3716] -> w2106
      tunnel: w2105 -> [w3715]
      tunnel: [w3715] -> w2104
      tunnel: [w3704] -> w2001
      tunnel: w2000 -> [w3704]
      tunnel: [w3712] -> w1980
      tunnel: w1979 -> [w3712]
      tunnel: w1811 -> [w3709]
      tunnel: [w3708] -> w1810
      tunnel: [w3707] -> w1780
      tunnel: w1779 -> [w3707]
      tunnel: [w3706] -> w1753
      tunnel: w1752 -> [w3706]
      tunnel: [w3705] -> w1676
      tunnel: w1675 -> [w3705]
      tunnel: [w3700] -> w1638
      tunnel: w2128 -> [w3826]
      tunnel: [w3825] -> w1898
      tunnel: w2126 -> [w3823]
      tunnel: w2124 -> [w3818]
      tunnel: [w3824] -> w1896
      tunnel: w2122 -> [w3824]
      tunnel: [w3823] -> w1894
      tunnel: [w3822] -> w1892
      tunnel: w2120 -> [w3822]
      tunnel: [w3821] -> w1890
      tunnel: [w3820] -> w1888
      tunnel: w2118 -> [w3820]
      tunnel: [w3819] -> w1886
      tunnel: w2116 -> [w3819]
      tunnel: [w3804] -> w1884
      tunnel: w2114 -> [w3817]
      tunnel: [w3817] -> w1883
      tunnel: [w3816] -> w1881
      tunnel: w2112 -> [w3816]
      tunnel: w2110 -> [w3815]
      tunnel: [w3815] -> w1879
      tunnel: w2108 -> [w3814]
      tunnel: [w3814] -> w1877
      tunnel: w2106 -> [w3813]
      tunnel: [w3813] -> w1875
      tunnel: w2104 -> [w3812]
      tunnel: [w3812] -> w1873
      tunnel: w2001 -> [w3811]
      tunnel: [w3808] -> w1871
      tunnel: w1980 -> [w3808]
      tunnel: [w3807] -> w1867
      tunnel: w1810 -> [w3799]
      tunnel: [w3798] -> w1781
      tunnel: w1780 -> [w3798]
      tunnel: [w3797] -> w1754
      tunnel: w1753 -> [w3797]
      tunnel: [w3796] -> w1677
      tunnel: w1676 -> [w3796]
      tunnel: w1638 -> [w3793]
      tunnel: w1898 -> [w3829]
      tunnel: [w3829] -> w1897
      tunnel: w1896 -> [w3858]
      tunnel: [w3858] -> w1895
      tunnel: w1894 -> [w3857]
      tunnel: [w3857] -> w1893
      tunnel: w1892 -> [w3856]
      tunnel: [w3856] -> w1891
      tunnel: w1890 -> [w3838]
      tunnel: [w3844] -> w1889
      tunnel: w1888 -> [w3855]
      tunnel: [w3855] -> w1887
      tunnel: w1886 -> [w3854]
      tunnel: [w3854] -> w1885
      tunnel: w1884 -> [w3830]
      tunnel: w1883 -> [w3853]
      tunnel: [w3853] -> w1882
      tunnel: w1881 -> [w3852]
      tunnel: [w3852] -> w1880
      tunnel: w1879 -> [w3851]
      tunnel: [w3851] -> w1878
      tunnel: w1877 -> [w3850]
      tunnel: [w3850] -> w1876
      tunnel: w1875 -> [w3849]
      tunnel: [w3849] -> w1874
      tunnel: w1873 -> [w3848]
      tunnel: [w3848] -> w1872
      tunnel: w1871 -> [w3847]
      tunnel: [w3847] -> w1870
      tunnel: [w3843] -> w1868
      tunnel: w1867 -> [w3843]
      tunnel: [w3833] -> w1782
      tunnel: w1781 -> [w3833]
      tunnel: [w3832] -> w1755
      tunnel: w1754 -> [w3832]
      tunnel: [w3831] -> w1678
      tunnel: w1677 -> [w3831]
      tunnel: w1897 -> [w3890]
      tunnel: [w3890] -> w2209
      tunnel: w1895 -> [w3889]
      tunnel: [w3889] -> w2208
      tunnel: w1893 -> [w3888]
      tunnel: [w3888] -> w2207
      tunnel: w1891 -> [w3886]
      tunnel: [w3885] -> w2206
      tunnel: w1889 -> [w3887]
      tunnel: w1887 -> [w3884]
      tunnel: [w3883] -> w2205
      tunnel: [w3881] -> w2204
      tunnel: w1885 -> [w3882]
      tunnel: w1882 -> [w3880]
      tunnel: [w3880] -> w2203
      tunnel: [w3879] -> w2202
      tunnel: w1880 -> [w3879]
      tunnel: [w3878] -> w2201
      tunnel: w1878 -> [w3878]
      tunnel: [w3877] -> w2200
      tunnel: w1876 -> [w3877]
      tunnel: w1874 -> [w3876]
      tunnel: [w3876] -> w2199
      tunnel: [w3875] -> w2198
      tunnel: w1872 -> [w3875]
      tunnel: [w3874] -> w1981
      tunnel: w1870 -> [w3874]
      tunnel: [w3873] -> w1869
      tunnel: w1868 -> [w3872]
      tunnel: [w3871] -> w1837
      tunnel: [w3870] -> w1783
      tunnel: w1782 -> [w3870]
      tunnel: [w3869] -> w1756
      tunnel: w1755 -> [w3869]
      tunnel: [w3868] -> w1679
      tunnel: w1678 -> [w3868]
      tunnel: w2209 -> [w3987]
      tunnel: [w3987] -> w2103
      tunnel: w2208 -> [w3986]
      tunnel: [w3986] -> w2101
      tunnel: w2207 -> [w3985]
      tunnel: [w3985] -> w2099
      tunnel: w2206 -> [w3964]
      tunnel: [w3964] -> w2097
      tunnel: w2205 -> [w3984]
      tunnel: [w3984] -> w2095
      tunnel: w2204 -> [w3983]
      tunnel: [w3983] -> w2093
      tunnel: w2203 -> [w3982]
      tunnel: [w3982] -> w2091
      tunnel: [w3981] -> w2089
      tunnel: w2202 -> [w3981]
      tunnel: [w3980] -> w2087
      tunnel: w2201 -> [w3980]
      tunnel: [w3979] -> w2085
      tunnel: w2200 -> [w3979]
      tunnel: [w3978] -> w2083
      tunnel: w2199 -> [w3978]
      tunnel: w2198 -> [w3977]
      tunnel: [w3977] -> w2081
      tunnel: [w3976] -> w1982
      tunnel: w1981 -> [w3976]
      tunnel: w1869 -> [w3975]
      tunnel: w1837 -> [w3963]
      tunnel: [w3962] -> w1832
      tunnel: [w3960] -> w1784
      tunnel: w1783 -> [w3960]
      tunnel: [w3959] -> w1757
      tunnel: w1756 -> [w3959]
      tunnel: [w3958] -> w1680
      tunnel: w1679 -> [w3958]
      tunnel: w2103 -> [w4090]
      tunnel: [w4090] -> w2102
      tunnel: w2101 -> [w4089]
      tunnel: [w4089] -> w2100
      tunnel: w2099 -> [w4088]
      tunnel: [w4088] -> w2098
      tunnel: w2097 -> [w4087]
      tunnel: [w4087] -> w2096
      tunnel: w2095 -> [w4086]
      tunnel: [w4086] -> w2094
      tunnel: w2093 -> [w4085]
      tunnel: [w4085] -> w2092
      tunnel: w2091 -> [w4084]
      tunnel: [w4084] -> w2090
      tunnel: w2089 -> [w4083]
      tunnel: [w4083] -> w2088
      tunnel: w2087 -> [w4082]
      tunnel: [w4082] -> w2086
      tunnel: w2085 -> [w4081]
      tunnel: [w4081] -> w2084
      tunnel: w2083 -> [w4080]
      tunnel: [w4080] -> w2082
      tunnel: w2081 -> [w4079]
      tunnel: [w4079] -> w2080
      tunnel: [w4068] -> w1983
      tunnel: w1982 -> [w4068]
      tunnel: w1832 -> [w4075]
      tunnel: [w4073] -> w1785
      tunnel: w1784 -> [w4073]
      tunnel: [w4072] -> w1758
      tunnel: w1757 -> [w4072]
      tunnel: [w4071] -> w1681
      tunnel: w1680 -> [w4071]
      tunnel: [w4070] -> w1662
      tunnel: [w4069] -> w1661
      tunnel: w2102 -> [w4189]
      tunnel: w2100 -> [w4183]
      tunnel: w2098 -> [w4164]
      tunnel: w2096 -> [w4187]
      tunnel: [w4188] -> w1866
      tunnel: [w4187] -> w1864
      tunnel: [w4186] -> w1862
      tunnel: [w4185] -> w1861
      tunnel: w2094 -> [w4185]
      tunnel: [w4184] -> w1859
      tunnel: w2092 -> [w4184]
      tunnel: [w4171] -> w1857
      tunnel: [w4182] -> w1856
      tunnel: w2090 -> [w4182]
      tunnel: w2088 -> [w4181]
      tunnel: [w4181] -> w1854
      tunnel: w2086 -> [w4180]
      tunnel: [w4180] -> w1852
      tunnel: w2084 -> [w4179]
      tunnel: [w4179] -> w1850
      tunnel: w2082 -> [w4178]
      tunnel: [w4178] -> w1848
      tunnel: [w4177] -> w1846
      tunnel: w2080 -> [w4177]
      tunnel: w1983 -> [w4176]
      tunnel: [w4173] -> w1841
      tunnel: [w4166] -> w1786
      tunnel: w1785 -> [w4166]
      tunnel: [w4165] -> w1759
      tunnel: w1758 -> [w4165]
      tunnel: [w4164] -> w1736
      tunnel: [w4163] -> w1682
      tunnel: w1681 -> [w4163]
      tunnel: w1662 -> [w4162]
      tunnel: w1661 -> [w4161]
      tunnel: w1866 -> [w4192]
      tunnel: [w4192] -> w1865
      tunnel: w1864 -> [w4219]
      tunnel: [w4219] -> w1863
      tunnel: w1862 -> [w4202]
      tunnel: w1861 -> [w4218]
      tunnel: [w4218] -> w1860
      tunnel: w1859 -> [w4217]
      tunnel: [w4217] -> w1858
      tunnel: w1857 -> [w4193]
      tunnel: w1856 -> [w4216]
      tunnel: [w4216] -> w1855
      tunnel: w1854 -> [w4215]
      tunnel: [w4215] -> w1853
      tunnel: w1852 -> [w4214]
      tunnel: [w4214] -> w1851
      tunnel: w1850 -> [w4213]
      tunnel: [w4213] -> w1849
      tunnel: w1848 -> [w4212]
      tunnel: [w4212] -> w1847
      tunnel: w1846 -> [w4211]
      tunnel: [w4211] -> w1845
      tunnel: [w4208] -> w1844
      tunnel: [w4207] -> w1842
      tunnel: w1841 -> [w4207]
      tunnel: [w4197] -> w1787
      tunnel: w1786 -> [w4197]
      tunnel: [w4196] -> w1760
      tunnel: w1759 -> [w4196]
      tunnel: w1736 -> [w4195]
      tunnel: [w4195] -> w1732
      tunnel: [w4194] -> w1683
      tunnel: w1682 -> [w4194]
      tunnel: w1865 -> [w4249]
      tunnel: w1863 -> [w4247]
      tunnel: w1860 -> [w4245]
      tunnel: w1858 -> [w4243]
      tunnel: [w4249] -> w2197
      tunnel: [w4246] -> w2196
      tunnel: [w4244] -> w2195
      tunnel: [w4242] -> w2194
      tunnel: w1855 -> [w4241]
      tunnel: [w4241] -> w2193
      tunnel: [w4240] -> w2192
      tunnel: w1853 -> [w4240]
      tunnel: [w4239] -> w2191
      tunnel: w1851 -> [w4239]
      tunnel: [w4238] -> w2190
      tunnel: w1849 -> [w4238]
      tunnel: [w4237] -> w2189
      tunnel: w1847 -> [w4237]
      tunnel: w1845 -> [w4236]
      tunnel: [w4236] -> w2188
      tunnel: w1844 -> [w4248]
      tunnel: [w4235] -> w1843
      tunnel: w1842 -> [w4234]
      tunnel: [w4233] -> w1836
      tunnel: [w4232] -> w1788
      tunnel: w1787 -> [w4232]
      tunnel: [w4231] -> w1761
      tunnel: w1760 -> [w4231]
      tunnel: [w4230] -> w1733
      tunnel: w1732 -> [w4230]
      tunnel: [w4229] -> w1684
      tunnel: w1683 -> [w4229]
      tunnel: w2197 -> [w4344]
      tunnel: w2196 -> [w4325]
      tunnel: w2195 -> [w4343]
      tunnel: w2194 -> [w4342]
      tunnel: w2193 -> [w4317]
      tunnel: w2192 -> [w4341]
      tunnel: w2191 -> [w4340]
      tunnel: w2190 -> [w4339]
      tunnel: w2189 -> [w4338]
      tunnel: w2188 -> [w4337]
      tunnel: [w4344] -> w2079
      tunnel: [w4325] -> w2078
      tunnel: [w4343] -> w2077
      tunnel: [w4342] -> w2076
      tunnel: [w4341] -> w2075
      tunnel: [w4340] -> w2074
      tunnel: [w4339] -> w2073
      tunnel: [w4338] -> w2072
      tunnel: [w4337] -> w2071
      tunnel: w1843 -> [w4336]
      tunnel: w1836 -> [w4324]
      tunnel: [w4323] -> w1831
      tunnel: [w4321] -> w1789
      tunnel: w1788 -> [w4321]
      tunnel: [w4320] -> w1762
      tunnel: w1761 -> [w4320]
      tunnel: [w4319] -> w1734
      tunnel: w1733 -> [w4319]
      tunnel: [w4318] -> w1685
      tunnel: w1684 -> [w4318]
      tunnel: [w4317] -> w1650
      tunnel: w2079 -> [w4445]
      tunnel: [w4445] -> w1801
      tunnel: w2078 -> [w4444]
      tunnel: [w4444] -> w1802
      tunnel: w2077 -> [w4443]
      tunnel: [w4443] -> w1803
      tunnel: w2076 -> [w4442]
      tunnel: [w4442] -> w1804
      tunnel: w2075 -> [w4441]
      tunnel: [w4441] -> w1805
      tunnel: w2074 -> [w4440]
      tunnel: [w4440] -> w1806
      tunnel: w2073 -> [w4439]
      tunnel: [w4439] -> w1807
      tunnel: w2072 -> [w4438]
      tunnel: [w4438] -> w1808
      tunnel: w2071 -> [w4437]
      tunnel: [w4437] -> w1809
      tunnel: w1831 -> [w4433]
      tunnel: [w4425] -> w1790
      tunnel: w1789 -> [w4425]
      tunnel: [w4431] -> w1763
      tunnel: w1762 -> [w4431]
      tunnel: [w4430] -> w1735
      tunnel: w1734 -> [w4430]
      tunnel: [w4429] -> w1686
      tunnel: w1685 -> [w4429]
      tunnel: [w4428] -> w1660
      tunnel: [w4426] -> w1659
      tunnel: w1650 -> [w4427]
      tunnel: [w4427] -> w1646
      tunnel: w1809 -> [w4542]
      tunnel: [w4542] -> w1800
      tunnel: w1808 -> [w4541]
      tunnel: [w4541] -> w1799
      tunnel: w1807 -> [w4540]
      tunnel: [w4540] -> w1798
      tunnel: w1806 -> [w4539]
      tunnel: [w4539] -> w1797
      tunnel: w1805 -> [w4538]
      tunnel: [w4538] -> w1796
      tunnel: w1804 -> [w4537]
      tunnel: [w4537] -> w1795
      tunnel: w1803 -> [w4536]
      tunnel: [w4536] -> w1794
      tunnel: w1802 -> [w4535]
      tunnel: [w4535] -> w1793
      tunnel: w1801 -> [w4519]
      tunnel: w1790 -> [w4529]
      tunnel: w1763 -> [w4528]
      tunnel: w1735 -> [w4527]
      tunnel: [w4526] -> w1731
      tunnel: [w4525] -> w1730
      tunnel: [w4524] -> w1721
      tunnel: [w4523] -> w1718
      tunnel: [w4522] -> w1687
      tunnel: w1686 -> [w4522]
      tunnel: w1660 -> [w4521]
      tunnel: w1659 -> [w4520]
      tunnel: [w4518] -> w1647
      tunnel: w1646 -> [w4518]
      tunnel: w1800 -> [w4569]
      tunnel: [w4569] -> w1729
      tunnel: w1799 -> [w4568]
      tunnel: [w4568] -> w1728
      tunnel: w1798 -> [w4567]
      tunnel: [w4567] -> w1727
      tunnel: w1797 -> [w4566]
      tunnel: [w4566] -> w1726
      tunnel: w1796 -> [w4565]
      tunnel: [w4565] -> w1725
      tunnel: w1795 -> [w4564]
      tunnel: [w4564] -> w1724
      tunnel: w1794 -> [w4563]
      tunnel: [w4563] -> w1723
      tunnel: w1793 -> [w4562]
      tunnel: [w4562] -> w1722
      tunnel: w1731 -> [w4550]
      tunnel: w1730 -> [w4549]
      tunnel: w1721 -> [w4548]
      tunnel: [w4547] -> w1720
      tunnel: [w4546] -> w1719
      tunnel: w1718 -> [w4546]
      tunnel: [w4545] -> w1688
      tunnel: w1687 -> [w4545]
      tunnel: [w4544] -> w1658
      tunnel: [w4543] -> w1648
      tunnel: w1647 -> [w4543]
      tunnel: w1729 -> [w4598]
      tunnel: [w4598] -> w1717
      tunnel: w1728 -> [w4597]
      tunnel: [w4597] -> w1715
      tunnel: w1727 -> [w4596]
      tunnel: [w4596] -> w1713
      tunnel: w1726 -> [w4595]
      tunnel: [w4595] -> w1711
      tunnel: w1725 -> [w4594]
      tunnel: [w4594] -> w1709
      tunnel: w1724 -> [w4593]
      tunnel: [w4592] -> w1707
      tunnel: w1723 -> [w4588]
      tunnel: [w4587] -> w1705
      tunnel: w1722 -> [w4591]
      tunnel: [w4590] -> w1703
      tunnel: w1720 -> [w4589]
      tunnel: w1719 -> [w4586]
      tunnel: [w4585] -> w1689
      tunnel: w1688 -> [w4585]
      tunnel: w1658 -> [w4584]
      tunnel: [w4584] -> w1657
      tunnel: [w4583] -> w1652
      tunnel: [w4582] -> w1651
      tunnel: [w4581] -> w1649
      tunnel: w1648 -> [w4581]
      tunnel: w1717 -> [w4689]
      tunnel: [w4689] -> w1716
      tunnel: w1715 -> [w4688]
      tunnel: [w4688] -> w1714
      tunnel: w1713 -> [w4687]
      tunnel: [w4687] -> w1712
      tunnel: w1711 -> [w4686]
      tunnel: [w4686] -> w1710
      tunnel: w1709 -> [w4685]
      tunnel: [w4685] -> w1708
      tunnel: w1707 -> [w4684]
      tunnel: [w4684] -> w1706
      tunnel: w1705 -> [w4683]
      tunnel: [w4683] -> w1704
      tunnel: w1703 -> [w4669]
      tunnel: [w4669] -> w1702
      tunnel: [w4681] -> w1701
      tunnel: [w4682] -> w1690
      tunnel: w1689 -> [w4682]
      tunnel: w1657 -> [w4681]
      tunnel: w1652 -> [w4668]
      tunnel: w1651 -> [w4667]
      tunnel: w1649 -> [w4666]
      tunnel: [w4896] -> w2273
      tunnel: [w4897] -> w2275
      tunnel: [w4898] -> w2276
      tunnel: [w4899] -> w2277
      tunnel: [w4900] -> w2281
      tunnel: [w4770] -> w2283
      tunnel: [w4771] -> w2285
      tunnel: [w4901] -> w2287
      tunnel: [w4902] -> w2295
      tunnel: w1716 -> [w4896]
      tunnel: w1714 -> [w4897]
      tunnel: w1712 -> [w4898]
      tunnel: w1710 -> [w4899]
      tunnel: w1708 -> [w4900]
      tunnel: w1706 -> [w4770]
      tunnel: w1704 -> [w4771]
      tunnel: w1702 -> [w4901]
      tunnel: w1701 -> [w4902]
      tunnel: [w4817] -> w1664
      tunnel: w1690 -> [w4817]
      frame #0 {
        n766 = Index Array(array=w2325, index #1=0 ("index")) -> (element #1=w2327:T3, element #2=w2328:T3)  [unwired: 1 in]
        n767 = Index Array(array=w2337, index #1=0 ("index")) -> (element #1=w2360:T4, element #2=w2361:T4)  [unwired: 1 in]
        n768 = Index Array(array=w2339, index #1=0 ("index")) -> (element #1=w2383:T6, element #2=w2382:T6)  [unwired: 1 in]
        n769 = Index Array(array=w2338, index #1=0 ("index")) -> (element #1=w2348:T5, element #2=w2349:T5)  [unwired: 1 in]
        n770 = Index Array(array=w2386, index #1=0 ("index")) -> (element #1=w2400:T7, element #2=w2399:T7)  [unwired: 1 in]
        n771 = Index Array(array=w2298, index #1=0 ("index")) -> (element #1=w2312:T2, element #2=w2311:T2)  [unwired: 1 in]
        n772 = Unbundle By Name(w2327) -> ("disc 05"=w2329:bool, "auto/man 05"=w2330:bool, "projector 05"=w2331:bool, "cam 05"=w2332:bool)
        n773 = Unbundle By Name(w2328) -> ("cam 05"=w2333:bool, "projector 05"=w2334:bool, "auto/man 05"=w2335:bool, "disc 05"=w2336:bool)
        n774 = Unbundle By Name(w2360) -> ("disc 04"=w2362:bool, "auto/man 04"=w2363:bool, "projector 04"=w2364:bool, "cam 04"=w2365:bool)
        n775 = Unbundle By Name(w2361) -> ("cam 04"=w2366:bool, "projector 04"=w2367:bool, "auto/man 04"=w2368:bool, "disc 04"=w2369:bool)
        n776 = Unbundle By Name(w2348) -> ("disc 03"=w2350:bool, "auto/man 03"=w2352:bool, "projector 03"=w2354:bool, "cam 03"=w2356:bool)
        n777 = Unbundle By Name(w2349) -> ("cam 03"=w2357:bool, "projector 03"=w2355:bool, "auto/man 03"=w2353:bool, "disc 03"=w2351:bool)
        n778 = Unbundle By Name(w2383) -> ("disc 02"=w2381:bool, "auto/man 02"=w2380:bool, "projector 02"=w2379:bool, "cam 02"=w2378:bool)
        n779 = Unbundle By Name(w2382) -> ("cam 02"=w2377:bool, "projector 02"=w2376:bool, "auto/man 02"=w2375:bool, "disc 02"=w2374:bool)
        n780 = Unbundle By Name(w2400) -> ("disc 01"=w2398:bool, "auto/man 01"=w2396:bool, "projector 01"=w2394:bool, "cam 01"=w2392:bool)
        n781 = Unbundle By Name(w2399) -> ("cam 01"=w2391:bool, "projector 01"=w2393:bool, "auto/man 01"=w2395:bool, "disc 01"=w2397:bool)
        n782 = Unbundle By Name(w2312) -> ("disc 06"=w2310:bool, "auto/man 06"=w2309:bool, "projector 06"=w2308:bool, "cam 06"=w2307:bool)
        n783 = Unbundle By Name(w2311) -> ("cam 06"=w2306:bool, "projector 06"=w2305:bool, "auto/man 06"=w2304:bool, "disc 06"=w2303:bool)
        n784 = Not Equal?(x=w2356, y=w2357) -> (x != y?=w2347:bool)
        n785 = Not Equal?(x=w2392, y=w2391) -> (x != y?=w2387:bool)
        n786 = Not Equal?(x=w2332, y=w2333) -> (x != y?=w2324:bool)
        n787 = Not Equal?(x=w2365, y=w2366) -> (x != y?=w2343:bool)
        n788 = Not Equal?(x=w2378, y=w2377) -> (x != y?=w2370:bool)
        n789 = Not Equal?(x=w2307, y=w2306) -> (x != y?=w2302:bool)
        n790 = Not Equal?(x=w2354, y=w2355) -> (x != y?=w2346:bool)
        n791 = Not Equal?(x=w2394, y=w2393) -> (x != y?=w2388:bool)
        n792 = Not Equal?(x=w2331, y=w2334) -> (x != y?=w2323:bool)
        n793 = Not Equal?(x=w2364, y=w2367) -> (x != y?=w2342:bool)
        n794 = Not Equal?(x=w2379, y=w2376) -> (x != y?=w2371:bool)
        n795 = Not Equal?(x=w2308, y=w2305) -> (x != y?=w2301:bool)
        n796 = Not Equal?(x=w2352, y=w2353) -> (x != y?=w2345:bool)
        n797 = Not Equal?(x=w2396, y=w2395) -> (x != y?=w2389:bool)
        n798 = Not Equal?(x=w2330, y=w2335) -> (x != y?=w2322:bool)
        n799 = Not Equal?(x=w2363, y=w2368) -> (x != y?=w2341:bool)
        n800 = Not Equal?(x=w2380, y=w2375) -> (x != y?=w2372:bool)
        n801 = Not Equal?(x=w2309, y=w2304) -> (x != y?=w2300:bool)
        n802 = Not Equal?(x=w2350, y=w2351) -> (x != y?=w2344:bool)
        n803 = Not Equal?(x=w2398, y=w2397) -> (x != y?=w2390:bool)
        n804 = Not Equal?(x=w2329, y=w2336) -> (x != y?=w2321:bool)
        n805 = Not Equal?(x=w2362, y=w2369) -> (x != y?=w2340:bool)
        n806 = Not Equal?(x=w2381, y=w2374) -> (x != y?=w2373:bool)
        n807 = Not Equal?(x=w2310, y=w2303) -> (x != y?=w2299:bool)
      }
      frame #1 {
        n808 = Build Array(w2468, w2467, w2466, w2465) -> (w2434:bool[])
        n809 = Build Array(w2453, w2456, w2455, w2454) -> (w2438:bool[])
        n810 = Build Array(w2462, w2464, w2463, w2461) -> (w2444:bool[])
        n811 = Build Array(w2452, w2449, w2450, w2451) -> (w2447:bool[])
        n812 = Build Array(w2460, w2458, w2457, w2459) -> (w2445:bool[])
        n813 = Build Array(w2424, w2423, w2422, w2421) -> (w2427:bool[])
        n814 = Or Array Elements(Boolean array=w2444) -> (logical OR=w2441:bool)
        n815 = Boolean Array To Number(Boolean array=w2444) -> (number=w2440:u32)
        n816 = Or Array Elements(Boolean array=w2434) -> (logical OR=w2435:bool)
        n817 = Or Array Elements(Boolean array=w2438) -> (logical OR=w2439:bool)
        n818 = Boolean Array To Number(Boolean array=w2434) -> (number=w2436:u32)
        n819 = Boolean Array To Number(Boolean array=w2438) -> (number=w2437:u32)
        n820 = Or Array Elements(Boolean array=w2445) -> (logical OR=w2443:bool)
        n821 = Boolean Array To Number(Boolean array=w2445) -> (number=w2442:u32)
        n822 = Or Array Elements(Boolean array=w2447) -> (logical OR=w2448:bool)
        n823 = Boolean Array To Number(Boolean array=w2447) -> (number=w2446:u32)
        n824 = Or Array Elements(Boolean array=w2427) -> (logical OR=w2426:bool)
        n825 = Boolean Array To Number(Boolean array=w2427) -> (number=w2425:u32)
        n826 = case shown="True" w2435 {
          tunnel: w2436 -> [_ w2496]
          frame False {
          }
          frame True {
            n827 = property on="DISC 05" class="Bool (strict)"() -> ("Value"=w2493:bool)  [unwired: 2 in, 2 out]
            n828 = property on="projector 05" class="Bool (strict)"() -> ("Value"=w2494:bool)  [unwired: 2 in, 2 out]
            n829 = property on="AUTO/MAN 05" class="Bool (strict)"() -> ("Value"=w2492:bool)  [unwired: 2 in, 2 out]
            n830 = property on="cam 05" class="Bool (strict)"() -> ("Value"=w2495:bool)  [unwired: 2 in, 2 out]
            n831 = call "save log.vi"("camera"=w2495, "auto/man"=w2492, "projector"=w2494, "disc"=w2493, "Case Num"=w2496, "Disc Number"="Disc 05") -> ("Error out"=w2491:errorcluster)  [unwired: 5 in]
            n832 = shared-variable ".\\Maintenance.lvlib\\error_16"(w2491) -> ()  [unwired: 1 in, 1 out]
          }
        }
        n833 = case shown="True" w2439 {
          tunnel: w2437 -> [_ w2503]
          frame False {
          }
          frame True {
            n834 = property on="DISC 04" class="Bool (strict)"() -> ("Value"=w2500:bool)  [unwired: 2 in, 2 out]
            n835 = property on="projector 04" class="Bool (strict)"() -> ("Value"=w2501:bool)  [unwired: 2 in, 2 out]
            n836 = property on="AUTO/MAN 04" class="Bool (strict)"() -> ("Value"=w2499:bool)  [unwired: 2 in, 2 out]
            n837 = property on="cam 04" class="Bool (strict)"() -> ("Value"=w2502:bool)  [unwired: 2 in, 2 out]
            n838 = call "save log.vi"("camera"=w2502, "auto/man"=w2499, "projector"=w2501, "disc"=w2500, "Case Num"=w2503, "Disc Number"="Disc 04") -> ("Error out"=w2498:errorcluster)  [unwired: 5 in]
            n839 = shared-variable ".\\Maintenance.lvlib\\error_15"(w2498) -> ()  [unwired: 1 in, 1 out]
          }
        }
        n840 = case shown="True" w2441 {
          tunnel: w2440 -> [_ w2510]
          frame False {
          }
          frame True {
            n841 = property on="DISC 03" class="Bool (strict)"() -> ("Value"=w2507:bool)  [unwired: 2 in, 2 out]
            n842 = property on="projector 03" class="Bool (strict)"() -> ("Value"=w2508:bool)  [unwired: 2 in, 2 out]
            n843 = property on="AUTO/MAN 03" class="Bool (strict)"() -> ("Value"=w2506:bool)  [unwired: 2 in, 2 out]
            n844 = property on="cam 03" class="Bool (strict)"() -> ("Value"=w2509:bool)  [unwired: 2 in, 2 out]
            n845 = call "save log.vi"("camera"=w2509, "auto/man"=w2506, "projector"=w2508, "disc"=w2507, "Case Num"=w2510, "Disc Number"="Disc 03") -> ("Error out"=w2505:errorcluster)  [unwired: 5 in]
            n846 = shared-variable ".\\Maintenance.lvlib\\error_14"(w2505) -> ()  [unwired: 1 in, 1 out]
          }
        }
        n847 = case shown="True" w2443 {
          tunnel: w2442 -> [_ w2517]
          frame False {
          }
          frame True {
            n848 = property on="DISC 02" class="Bool (strict)"() -> ("Value"=w2514:bool)  [unwired: 2 in, 2 out]
            n849 = property on="projector 02" class="Bool (strict)"() -> ("Value"=w2515:bool)  [unwired: 2 in, 2 out]
            n850 = property on="AUTO/MAN 02" class="Bool (strict)"() -> ("Value"=w2513:bool)  [unwired: 2 in, 2 out]
            n851 = property on="cam 02" class="Bool (strict)"() -> ("Value"=w2516:bool)  [unwired: 2 in, 2 out]
            n852 = call "save log.vi"("camera"=w2516, "auto/man"=w2513, "projector"=w2515, "disc"=w2514, "Case Num"=w2517, "Disc Number"="Disc 02") -> ("Error out"=w2512:errorcluster)  [unwired: 5 in]
            n853 = shared-variable ".\\Maintenance.lvlib\\error_13"(w2512) -> ()  [unwired: 1 in, 1 out]
          }
        }
        n854 = case shown="True" w2448 {
          tunnel: w2446 -> [_ w2524]
          frame False {
          }
          frame True {
            n855 = property on="DISC 01" class="Bool (strict)"() -> ("Value"=w2521:bool)  [unwired: 2 in, 2 out]
            n856 = property on="projector 01" class="Bool (strict)"() -> ("Value"=w2522:bool)  [unwired: 2 in, 2 out]
            n857 = property on="AUTO/MAN 01" class="Bool (strict)"() -> ("Value"=w2520:bool)  [unwired: 2 in, 2 out]
            n858 = property on="cam 01" class="Bool (strict)"() -> ("Value"=w2523:bool)  [unwired: 2 in, 2 out]
            n859 = call "save log.vi"("camera"=w2523, "auto/man"=w2520, "projector"=w2522, "disc"=w2521, "Case Num"=w2524, "Disc Number"="Disc 01") -> ("Error out"=w2519:errorcluster)  [unwired: 5 in]
            n860 = shared-variable ".\\Maintenance.lvlib\\error_12"(w2519) -> ()  [unwired: 1 in, 1 out]
          }
        }
        n861 = shared-variable ".\\Setting Lib.lvlib\\processing file path"() -> (w2414:path)  [unwired: 1 in, 1 out]
        n862 = case shown="True" w2426 {
          tunnel: w2425 -> [_ w2489]
          frame False {
          }
          frame True {
            n863 = property on="DISC 06" class="Bool (strict)"() -> ("Value"=w2486:bool)  [unwired: 2 in, 2 out]
            n864 = property on="projector 06" class="Bool (strict)"() -> ("Value"=w2487:bool)  [unwired: 2 in, 2 out]
            n865 = property on="AUTO/MAN 06" class="Bool (strict)"() -> ("Value"=w2485:bool)  [unwired: 2 in, 2 out]
            n866 = property on="cam 06" class="Bool (strict)"() -> ("Value"=w2488:bool)  [unwired: 2 in, 2 out]
            n867 = call "save log.vi"("camera"=w2488, "auto/man"=w2485, "projector"=w2487, "disc"=w2486, "Case Num"=w2489, "Disc Number"="Disc 06") -> ("Error out"=w2484:errorcluster)  [unwired: 5 in]
            n868 = shared-variable ".\\Maintenance.lvlib\\error_16"(w2484) -> ()  [unwired: 1 in, 1 out]
          }
        }
        n869 = shared-variable ".\\D01.lvlib\\LiveViewD01"() -> (w2411:refnum<image>, error out=w2419:errorcluster)  [unwired: 1 in]
        n870 = shared-variable ".\\D01.lvlib\\GradingThrD01"() -> (w2416:dbl[])  [unwired: 1 in, 1 out]
        n871 = Wait (ms)(milliseconds to wait=u32 5) -> ()  [unwired: 1 out]
        n872 = call "IMAQ Copy"("error in (no error)"=w2419, "Image Dst"=w2413, "Image Src"=w2411) -> ("error out"=w2418:errorcluster, "Image Dst Out"=w2412:T9)  [unwired: 3 in]
      }
      frame #2 {
        n873 = shared-variable ".\\control setting.lvlib\\bias"() -> (w2527:dbl[])  [unwired: 1 in, 1 out]
        n874 = shared-variable ".\\Maintenance.lvlib\\error_104"() -> (w2550:errorcluster)  [unwired: 1 in, 1 out]
        n875 = shared-variable ".\\Maintenance.lvlib\\error_104"() -> (w2578:errorcluster)  [unwired: 1 in, 1 out]
        n876 = shared-variable ".\\Maintenance.lvlib\\error_84"() -> (w2590:errorcluster)  [unwired: 1 in, 1 out]
        n877 = shared-variable ".\\Maintenance.lvlib\\error_94"() -> (w2584:errorcluster)  [unwired: 1 in, 1 out]
        n878 = shared-variable ".\\Maintenance.lvlib\\error_89"() -> (w2587:errorcluster)  [unwired: 1 in, 1 out]
        n879 = shared-variable ".\\Maintenance.lvlib\\error_99"() -> (w2581:errorcluster)  [unwired: 1 in, 1 out]
        n880 = property on="AUTO/MAN 06" class="Bool (strict)"() -> ("Value"=w2552:bool)  [unwired: 2 in, 2 out]
        n881 = property on="AUTO/MAN 05" class="Bool (strict)"() -> ("Value"=w2565:bool)  [unwired: 2 in, 2 out]
        n882 = Index Array(array=w2527, index=0) -> (element=w2529:dbl)
        n883 = property on="DISC 03" class="Bool (strict)"() -> ("Value"=w2574:bool)  [unwired: 2 in, 2 out]
        n884 = property on="AUTO/MAN 03" class="Bool (strict)"() -> ("Value"=w2563:bool)  [unwired: 2 in, 2 out]
        n885 = property on="AUTO/MAN 04" class="Bool (strict)"() -> ("Value"=w2564:bool)  [unwired: 2 in, 2 out]
        n886 = shared-variable ".\\D06.lvlib\\projector 06"() -> (w2541:bool)  [unwired: 1 in, 1 out]
        "projector 06" <- w2541
        n887 = property on="AUTO/MAN 02" class="Bool (strict)"() -> ("Value"=w2562:bool)  [unwired: 2 in, 2 out]
        n888 = property on="DISC 01" class="Bool (strict)"() -> ("Value"=w2572:bool)  [unwired: 2 in, 2 out]
        n889 = property on="AUTO/MAN 01" class="Bool (strict)"() -> ("Value"=w2561:bool)  [unwired: 2 in, 2 out]
        n890 = shared-variable ".\\D05.lvlib\\projector 05"() -> (w2566:bool)  [unwired: 1 in, 1 out]
        "projector 05" <- w2566
        n891 = Unbundle By Name(w2590) -> ("status"=w2589:bool)
        n892 = Unbundle By Name(w2550) -> ("status"=w2549:bool)
        n893 = shared-variable ".\\D04.lvlib\\projector 04"() -> (w2567:bool)  [unwired: 1 in, 1 out]
        "projector 04" <- w2567
        n894 = property on="DISC 02" class="Bool (strict)"() -> ("Value"=w2573:bool)  [unwired: 2 in, 2 out]
        n895 = Unbundle By Name(w2578) -> ("status"=w2579:bool)
        n896 = shared-variable ".\\D02.lvlib\\projector 02"() -> (w2569:bool)  [unwired: 1 in, 1 out]
        "projector 02" <- w2569
        n897 = shared-variable ".\\D01.lvlib\\projector 01"() -> (w2570:bool)  [unwired: 1 in, 1 out]
        "projector 01" <- w2570
        n898 = Unbundle By Name(w2584) -> ("status"=w2585:bool)
        n899 = Unbundle By Name(w2581) -> ("status"=w2582:bool)
        n900 = Unbundle By Name(w2587) -> ("status"=w2588:bool)
        n901 = To Byte Integer(number=w2529) -> (8bit integer=w2526:i8)
        n902 = shared-variable ".\\D03.lvlib\\projector 03"() -> (w2568:bool)  [unwired: 1 in, 1 out]
        "projector 03" <- w2568
        n903 = property on="DISC 04" class="Bool (strict)"() -> ("Value"=w2575:bool)  [unwired: 2 in, 2 out]
        n904 = property on="DISC 01" class="Bool (strict)"() -> ("Value"=w2571:bool)  [unwired: 2 in, 2 out]
        n905 = property on="DISC 06" class="Bool (strict)"() -> ("Value"=w2551:bool)  [unwired: 2 in, 2 out]
        n906 = property on="DISC 05" class="Bool (strict)"() -> ("Value"=w2576:bool)  [unwired: 2 in, 2 out]
        n907 = Not(x=w2589) -> (.not. x?=w2591:bool)
        "cam 01" <- w2591
        n908 = Not(x=w2549) -> (.not. x?=w2540:bool)
        "cam 06" <- w2540
        n909 = Not(x=w2579) -> (.not. x?=w2577:bool)
        "cam 05" <- w2577
        n910 = Not(x=w2585) -> (.not. x?=w2583:bool)
        "cam 03" <- w2583
        n911 = Not(x=w2582) -> (.not. x?=w2580:bool)
        "cam 04" <- w2580
        n912 = Not(x=w2588) -> (.not. x?=w2586:bool)
        "cam 02" <- w2586
        n913 = shared-variable ".\\Maintenance.lvlib\\error_17"(w2530) -> ()  [unwired: 1 in, 1 out]
        n914 = Build Array(w2540, w2541, TRUE ("element"), w2551) -> (w2548:bool[])
        n915 = call "find and draw circles.vi"("Image Src"=w2532, "module path"=w2536, "function name"=w2535, "initialized array"=w2600, "Image Dst"=w2601, "error in (no error)"=w2530, "session in"=w2599, "Run/Stop"=w2571, "grading Thr"=w2534, "bias"=w2526) -> ("session out"=w2598:refnum<k35>, "circle info"=w2531:dbl[][], "Image Out"=w2597:T9, "error out"=w2533:errorcluster, "pellet detected?"=w2596:bool)  [unwired: 5 in]
        n916 = Build Array(w2577, w2566, TRUE ("element"), w2576) -> (w2603:bool[])
        n917 = Build Array(w2580, w2567, TRUE ("element"), w2575) -> (w2605:bool[])
        n918 = Build Array(w2591, w2570, TRUE ("element"), w2572) -> (w2612:bool[])
        n919 = Build Array(w2583, w2568, TRUE ("element"), w2574) -> (w2607:bool[])
        n920 = Build Array(w2586, w2569, TRUE ("element"), w2573) -> (w2610:bool[])
        n921 = shared-variable ".\\Maintenance.lvlib\\error_22"(w2533) -> ()  [unwired: 1 in, 1 out]
        n922 = And Array Elements(Boolean array=w2607) -> (logical AND=w2619:bool)
        n923 = Not(x=w2548) -> (.not. x?=→"Warning array 06":bool[])
        n924 = Not(x=w2603) -> (.not. x?=→"Warning array 05":bool[])
        n925 = Not(x=w2607) -> (.not. x?=→"Warning array 03":bool[])
        n926 = And Array Elements(Boolean array=w2612) -> (logical AND=w2615:bool)
        n927 = And Array Elements(Boolean array=w2610) -> (logical AND=w2617:bool)
        n928 = And Array Elements(Boolean array=w2605) -> (logical AND=w2620:bool)
        n929 = Not(x=w2619) -> (.not. x?=→"Warning 03":bool)
        n930 = Not(x=w2610) -> (.not. x?=→"Warning array 02":bool[])
        n931 = And Array Elements(Boolean array=w2548) -> (logical AND=w2546:bool)
        n932 = Not(x=w2605) -> (.not. x?=→"Warning array 04":bool[])
        n933 = Not(x=w2612) -> (.not. x?=→"Warning array 01":bool[])
        n934 = And Array Elements(Boolean array=w2603) -> (logical AND=w2622:bool)
        n935 = shared-variable ".\\D01.lvlib\\PelletDetectedD 01"(w2597, error in=w2533) -> (error out=w2602:errorcluster)
        n936 = Bundle By Name(cluster=T2 {"disc 06"=FALSE, "auto/man 06"=FALSE, "projector 06"=FALSE, "cam 06"=FALSE}, "disc 06"=w2551, "auto/man 06"=w2552, "projector 06"=w2541, "cam 06"=w2540) -> (w2544:T2)
        n937 = Bundle By Name(cluster=T3 {"disc 05"=FALSE, "auto/man 05"=FALSE, "projector 05"=FALSE, "cam 05"=FALSE}, "disc 05"=w2576, "auto/man 05"=w2565, "projector 05"=w2566, "cam 05"=w2577) -> (w2626:T3)
        n938 = Bundle By Name(cluster=T6 {"disc 02"=FALSE, "auto/man 02"=FALSE, "projector 02"=FALSE, "cam 02"=FALSE}, "disc 02"=w2573, "auto/man 02"=w2562, "projector 02"=w2569, "cam 02"=w2586) -> (w2643:T6)
        n939 = Bundle By Name(cluster=T4 {"disc 04"=FALSE, "auto/man 04"=FALSE, "projector 04"=FALSE, "cam 04"=FALSE}, "disc 04"=w2575, "auto/man 04"=w2564, "projector 04"=w2567, "cam 04"=w2580) -> (w2639:T4)
        n940 = Bundle By Name(cluster=T7 {"disc 01"=FALSE, "auto/man 01"=FALSE, "projector 01"=FALSE, "cam 01"=FALSE}, "disc 01"=w2572, "auto/man 01"=w2561, "projector 01"=w2570, "cam 01"=w2591) -> (w2648:T7)
        n941 = Bundle By Name(cluster=T5 {"disc 03"=FALSE, "auto/man 03"=FALSE, "projector 03"=FALSE, "cam 03"=FALSE}, "disc 03"=w2574, "auto/man 03"=w2563, "projector 03"=w2568, "cam 03"=w2583) -> (w2636:T5)
        n942 = Not(x=w2615) -> (.not. x?=→"Warning 01":bool)
        n943 = Not(x=w2617) -> (.not. x?=→"Warning 02":bool)
        n944 = Not(x=w2620) -> (.not. x?=→"Warning 04":bool)
        n945 = Not(x=w2546) -> (.not. x?=→"Warning 06":bool)
        n946 = Not(x=w2622) -> (.not. x?=→"Warning 05":bool)
        n947 = Delete From Array(array=w2538, index=1) -> (array with subset deleted=w2545:T12)  [unwired: 1 in, 1 out]
        n948 = Delete From Array(array=w2625, index=1) -> (array with subset deleted=w2624:T13)  [unwired: 1 in, 1 out]
        n949 = Delete From Array(array=w2644, index=1) -> (array with subset deleted=w2641:T11)  [unwired: 1 in, 1 out]
        n950 = Delete From Array(array=w2632, index=1) -> (array with subset deleted=w2640:T15)  [unwired: 1 in, 1 out]
        n951 = Delete From Array(array=w2651, index=1) -> (array with subset deleted=w2649:T10)  [unwired: 1 in, 1 out]
        n952 = Delete From Array(array=w2631, index=1) -> (array with subset deleted=w2635:T14)  [unwired: 1 in, 1 out]
        n953 = Build Array (concatenate)(w2544, w2545) -> (w2537:T12)
        n954 = Build Array (concatenate)(w2648, w2649) -> (w2647:T10)
        n955 = Build Array (concatenate)(w2626, w2624) -> (w2623:T13)
        n956 = Build Array (concatenate)(w2643, w2641) -> (w2642:T11)
        n957 = Build Array (concatenate)(w2639, w2640) -> (w2630:T15)
        n958 = Build Array (concatenate)(w2636, w2635) -> (w2629:T14)
      }
      frame #3 {
        # "Method selection\nMethod 1: threshold calibration (weigth of pelletizes)\nMethod 2: chess calibration (image processing)"
        n959 = shared-variable ".\\Calibration Lib.lvlib\\Method Selection"() -> (w2681:enum32{"Method 1", "Method 2"}, error out=w2673:errorcluster)  [unwired: 1 in]
        n960 = shared-variable ".\\Calibration Lib.lvlib\\calibration matrix D01"(error in=w2673) -> (w2679:dbl[], error out=w2672:errorcluster)
        n961 = Matrix Size(0:w2669) -> (1:w2667:i32)  [unwired: 1 out]
        n962 = property on="DISC 01" class="Bool (strict)"() -> ("Value"=w2665:bool)  [unwired: 2 in, 2 out]
        n963 = Select(t=w2667, s=w2665, f=0) -> (s? t:f=w2666:i32)
        n964 = case shown="\"Method 2\"" w2681 {
          tunnel: w2679 -> [_ w2703]
          tunnel: w2669 -> [w2697 w2702]
          tunnel: [w2697 w2700] -> w2674
          tunnel: w2661 -> [w2696 w2701]
          tunnel: w2672 -> [w2695 w2698]
          tunnel: [w2696 w2699] -> w2671
          tunnel: [w2695 w2698] -> w2670
          frame "Method 1", Default {
          }
          frame "Method 2" {
            n965 = call "pixel2milimetr.vi"("1*3 Transform Matrix"=w2703, "circle array"=w2702, "Error in"=w2701) -> ("calibrated circles"=w2700:dbl[][], "Error out"=w2699:errorcluster)  [unwired: 11 in]
          }
        }
        n966 = shared-variable ".\\D01.lvlib\\number of pellet 01"(w2666) -> ()  [unwired: 1 in, 1 out]
        n967 = shared-variable ".\\Maintenance.lvlib\\error_27"(w2671, error in=w2670) -> ()  [unwired: 1 out]
      }
      frame #4 {
        w2724 = u16 1 items=["Falling Edge", "Rising Edge"] ("trigger slope")
        n968 = case shown="True" w2717 {
          tunnel: w2740 -> [w2750 w2812]
          tunnel: [w2750 w2808] -> w2739
          tunnel: w2738 -> [w2749 w2807]
          tunnel: [w2749 w2803] -> w2737
          tunnel: w2736 -> [w2751 w2802]
          tunnel: [w2751 w2800] -> w2735
          tunnel: [dbl[] [0.0, 0.0, 0.0, 0.0, 0.0, 0.0, 0.0, 0.0] w2763] -> w2716
          tunnel: w2711 -> [_ w2787]
          tunnel: [errorcluster {"status"=FALSE, "code"=0, "source"=""} ("error IO") w2782] -> w2709
          frame False {
          }
          frame True {
            w2754 = dbl[] [250.047, 512.0, 857.375, 1331.0, 2048.0, 2744.0, 4096.0]  # fixed threshoulds
            n969 = shared-variable ".\\D01.lvlib\\GradingThrD01"() -> (w2795:dbl[], error out=w2785:errorcluster)  [unwired: 1 in]
            n970 = Index Array(array=w2787, index (col)=2 ("disabled index (col)")) -> (element=w2786:dbl[])  [unwired: 1 in]
            n971 = property on="live grading array size" class="DigNum (strict)"() -> ("Value"=w2790:i32)  [unwired: 2 in, 2 out]
            n972 = shared-variable ".\\Calibration Lib.lvlib\\Method Selection"(error in=w2785) -> (w2791:enum32{"Method 1", "Method 2"}, error out=w2784:errorcluster)
            n973 = property on="avg grading array size" class="DigNum (strict)"() -> ("Value"=w2789:i32)  [unwired: 2 in, 2 out]
            n974 = Array Size(array=w2786) -> (size(s)=w2801:i32)
            n975 = Subtract(x=w2790, y=w2801) -> (x-y=w2810:i32)
            n976 = Multiply(x=w2754, y=0.125) -> (x*y=w2753:dbl[])
            n977 = Subtract(x=w2789, y=w2801) -> (x-y=w2806:i32)
            n978 = Equal?(x=w2791, y=enum32{"Method 1", "Method 2"}."Method 1" ("Method Selection")) -> (x = y?=w2792:bool)
            n979 = property on="DISC 01" class="Bool (strict)"() -> ("Value"=w2778:bool)  [unwired: 2 in, 2 out]
            n980 = Select(t=w2795, s=w2792, f=w2753) -> (s? t:f=w2794:dbl[])
            n981 = property on="DISC 01" class="Bool (strict)"() -> ("Value"=w2777:bool)  [unwired: 2 in, 2 out]
            n982 = call "array managment.vi"("2D array in"=w2812, "col sel"=0, "cir num"=w2801, "index"=w2810, "subarray"=w2786) -> ("2D array out"=w2808:dbl[][], "1D array out"=w2809:dbl[])  [unwired: 13 in]
            n983 = call "array managment.vi"("2D array in"=w2807, "col sel"=0, "cir num"=w2801, "index"=w2806, "subarray"=w2786) -> ("2D array out"=w2803:dbl[][], "1D array out"=w2804:dbl[])  [unwired: 13 in]
            n984 = call "pelletpercents.vi"("Run/Stop"=w2778, "grading threshoulds"=w2794, "Sorted data"=w2809) -> ("Percentage"=w2798:dbl[])  [unwired: 8 in]
            n985 = call "pelletpercents.vi"("Run/Stop"=w2777, "grading threshoulds"=w2794, "Sorted data"=w2804) -> ("Percentage"=w2779:dbl[])  [unwired: 8 in]
            n986 = Number To Fractional String(number=w2798, precision (6)=i16 3) -> (F-format string=w2796:string[])  [unwired: 2 in]
            n987 = Number To Fractional String(number=w2779, precision (6)=i16 2) -> (F-format string=w2781:string[])  [unwired: 2 in]
            n988 = Fract/Exp String To Number(string=w2796) -> (number=w2763:dbl[])  [unwired: 3 in, 1 out]
            n989 = Fract/Exp String To Number(string=w2781) -> (number=w2752:dbl[])  [unwired: 3 in, 1 out]
            n990 = Index Array(array=w2763, index #1=3 ("index")) -> (element #1=w2776:dbl, element #2=w2773:dbl, element #3=w2774:dbl, element #4=w2775:dbl)  [unwired: 3 in]
            n991 = shared-variable ".\\D01.lvlib\\AvgResultArray"(w2752, error in=w2784) -> (error out=w2783:errorcluster)
            n992 = call "grading average.vi"("input array"=w2752) -> ("avg"=w2757:dbl)  [unwired: 10 in]
            n993 = Add(x=w2776, y=w2773) -> (x+y=w2765:dbl)
            "9.5-12.7 01" <- w2765
            n994 = Add(x=w2774, y=w2775) -> (x+y=w2766:dbl)
            "12.7-16 01" <- w2766
            n995 = Not A Number/Path/Refnum?(number/path/refnum=w2757) -> (NaN/Path/Refnum?=w2759:bool)
            n996 = Select(t=12.0, s=w2759, f=w2757) -> (s? t:f=w2756:dbl)
            "AVG 01" <- w2756
            n997 = property on="DISC 01" class="Bool (strict)"() -> ("Value"=w2762:bool)  [unwired: 2 in, 2 out]
            n998 = shared-variable ".\\D01.lvlib\\liveResultArray"(w2763, error in=w2783) -> (error out=w2782:errorcluster)
            n999 = Add(x=w2766, y=w2765) -> (x+y=→"8-16mm 26":dbl)
            n1000 = Select(t=w2756, s=w2762, f=12.0) -> (s? t:f=w2760:dbl)
            n1001 = Add(x=w2773, y=w2774) -> (x+y=w2772:dbl)
            "10-14 01" <- w2772
            n1002 = call "dif array management.vi"("2D array in"=w2802, "col sel"=0, "new element/subarray"=w2760) -> ("2D array out"=w2800:dbl[][])  [unwired: 15 in, 1 out]
            n1003 = Greater Or Equal?(x=w2772, y=70.0) -> (x >= y?=w2770:bool)
            n1004 = Select(t=u32 65282 ("Fill Color"), s=w2770, f=u32 4018019 ("Fill Color")) -> (s? t:f=w2768:u32)
            n1005 = property on="10-14 01" class="Slide (strict)"("Fill Color"=w2768) -> ()  [unwired: 2 in, 2 out]
          }
        }
        n1006 = shared-variable ".\\Setting Lib.lvlib\\data saving period"() -> (w2710:i32, error out=w2708:errorcluster)  [unwired: 1 in]
        n1007 = Get Date/Time In Seconds() -> (seconds since 1Jan1904=w2734:timestamp)
        n1008 = Seconds To Date/Time(time stamp (now)=w2734) -> (date time rec=w2733:T35)  [unwired: 1 in]
        n1009 = Unbundle By Name(w2733) -> ("minute"=w2732:i32)
        n1010 = Quotient & Remainder(x=w2732, y=w2710) -> (x-y*floor(x/y)=w2731:i32)  [unwired: 1 out]
        n1011 = Equal To 0?(x=w2731) -> (x = 0?=w2730:bool)
        n1012 = Boolean To (0,1)(Boolean=w2730) -> (0, 1=w2729:i16)
        n1013 = Get Date/Time In Seconds() -> (seconds since 1Jan1904=w2727:timestamp)
        n1014 = Build Array(w2729) -> (w2728:i16[])
        n1015 = Bundle By Name("Y"=w2728, "t0"=w2727) -> (w2726:waveform(i16))  [unwired: 1 in]
        n1016 = call-poly <vilib>:"Basic Level Trigger Detection.vi"("signal in"=w2726, "level"=0.5, "error in (no error)"=w2708, "trigger slope"=w2724) -> ("trigger detected?"=w2723:bool, "error out"=w2707:errorcluster)  [unwired: 9 in, 1 out]
      }
      frame #5 {
        n1017 = shared-variable ".\\D01.lvlib\\SaveD01"(error in=w2821) -> (w2831:bool, error out=w2827:errorcluster)
        n1018 = case shown="True" w2842 {
          tunnel: w2828 -> [_ w2877]
          tunnel: w2820 -> [_ w2875]
          frame False {
          }
          frame True {
            w2871 = enum16{"ID Delete", "Time Delete"}."Time Delete" ("Enum")
            n1019 = property on="projector 01" class="Bool (strict)"(error in=w2875) -> ("Value"=w2907:bool)  [unwired: 1 in, 2 out]
            n1020 = Select(t="ON" ("time format string (%c)"), s=w2907, f="OFF" ("time format string (%c)")) -> (s? t:f=w2908:string)
            n1021 = property on="cam 01" class="Bool (strict)"() -> ("Value"=w2905:bool)  [unwired: 2 in, 2 out]
            n1022 = Select(t="ON" ("time format string (%c)"), s=w2905, f="OFF" ("time format string (%c)")) -> (s? t:f=w2906:string)
            n1023 = property on="AUTO/MAN 01" class="Bool (strict)"() -> ("Value"=w2903:bool)  [unwired: 2 in, 2 out]
            n1024 = Select(t="Auto", s=w2903, f="Manual") -> (s? t:f=w2904:string)
            n1025 = property on="DISC 01" class="Bool (strict)"() -> ("Value"=w2901:bool)  [unwired: 2 in, 2 out]
            n1026 = Select(t="Run", s=w2901, f="Stop") -> (s? t:f=w2902:string)
            n1027 = Get Date/Time In Seconds() -> (seconds since 1Jan1904=w2898:timestamp)
            n1028 = Format Date/Time String(time format string (%c)="%Y/%m/%d", seconds (now)=w2898) -> (date/time string=w2899:string)  [unwired: 1 in]
            n1029 = Format Date/Time String(time format string (%c)="%H:%M:%S", seconds (now)=w2898) -> (date/time string=w2900:string)  [unwired: 1 in]
            n1030 = Index Array(array=w2877, index #1=0 ("index")) -> (element #1=w2890:dbl, element #2=w2891:dbl, element #3=w2892:dbl, element #4=w2893:dbl, element #5=w2894:dbl, element #6=w2895:dbl, element #7=w2896:dbl, element #8=w2897:dbl)  [unwired: 7 in]
            n1031 = shared-variable ".\\Setting Lib.lvlib\\database refresh period"() -> (w2876:i32, error out=w2874:errorcluster)  [unwired: 1 in]
            n1032 = Bundle("date/time string"=w2899, "date/time string"=w2900, w2890, w2891, w2892, w2893, w2894, w2895, w2896, w2897, "f"=w2902, "f"=w2904, "time format string (%c)"=w2906, "time format string (%c)"=w2908) -> (w2878:T36)  [unwired: 1 in]
            n1033 = Unbundle(w2878) -> ("date/time string"=w2922:string, "date/time string"=w2921:string, w2920:dbl, w2917:dbl, w2916:dbl, w2919:dbl, "f"=w2914:string, "f"=w2913:string, "time format string (%c)"=w2912:string, "time format string (%c)"=w2909:string)  [unwired: 4 out]
            n1034 = Add(x=w2917, y=w2916) -> (x+y=w2915:dbl)
            n1035 = Compound Arithmetic op=ADD(w2920, w2917, w2916, w2919) -> (w2918:dbl)
            n1036 = To Variant(anything=w2878) -> (Variant=w2923:variant)
            n1037 = call "Database.vi"("Maximum Row"=w2876, "Enum"=w2871, "Delete row?"=TRUE, "Data"=w2923, "Error in"=w2874, "Auto Increment ID?"=TRUE, "Table"="grading_disc_01", "Connection"="dsgs") -> ("Error out"=w2873:errorcluster)  [unwired: 3 in]
            n1038 = Bundle("date/time string"=w2922, "date/time string"=w2921, w2918, w2915, "f"=w2914, "f"=w2913, "time format string (%c)"=w2912, "time format string (%c)"=w2909) -> (w2911:T37)  [unwired: 1 in]
            n1039 = To Variant(anything=w2911) -> (Variant=w2910:variant)
            n1040 = call "Database.vi"("Maximum Row"=w2876, "Enum"=w2871, "Delete row?"=TRUE, "Data"=w2910, "Auto Increment ID?"=TRUE, "Table"="main_grading_group_disc_01", "Connection"="dsgs") -> ("Error out"=w2872:errorcluster)  [unwired: 4 in]
            n1041 = shared-variable ".\\Maintenance.lvlib\\error_32"(w2873) -> ()  [unwired: 1 in, 1 out]
            n1042 = shared-variable ".\\Maintenance.lvlib\\error_33"(w2872) -> ()  [unwired: 1 in, 1 out]
          }
        }
        n1043 = Index Array(array=w2836, index (col)=0 ("disabled index (col)")) -> (element=w2834:dbl[])  [unwired: 1 in]
        n1044 = Boolean To (0,1)(Boolean=w2831) -> (0, 1=w2832:i16)
        n1045 = Build Array(w2832) -> (w2833:i16[])
        n1046 = call-poly <vilib>:"Basic Level Trigger Detection.vi"("signal in"=w2833, "level"=0.5, "error in (no error)"=w2827) -> ("trigger detected?"=w2835:bool, "error out"=w2826:errorcluster)  [unwired: 10 in, 1 out]
        n1047 = case shown="True" w2835 {
          selector: w2835 -> [_ w2866]
          tunnel: [FALSE w2866] -> w2817
          tunnel: w2834 -> [_ w2861]
          tunnel: w2826 -> [w2852 w2854]
          tunnel: [w2852 w2853] -> w2819
          frame False {
          }
          frame True {
            n1048 = Array To Spreadsheet String(array=w2861, 3:"%.2f" ("format string")) -> (spreadsheet string=w2865:string)  [unwired: 1 in]
            n1049 = Get Date/Time In Seconds() -> (seconds since 1Jan1904=w2862:timestamp)
            n1050 = Format Date/Time String(time format string (%c)="%H:%M:%S", seconds (now)=w2862) -> (date/time string=w2864:string)  [unwired: 1 in]
            n1051 = Format Date/Time String(time format string (%c)="%Y/%m/%d", seconds (now)=w2862) -> (date/time string=w2863:string)  [unwired: 1 in]
            n1052 = Bundle("date/time string"=w2863, "date/time string"=w2864, "disc 01", "spreadsheet string"=w2865) -> (w2856:T38)  [unwired: 1 in]
            n1053 = To Variant(anything=w2856) -> (Variant=w2855:variant)
            n1054 = call "Database.vi"("Delete row?"=FALSE, "Data"=w2855, "Error in"=w2854, "Auto Increment ID?"=TRUE, "Table"="thresholds_calibration_table", "Connection"="dsgs") -> ("Error out"=w2853:errorcluster)  [unwired: 5 in]
          }
        }
        n1055 = shared-variable ".\\D01.lvlib\\SaveD01Ok"(w2817) -> ()  [unwired: 1 in, 1 out]
        n1056 = shared-variable ".\\Maintenance.lvlib\\error_42"(w2819) -> (error out=w2818:errorcluster)  [unwired: 1 in]
      }
      frame #6 {
        n1057 = shared-variable ".\\D01.lvlib\\SaveD01"(FALSE ("SaveD26"), error in=w2943) -> (error out=w2942:errorcluster)
        n1058 = case shown="8" "speed disc 26" {
          tunnel: w2942 -> [w2965 w2967 w2983 w2999 w3015]
          tunnel: [w2965 w2966 w2982 w2998 w3014] -> w2945
          frame 0, Default {
          }
          frame 1 {
            n1059 = Get Date/Time In Seconds() -> (seconds since 1Jan1904=w2981:timestamp)
            n1060 = Format Date/Time String(time format string (%c)="%Y/%m/%d", seconds (now)=w2981) -> (date/time string=w2980:string)  [unwired: 1 in]
            n1061 = Format Date/Time String(time format string (%c)="%H:%M:%S", seconds (now)=w2981) -> (date/time string=w2979:string)  [unwired: 1 in]
            n1062 = Bundle("60001", "date/time string"=w2980, "date/time string"=w2979, "Speed signal is changed and applied in disc 26") -> (w2978:T19)  [unwired: 1 in]
            n1063 = To Variant(anything=w2978) -> (Variant=w2977:variant)
            n1064 = call "Database.vi"("Maximum Row"=u64 0 ("Storage Time (Day)"), "Delete row?"=FALSE, "Data"=w2977, "Error in"=w2967, "Auto Increment ID?"=TRUE, "Table"="log_table", "Connection"="dsgs") -> ("Error out"=w2966:errorcluster)  [unwired: 4 in]
          }
          frame 2 {
            n1065 = Get Date/Time In Seconds() -> (seconds since 1Jan1904=w2997:timestamp)
            n1066 = Format Date/Time String(time format string (%c)="%Y/%m/%d", seconds (now)=w2997) -> (date/time string=w2996:string)  [unwired: 1 in]
            n1067 = Format Date/Time String(time format string (%c)="%H:%M:%S", seconds (now)=w2997) -> (date/time string=w2995:string)  [unwired: 1 in]
            n1068 = Bundle("60002", "date/time string"=w2996, "date/time string"=w2995, "Speed signal is changed and applied in disc 26") -> (w2994:T19)  [unwired: 1 in]
            n1069 = To Variant(anything=w2994) -> (Variant=w2993:variant)
            n1070 = call "Database.vi"("Maximum Row"=u64 0 ("Storage Time (Day)"), "Delete row?"=FALSE, "Data"=w2993, "Error in"=w2983, "Auto Increment ID?"=TRUE, "Table"="log_table", "Connection"="dsgs") -> ("Error out"=w2982:errorcluster)  [unwired: 4 in]
          }
          frame 4 {
            n1071 = Get Date/Time In Seconds() -> (seconds since 1Jan1904=w3013:timestamp)
            n1072 = Format Date/Time String(time format string (%c)="%Y/%m/%d", seconds (now)=w3013) -> (date/time string=w3012:string)  [unwired: 1 in]
            n1073 = Format Date/Time String(time format string (%c)="%H:%M:%S", seconds (now)=w3013) -> (date/time string=w3011:string)  [unwired: 1 in]
            n1074 = Bundle("60003", "date/time string"=w3012, "date/time string"=w3011, "Speed signal is changed but not applied in disc 26") -> (w3010:T19)  [unwired: 1 in]
            n1075 = To Variant(anything=w3010) -> (Variant=w3009:variant)
            n1076 = call "Database.vi"("Maximum Row"=u64 0 ("Storage Time (Day)"), "Delete row?"=FALSE, "Data"=w3009, "Error in"=w2999, "Auto Increment ID?"=TRUE, "Table"="log_table", "Connection"="dsgs") -> ("Error out"=w2998:errorcluster)  [unwired: 4 in]
          }
          frame 8 {
            n1077 = Get Date/Time In Seconds() -> (seconds since 1Jan1904=w3029:timestamp)
            n1078 = Format Date/Time String(time format string (%c)="%Y/%m/%d", seconds (now)=w3029) -> (date/time string=w3028:string)  [unwired: 1 in]
            n1079 = Format Date/Time String(time format string (%c)="%H:%M:%S", seconds (now)=w3029) -> (date/time string=w3027:string)  [unwired: 1 in]
            n1080 = Bundle("60004", "date/time string"=w3028, "date/time string"=w3027, "Speed signal is changed but not applied in disc 26") -> (w3026:T19)  [unwired: 1 in]
            n1081 = To Variant(anything=w3026) -> (Variant=w3025:variant)
            n1082 = call "Database.vi"("Maximum Row"=u64 0 ("Storage Time (Day)"), "Delete row?"=FALSE, "Data"=w3025, "Error in"=w3015, "Auto Increment ID?"=TRUE, "Table"="log_table", "Connection"="dsgs") -> ("Error out"=w3014:errorcluster)  [unwired: 4 in]
          }
        }
        n1083 = shared-variable ".\\control setting.lvlib\\bias"() -> (w2933:dbl[])  [unwired: 1 in, 1 out]
        n1084 = shared-variable ".\\Setting Lib.lvlib\\processing file path"() -> (w2937:path, error out=w2938:errorcluster)  [unwired: 1 in]
        n1085 = shared-variable ".\\Maintenance.lvlib\\error_47"(w2945) -> ()  [unwired: 1 in, 1 out]
        n1086 = Index Array(array=w2933, index=1) -> (element=w2935:dbl)
        n1087 = To Byte Integer(number=w2935) -> (8bit integer=w2932:i8)
      }
      frame #7 {
        n1088 = shared-variable ".\\D02.lvlib\\LiveViewD02"(error in=w3035) -> (w3042:refnum<image>, error out=w3041:errorcluster)
        n1089 = property on="DISC 02" class="Bool (strict)" props=["Value"]() -> ()  [unwired: 2 in, 3 out]
        n1090 = shared-variable ".\\D02.lvlib\\GradingThrD02"() -> (w3043:dbl[])  [unwired: 1 in, 1 out]
        n1091 = call "IMAQ Copy"("error in (no error)"=w3041, "Image Dst"=w3049, "Image Src"=w3042) -> ("error out"=w3034:errorcluster, "Image Dst Out"=w3032:T9)  [unwired: 3 in]
        n1092 = call "find and draw circles.vi"("Image Src"=w3032, "module path"=w3037, "function name"="get_circels", "initialized array"=w3059, "Image Dst"=w3056, "error in (no error)"=w3034, "session in"=w3065, "Run/Stop"=TRUE, "grading Thr"=w3043, "bias"=w3030) -> ("session out"=w3064:refnum<k35>, "circle info"=w3031:dbl[][], "Image Out"=w3066:T9, "error out"=w3036:errorcluster, "pellet detected?"=w3045:bool)  [unwired: 5 in]
        n1093 = shared-variable ".\\Maintenance.lvlib\\error_18"(w3034) -> ()  [unwired: 1 in, 1 out]
        n1094 = shared-variable ".\\Maintenance.lvlib\\error_23"(w3036) -> ()  [unwired: 1 in, 1 out]
        n1095 = shared-variable ".\\D02.lvlib\\PelletDetectedD02"(w3066, error in=w3036) -> (error out=w3044:errorcluster)
      }
      frame #8 {
        n1096 = shared-variable ".\\Calibration Lib.lvlib\\calibration matrix D02"() -> (w3074:dbl[], error out=w3082:errorcluster)  [unwired: 1 in]
        n1097 = Matrix Size(0:w3079) -> (1:w3077:i32)  [unwired: 1 out]
        n1098 = property on="DISC 02" class="Bool (strict)"() -> ("Value"=w3076:bool)  [unwired: 2 in, 2 out]
        n1099 = Select(t=w3077, s=w3076, f=0) -> (s? t:f=w3075:i32)
        n1100 = shared-variable ".\\Calibration Lib.lvlib\\Method Selection"(error in=w3082) -> (w3085:enum32{"Method 1", "Method 2"}, error out=w3080:errorcluster)
        n1101 = shared-variable ".\\D02.lvlib\\number of pellet 02"(w3075) -> ()  [unwired: 1 in, 1 out]
        n1102 = case shown="\"Method 2\"" w3085 {
          tunnel: w3074 -> [_ w3110]
          tunnel: w3079 -> [w3104 w3109]
          tunnel: [w3104 w3107] -> w3084
          tunnel: w3070 -> [w3103 w3108]
          tunnel: [w3103 w3106] -> w3068
          tunnel: [w3102 w3105] -> w3081
          tunnel: w3080 -> [w3102 w3105]
          frame "Method 1", Default {
          }
          frame "Method 2" {
            n1103 = call "pixel2milimetr.vi"("1*3 Transform Matrix"=w3110, "circle array"=w3109, "Error in"=w3108) -> ("calibrated circles"=w3107:dbl[][], "Error out"=w3106:errorcluster)  [unwired: 11 in]
          }
        }
        n1104 = shared-variable ".\\Maintenance.lvlib\\error_28"(w3068, error in=w3081) -> ()  [unwired: 1 out]
      }
      frame #9 {
        n1105 = case shown="True" w3116 {
          tunnel: w3133 -> [_ w3205]
          tunnel: w3132 -> [w3142 w3202]
          tunnel: [w3142 w3201] -> w3131
          tunnel: w3130 -> [w3143 w3196]
          tunnel: [w3143 w3195] -> w3129
          tunnel: w3128 -> [w3141 w3192]
          tunnel: [w3141 w3191] -> w3127
          tunnel: [dbl[] [0.0, 0.0, 0.0, 0.0, 0.0, 0.0, 0.0, 0.0] w3156] -> w3117
          tunnel: [errorcluster {"status"=FALSE, "code"=0, "source"=""} ("error IO") w3175] -> w3115
          tunnel: w3111 -> [_ w3148]
          frame False {
          }
          frame True {
            w3146 = dbl[] [250.047, 512.0, 857.375, 1331.0, 2048.0, 2744.0, 4096.0]  # fixed threshoulds
            n1106 = shared-variable ".\\D02.lvlib\\GradingThrD02"(error in=w3148) -> (w3180:dbl[], error out=w3178:errorcluster)
            n1107 = Index Array(array=w3205, index (col)=2 ("disabled index (col)")) -> (element=w3193:dbl[])  [unwired: 1 in]
            n1108 = property on="live grading array size" class="DigNum (strict)"() -> ("Value"=w3185:i32)  [unwired: 2 in, 2 out]
            n1109 = property on="avg grading array size" class="DigNum (strict)"() -> ("Value"=w3184:i32)  [unwired: 2 in, 2 out]
            n1110 = shared-variable ".\\Calibration Lib.lvlib\\Method Selection"(error in=w3178) -> (w3181:enum32{"Method 1", "Method 2"}, error out=w3177:errorcluster)
            n1111 = Array Size(array=w3193) -> (size(s)=w3194:i32)
            n1112 = Subtract(x=w3185, y=w3194) -> (x-y=w3204:i32)
            n1113 = Subtract(x=w3184, y=w3194) -> (x-y=w3197:i32)
            n1114 = Multiply(x=w3146, y=0.125) -> (x*y=w3145:dbl[])
            n1115 = Equal?(x=w3181, y=enum32{"Method 1", "Method 2"}."Method 1" ("Method Selection")) -> (x = y?=w3182:bool)
            n1116 = property on="DISC 02" class="Bool (strict)"() -> ("Value"=w3171:bool)  [unwired: 2 in, 2 out]
            n1117 = property on="DISC 02" class="Bool (strict)"() -> ("Value"=w3170:bool)  [unwired: 2 in, 2 out]
            n1118 = call "array managment.vi"("2D array in"=w3202, "col sel"=1, "cir num"=w3194, "index"=w3204, "subarray"=w3193) -> ("2D array out"=w3201:dbl[][], "1D array out"=w3200:dbl[])  [unwired: 13 in]
            n1119 = call "array managment.vi"("2D array in"=w3196, "col sel"=1, "cir num"=w3194, "index"=w3197, "subarray"=w3193) -> ("2D array out"=w3195:dbl[][], "1D array out"=w3199:dbl[])  [unwired: 13 in]
            n1120 = Select(t=w3180, s=w3182, f=w3145) -> (s? t:f=w3179:dbl[])
            n1121 = call "pelletpercents.vi"("Run/Stop"=w3170, "grading threshoulds"=w3179, "Sorted data"=w3200) -> ("Percentage"=w3186:dbl[])  [unwired: 8 in]
            n1122 = call "pelletpercents.vi"("Run/Stop"=w3171, "grading threshoulds"=w3179, "Sorted data"=w3199) -> ("Percentage"=w3172:dbl[])  [unwired: 8 in]
            n1123 = Number To Fractional String(number=w3172, precision (6)=i16 2) -> (F-format string=w3174:string[])  [unwired: 2 in]
            n1124 = Number To Fractional String(number=w3186, precision (6)=i16 2) -> (F-format string=w3187:string[])  [unwired: 2 in]
            n1125 = Fract/Exp String To Number(string=w3174) -> (number=w3144:dbl[])  [unwired: 3 in, 1 out]
            n1126 = Fract/Exp String To Number(string=w3187) -> (number=w3156:dbl[])  [unwired: 3 in, 1 out]
            n1127 = call "grading average.vi"("input array"=w3144) -> ("avg"=w3153:dbl)  [unwired: 10 in]
            "AVG 02" <- w3153
            n1128 = property on="DISC 02" class="Bool (strict)"() -> ("Value"=w3152:bool)  [unwired: 2 in, 2 out]
            n1129 = Index Array(array=w3156, index #1=3 ("index")) -> (element #1=w3169:dbl, element #2=w3166:dbl, element #3=w3167:dbl, element #4=w3168:dbl)  [unwired: 3 in]
            n1130 = Not A Number/Path/Refnum?(number/path/refnum=w3153) -> (NaN/Path/Refnum?=w3150:bool)
            n1131 = shared-variable ".\\D02.lvlib\\AvgResultD02"(w3144, error in=w3177) -> (error out=w3176:errorcluster)
            n1132 = Not(x=w3150) -> (.not. x?=w3149:bool)
            n1133 = Add(x=w3169, y=w3166) -> (x+y=w3158:dbl)
            "9.5-12.7 02" <- w3158
            n1134 = Add(x=w3167, y=w3168) -> (x+y=w3159:dbl)
            "12.7-16 02" <- w3159
            n1135 = And(x=w3152, y=w3149) -> (x .and. y?=w3151:bool)
            n1136 = Select(t=w3153, s=w3151, f=12.0) -> (s? t:f=w3154:dbl)
            n1137 = Add(x=w3159, y=w3158) -> (x+y=→"8-16mm 27":dbl)
            n1138 = Add(x=w3166, y=w3167) -> (x+y=w3161:dbl)
            "10-14 02" <- w3161
            n1139 = shared-variable ".\\D02.lvlib\\LiveResultD02"(w3156, error in=w3176) -> (error out=w3175:errorcluster)
            n1140 = call "dif array management.vi"("2D array in"=w3192, "col sel"=1, "new element/subarray"=w3154) -> ("2D array out"=w3191:dbl[][])  [unwired: 15 in, 1 out]
            n1141 = Greater Or Equal?(x=w3161, y=70.0) -> (x >= y?=w3164:bool)
            n1142 = Select(t=u32 65282 ("Fill Color"), s=w3164, f=u32 4018019 ("Fill Color")) -> (s? t:f=w3160:u32)
            n1143 = property on="10-14 02" class="Slide (strict)"("Fill Color"=w3160) -> ()  [unwired: 2 in, 2 out]
          }
        }
      }
      frame #10 {
        n1144 = case shown="True" w3233 {
          tunnel: w3224 -> [_ w3267]
          frame False {
          }
          frame True {
            w3261 = enum16{"ID Delete", "Time Delete"}."Time Delete" ("Enum")
            n1145 = property on="projector 02" class="Bool (strict)"() -> ("Value"=w3296:bool)  [unwired: 2 in, 2 out]
            n1146 = Select(t="ON" ("time format string (%c)"), s=w3296, f="OFF" ("time format string (%c)")) -> (s? t:f=w3297:string)
            n1147 = property on="cam 02" class="Bool (strict)"() -> ("Value"=w3294:bool)  [unwired: 2 in, 2 out]
            n1148 = Select(t="ON" ("time format string (%c)"), s=w3294, f="OFF" ("time format string (%c)")) -> (s? t:f=w3295:string)
            n1149 = property on="AUTO/MAN 02" class="Bool (strict)"() -> ("Value"=w3292:bool)  [unwired: 2 in, 2 out]
            n1150 = Select(t="Auto", s=w3292, f="Manual") -> (s? t:f=w3293:string)
            n1151 = property on="DISC 02" class="Bool (strict)"() -> ("Value"=w3290:bool)  [unwired: 2 in, 2 out]
            n1152 = Select(t="Run", s=w3290, f="Stop") -> (s? t:f=w3291:string)
            n1153 = Get Date/Time In Seconds() -> (seconds since 1Jan1904=w3287:timestamp)
            n1154 = Format Date/Time String(time format string (%c)="%Y/%m/%d", seconds (now)=w3287) -> (date/time string=w3288:string)  [unwired: 1 in]
            n1155 = Format Date/Time String(time format string (%c)="%H:%M:%S", seconds (now)=w3287) -> (date/time string=w3289:string)  [unwired: 1 in]
            n1156 = Index Array(array=w3267, index #1=0 ("index")) -> (element #1=w3279:dbl, element #2=w3280:dbl, element #3=w3281:dbl, element #4=w3282:dbl, element #5=w3283:dbl, element #6=w3284:dbl, element #7=w3285:dbl, element #8=w3286:dbl)  [unwired: 7 in]
            n1157 = shared-variable ".\\Setting Lib.lvlib\\database refresh period"() -> (w3265:i32, error out=w3264:errorcluster)  [unwired: 1 in]
            n1158 = Bundle("date/time string"=w3288, "date/time string"=w3289, w3279, w3280, w3281, w3282, w3283, w3284, w3285, w3286, "f"=w3291, "f"=w3293, "time format string (%c)"=w3295, "time format string (%c)"=w3297) -> (w3266:T36)  [unwired: 1 in]
            n1159 = Unbundle(w3266) -> ("date/time string"=w3299:string, "date/time string"=w3300:string, w3301:dbl, w3304:dbl, w3305:dbl, w3302:dbl, "f"=w3307:string, "f"=w3308:string, "time format string (%c)"=w3309:string, "time format string (%c)"=w3310:string)  [unwired: 4 out]
            n1160 = Add(x=w3304, y=w3305) -> (x+y=w3306:dbl)
            n1161 = Compound Arithmetic op=ADD(w3301, w3304, w3305, w3302) -> (w3303:dbl)
            n1162 = To Variant(anything=w3266) -> (Variant=w3312:variant)
            n1163 = call "Database.vi"("Maximum Row"=w3265, "Enum"=w3261, "Delete row?"=TRUE, "Data"=w3312, "Error in"=w3264, "Auto Increment ID?"=TRUE, "Table"="grading_disc_02", "Connection"="dsgs") -> ("Error out"=w3262:errorcluster)  [unwired: 3 in]
            n1164 = Bundle("date/time string"=w3299, "date/time string"=w3300, w3303, w3306, "f"=w3307, "f"=w3308, "time format string (%c)"=w3309, "time format string (%c)"=w3310) -> (w3311:T37)  [unwired: 1 in]
            n1165 = shared-variable ".\\Maintenance.lvlib\\error_34"(w3262) -> ()  [unwired: 1 in, 1 out]
            n1166 = To Variant(anything=w3311) -> (Variant=w3298:variant)
            n1167 = call "Database.vi"("Maximum Row"=w3265, "Enum"=w3261, "Delete row?"=TRUE, "Data"=w3298, "Auto Increment ID?"=TRUE, "Table"="main_grading_group_disc_02", "Connection"="dsgs") -> ("Error out"=w3263:errorcluster)  [unwired: 4 in]
            n1168 = shared-variable ".\\Maintenance.lvlib\\error_35"(w3263) -> ()  [unwired: 1 in, 1 out]
          }
        }
        n1169 = shared-variable ".\\D02.lvlib\\SaveD02"(error in=w3212) -> (w3218:bool, error out=w3215:errorcluster)
        n1170 = Index Array(array=w3213, index (col)=1 ("disabled index (col)")) -> (element=w3221:dbl[])  [unwired: 1 in]
        n1171 = Boolean To (0,1)(Boolean=w3218) -> (0, 1=w3219:i16)
        n1172 = Build Array(w3219) -> (w3220:i16[])
        n1173 = call-poly <vilib>:"Basic Level Trigger Detection.vi"("signal in"=w3220, "level"=0.5, "error in (no error)"=w3215) -> ("trigger detected?"=w3223:bool, "error out"=w3214:errorcluster)  [unwired: 10 in, 1 out]
        n1174 = case shown="True" w3223 {
          selector: w3223 -> [_ w3256]
          tunnel: [FALSE w3256] -> w3222
          tunnel: w3221 -> [_ w3251]
          tunnel: w3214 -> [w3242 w3244]
          tunnel: [w3242 w3243] -> w3210
          frame False {
          }
          frame True {
            n1175 = Array To Spreadsheet String(array=w3251, 3:"%.2f" ("format string")) -> (spreadsheet string=w3255:string)  [unwired: 1 in]
            n1176 = Get Date/Time In Seconds() -> (seconds since 1Jan1904=w3252:timestamp)
            n1177 = Format Date/Time String(time format string (%c)="%H:%M:%S", seconds (now)=w3252) -> (date/time string=w3254:string)  [unwired: 1 in]
            n1178 = Format Date/Time String(time format string (%c)="%Y/%m/%d", seconds (now)=w3252) -> (date/time string=w3253:string)  [unwired: 1 in]
            n1179 = Bundle("date/time string"=w3253, "date/time string"=w3254, "disc 02", "spreadsheet string"=w3255) -> (w3246:T38)  [unwired: 1 in]
            n1180 = To Variant(anything=w3246) -> (Variant=w3245:variant)
            n1181 = call "Database.vi"("Delete row?"=FALSE, "Data"=w3245, "Error in"=w3244, "Auto Increment ID?"=TRUE, "Table"="thresholds_calibration_table", "Connection"="dsgs") -> ("Error out"=w3243:errorcluster)  [unwired: 5 in]
          }
        }
        n1182 = shared-variable ".\\D02.lvlib\\SaveD02Ok"(w3222, error in=w3210) -> (error out=w3211:errorcluster)
        n1183 = shared-variable ".\\Maintenance.lvlib\\error_43"(w3210) -> ()  [unwired: 1 in, 1 out]
      }
      frame #11 {
        n1184 = shared-variable ".\\D02.lvlib\\SaveD02"(FALSE ("SaveD27"), error in=w3333) -> (error out=w3332:errorcluster)
        n1185 = case shown="8" "speed disc 27" {
          tunnel: w3332 -> [w3352 w3354 w3370 w3386 w3402]
          tunnel: [w3352 w3353 w3369 w3385 w3401] -> w3334
          frame 0, Default {
          }
          frame 1 {
            n1186 = Get Date/Time In Seconds() -> (seconds since 1Jan1904=w3368:timestamp)
            n1187 = Format Date/Time String(time format string (%c)="%Y/%m/%d", seconds (now)=w3368) -> (date/time string=w3367:string)  [unwired: 1 in]
            n1188 = Format Date/Time String(time format string (%c)="%H:%M:%S", seconds (now)=w3368) -> (date/time string=w3366:string)  [unwired: 1 in]
            n1189 = Bundle("60001", "date/time string"=w3367, "date/time string"=w3366, "Speed signal is changed and applied in disc 27") -> (w3365:T19)  [unwired: 1 in]
            n1190 = To Variant(anything=w3365) -> (Variant=w3364:variant)
            n1191 = call "Database.vi"("Maximum Row"=u64 0 ("Storage Time (Day)"), "Delete row?"=FALSE, "Data"=w3364, "Error in"=w3354, "Auto Increment ID?"=TRUE, "Table"="log_table", "Connection"="dsgs") -> ("Error out"=w3353:errorcluster)  [unwired: 4 in]
          }
          frame 2 {
            n1192 = Get Date/Time In Seconds() -> (seconds since 1Jan1904=w3384:timestamp)
            n1193 = Format Date/Time String(time format string (%c)="%Y/%m/%d", seconds (now)=w3384) -> (date/time string=w3383:string)  [unwired: 1 in]
            n1194 = Format Date/Time String(time format string (%c)="%H:%M:%S", seconds (now)=w3384) -> (date/time string=w3382:string)  [unwired: 1 in]
            n1195 = Bundle("60002", "date/time string"=w3383, "date/time string"=w3382, "Speed signal is changed and applied in disc 27") -> (w3381:T19)  [unwired: 1 in]
            n1196 = To Variant(anything=w3381) -> (Variant=w3380:variant)
            n1197 = call "Database.vi"("Maximum Row"=u64 0 ("Storage Time (Day)"), "Delete row?"=FALSE, "Data"=w3380, "Error in"=w3370, "Auto Increment ID?"=TRUE, "Table"="log_table", "Connection"="dsgs") -> ("Error out"=w3369:errorcluster)  [unwired: 4 in]
          }
          frame 4 {
            n1198 = Get Date/Time In Seconds() -> (seconds since 1Jan1904=w3400:timestamp)
            n1199 = Format Date/Time String(time format string (%c)="%Y/%m/%d", seconds (now)=w3400) -> (date/time string=w3399:string)  [unwired: 1 in]
            n1200 = Format Date/Time String(time format string (%c)="%H:%M:%S", seconds (now)=w3400) -> (date/time string=w3398:string)  [unwired: 1 in]
            n1201 = Bundle("60003", "date/time string"=w3399, "date/time string"=w3398, "Speed signal is changed but not applied in disc 27") -> (w3397:T19)  [unwired: 1 in]
            n1202 = To Variant(anything=w3397) -> (Variant=w3396:variant)
            n1203 = call "Database.vi"("Maximum Row"=u64 0 ("Storage Time (Day)"), "Delete row?"=FALSE, "Data"=w3396, "Error in"=w3386, "Auto Increment ID?"=TRUE, "Table"="log_table", "Connection"="dsgs") -> ("Error out"=w3385:errorcluster)  [unwired: 4 in]
          }
          frame 8 {
            n1204 = Get Date/Time In Seconds() -> (seconds since 1Jan1904=w3416:timestamp)
            n1205 = Format Date/Time String(time format string (%c)="%Y/%m/%d", seconds (now)=w3416) -> (date/time string=w3415:string)  [unwired: 1 in]
            n1206 = Format Date/Time String(time format string (%c)="%H:%M:%S", seconds (now)=w3416) -> (date/time string=w3414:string)  [unwired: 1 in]
            n1207 = Bundle("60004", "date/time string"=w3415, "date/time string"=w3414, "Speed signal is changed but not applied in disc 27") -> (w3413:T19)  [unwired: 1 in]
            n1208 = To Variant(anything=w3413) -> (Variant=w3412:variant)
            n1209 = call "Database.vi"("Maximum Row"=u64 0 ("Storage Time (Day)"), "Delete row?"=FALSE, "Data"=w3412, "Error in"=w3402, "Auto Increment ID?"=TRUE, "Table"="log_table", "Connection"="dsgs") -> ("Error out"=w3401:errorcluster)  [unwired: 4 in]
          }
        }
        n1210 = shared-variable ".\\D03.lvlib\\LiveViewD03"() -> (w3326:refnum<image>, error out=w3325:errorcluster)  [unwired: 1 in]
        n1211 = shared-variable ".\\control setting.lvlib\\bias"() -> (w3322:dbl[])  [unwired: 1 in, 1 out]
        n1212 = Index Array(array=w3322, index=2) -> (element=w3324:dbl)
        n1213 = shared-variable ".\\Maintenance.lvlib\\error_48"(w3334) -> ()  [unwired: 1 in, 1 out]
        n1214 = To Byte Integer(number=w3324) -> (8bit integer=w3321:i8)
      }
      frame #12 {
        n1215 = shared-variable ".\\Setting Lib.lvlib\\processing file path"() -> (w3421:path, error out=w3428:errorcluster)  [unwired: 1 in]
        n1216 = shared-variable ".\\D03.lvlib\\GradingThrD03"() -> (w3427:dbl[], error out=w3426:errorcluster)  [unwired: 1 in]
        n1217 = call "IMAQ Copy"("error in (no error)"=w3418, "Image Dst"=w3435, "Image Src"=w3419) -> ("error out"=w3431:errorcluster, "Image Dst Out"=w3420:T9)  [unwired: 3 in]
        n1218 = property on="DISC 03" class="Bool (strict)"() -> ("Value"=w3425:bool)  [unwired: 2 in, 2 out]
        n1219 = shared-variable ".\\Maintenance.lvlib\\error_19"(w3431) -> ()  [unwired: 1 in, 1 out]
        n1220 = call "find and draw circles.vi"("Image Src"=w3420, "module path"=w3421, "function name"="get_circels", "initialized array"=w3449, "Image Dst"=w3442, "error in (no error)"=w3428, "session in"=w3451, "Run/Stop"=w3425, "grading Thr"=w3427, "bias"=w3417) -> ("session out"=w3450:refnum<k35>, "circle info"=w3445:dbl[][], "Image Out"=w3453:T9, "error out"=w3430:errorcluster, "pellet detected?"=w3432:bool)  [unwired: 5 in]
        n1221 = shared-variable ".\\Maintenance.lvlib\\error_24"(w3430) -> ()  [unwired: 1 in, 1 out]
        n1222 = shared-variable ".\\D03.lvlib\\PelletDetectedD03"(w3453, error in=w3426) -> (error out=w3429:errorcluster)
      }
      frame #13 {
        n1223 = shared-variable ".\\Calibration Lib.lvlib\\calibration matrix D03"() -> (w3472:dbl[], error out=w3468:errorcluster)  [unwired: 1 in]
        n1224 = shared-variable ".\\Calibration Lib.lvlib\\calibration factor D03"(error in=w3465) -> (w3471:sgl, error out=w3466:errorcluster)
        n1225 = Matrix Size(0:w3462) -> (1:w3460:i32)  [unwired: 1 out]
        n1226 = property on="DISC 03" class="Bool (strict)"() -> ("Value"=w3458:bool)  [unwired: 2 in, 2 out]
        n1227 = shared-variable ".\\Calibration Lib.lvlib\\Method Selection"(error in=w3468) -> (w3473:enum32{"Method 1", "Method 2"}, error out=w3467:errorcluster)
        n1228 = Select(t=w3460, s=w3458, f=0) -> (s? t:f=w3459:i32)
        n1229 = case shown="\"Method 1\", Default" w3473 {
          tunnel: w3472 -> [_ w3496]
          tunnel: w3471 -> [_ _]
          tunnel: w3462 -> [w3490 w3495]
          tunnel: [w3490 w3493] -> w3470
          tunnel: w3466 -> [w3489 w3494]
          tunnel: [w3489 w3492] -> w3464
          tunnel: w3467 -> [w3488 w3491]
          tunnel: [w3488 w3491] -> w3463
          frame "Method 1", Default {
          }
          frame "Method 2" {
            n1230 = call "pixel2milimetr.vi"("1*3 Transform Matrix"=w3496, "circle array"=w3495, "Error in"=w3494) -> ("calibrated circles"=w3493:dbl[][], "Error out"=w3492:errorcluster)  [unwired: 11 in]
          }
        }
        n1231 = shared-variable ".\\D03.lvlib\\number of pellet 03"(w3459) -> ()  [unwired: 1 in, 1 out]
        n1232 = shared-variable ".\\Maintenance.lvlib\\error_29"(w3464, error in=w3463) -> ()  [unwired: 1 out]
      }
      frame #14 {
        n1233 = case shown="True" w3501 {
          tunnel: w3517 -> [_ w3587]
          tunnel: w3516 -> [w3525 w3583]
          tunnel: [w3525 w3582] -> w3515
          tunnel: w3514 -> [w3524 w3578]
          tunnel: [w3524 w3577] -> w3513
          tunnel: w3512 -> [w3526 w3574]
          tunnel: [w3526 w3572] -> w3511
          tunnel: [dbl[] [0.0, 0.0, 0.0, 0.0, 0.0, 0.0, 0.0, 0.0] w3538] -> w3502
          tunnel: [errorcluster {"status"=FALSE, "code"=0, "source"=""} ("error IO") w3557] -> w3500
          frame False {
          }
          frame True {
            w3529 = dbl[] [250.047, 512.0, 857.375, 1331.0, 2048.0, 2744.0, 3500.0]  # fixed threshoulds
            n1234 = shared-variable ".\\Calibration Lib.lvlib\\Method Selection"() -> (w3563:enum32{"Method 1", "Method 2"}, error out=w3559:errorcluster)  [unwired: 1 in]
            n1235 = Index Array(array=w3587, index (col)=2 ("disabled index (col)")) -> (element=w3575:dbl[])  [unwired: 1 in]
            n1236 = Array Size(array=w3575) -> (size(s)=w3576:i32)
            n1237 = property on="avg grading array size" class="DigNum (strict)"() -> ("Value"=w3567:i32)  [unwired: 2 in, 2 out]
            n1238 = property on="live grading array size" class="DigNum (strict)"() -> ("Value"=w3566:i32)  [unwired: 2 in, 2 out]
            n1239 = shared-variable ".\\D03.lvlib\\GradingThrD03"(error in=w3559) -> (w3562:dbl[], error out=w3558:errorcluster)
            n1240 = Subtract(x=w3566, y=w3576) -> (x-y=w3586:i32)
            n1241 = Subtract(x=w3567, y=w3576) -> (x-y=w3581:i32)
            n1242 = Multiply(x=w3529, y=0.125) -> (x*y=w3528:dbl[])
            n1243 = Equal?(x=w3563, y=enum32{"Method 1", "Method 2"}."Method 1" ("Method Selection")) -> (x = y?=w3564:bool)
            n1244 = Select(t=w3562, s=w3564, f=w3528) -> (s? t:f=w3561:dbl[])
            n1245 = property on="DISC 03" class="Bool (strict)"() -> ("Value"=w3553:bool)  [unwired: 2 in, 2 out]
            n1246 = call "array managment.vi"("2D array in"=w3583, "col sel"=2, "cir num"=w3576, "index"=w3586, "subarray"=w3575) -> ("2D array out"=w3582:dbl[][], "1D array out"=w3585:dbl[])  [unwired: 13 in]
            n1247 = call "array managment.vi"("2D array in"=w3578, "col sel"=2, "cir num"=w3576, "index"=w3581, "subarray"=w3575) -> ("2D array out"=w3577:dbl[][], "1D array out"=w3579:dbl[])  [unwired: 13 in]
            n1248 = property on="DISC 03" class="Bool (strict)"() -> ("Value"=w3552:bool)  [unwired: 2 in, 2 out]
            n1249 = call "pelletpercents.vi"("Run/Stop"=w3553, "grading threshoulds"=w3561, "Sorted data"=w3585) -> ("Percentage"=w3568:dbl[])  [unwired: 8 in]
            n1250 = call "pelletpercents.vi"("Run/Stop"=w3552, "grading threshoulds"=w3561, "Sorted data"=w3579) -> ("Percentage"=w3554:dbl[])  [unwired: 8 in]
            n1251 = Number To Fractional String(number=w3568, precision (6)=i16 2) -> (F-format string=w3569:string[])  [unwired: 2 in]
            n1252 = Number To Fractional String(number=w3554, precision (6)=i16 2) -> (F-format string=w3556:string[])  [unwired: 2 in]
            n1253 = Fract/Exp String To Number(string=w3569) -> (number=w3538:dbl[])  [unwired: 3 in, 1 out]
            n1254 = property on="DISC 03" class="Bool (strict)"() -> ("Value"=w3534:bool)  [unwired: 2 in, 2 out]
            n1255 = Fract/Exp String To Number(string=w3556) -> (number=w3527:dbl[])  [unwired: 3 in, 1 out]
            n1256 = call "grading average.vi"("input array"=w3527) -> ("avg"=w3535:dbl)  [unwired: 10 in]
            "AVG 03" <- w3535
            n1257 = Not A Number/Path/Refnum?(number/path/refnum=w3535) -> (NaN/Path/Refnum?=w3532:bool)
            n1258 = shared-variable ".\\D03.lvlib\\AvgResultD03"(w3527, error in=w3558) -> (error out=w3560:errorcluster)
            n1259 = Not(x=w3532) -> (.not. x?=w3531:bool)
            n1260 = Index Array(array=w3538, index #1=3 ("index")) -> (element #1=w3551:dbl, element #2=w3548:dbl, element #3=w3549:dbl, element #4=w3550:dbl)  [unwired: 3 in]
            n1261 = And(x=w3534, y=w3531) -> (x .and. y?=w3533:bool)
            n1262 = Select(t=w3535, s=w3533, f=12.0) -> (s? t:f=w3536:dbl)
            n1263 = Add(x=w3551, y=w3548) -> (x+y=w3540:dbl)
            "9.5-12.7 03" <- w3540
            n1264 = Add(x=w3549, y=w3550) -> (x+y=w3541:dbl)
            "12.7-16 03" <- w3541
            n1265 = Add(x=w3548, y=w3549) -> (x+y=w3543:dbl)
            "10-14 03" <- w3543
            n1266 = shared-variable ".\\D03.lvlib\\LiveResultD03"(w3538, error in=w3560) -> (error out=w3557:errorcluster)
            n1267 = Add(x=w3541, y=w3540) -> (x+y=→"8-16mm 03":dbl)
            n1268 = call "dif array management.vi"("2D array in"=w3574, "col sel"=2, "new element/subarray"=w3536) -> ("2D array out"=w3572:dbl[][])  [unwired: 15 in, 1 out]
            n1269 = Greater Or Equal?(x=w3543, y=70.0) -> (x >= y?=w3546:bool)
            n1270 = Select(t=u32 65282 ("Fill Color"), s=w3546, f=u32 4018019 ("Fill Color")) -> (s? t:f=w3542:u32)
            n1271 = property on="10-14 03" class="Slide (strict)"("Fill Color"=w3542) -> ()  [unwired: 2 in, 2 out]
          }
        }
      }
      frame #15 {
        n1272 = case shown="True" w3613 {
          tunnel: w3605 -> [_ w3645]
          frame False {
          }
          frame True {
            w3640 = enum16{"ID Delete", "Time Delete"}."Time Delete" ("Enum")
            n1273 = property on="projector 03" class="Bool (strict)"() -> ("Value"=w3675:bool)  [unwired: 2 in, 2 out]
            n1274 = Select(t="ON" ("time format string (%c)"), s=w3675, f="OFF" ("time format string (%c)")) -> (s? t:f=w3676:string)
            n1275 = property on="cam 03" class="Bool (strict)"() -> ("Value"=w3673:bool)  [unwired: 2 in, 2 out]
            n1276 = Select(t="ON" ("time format string (%c)"), s=w3673, f="OFF" ("time format string (%c)")) -> (s? t:f=w3674:string)
            n1277 = property on="AUTO/MAN 03" class="Bool (strict)"() -> ("Value"=w3671:bool)  [unwired: 2 in, 2 out]
            n1278 = Select(t="Auto", s=w3671, f="Manual") -> (s? t:f=w3672:string)
            n1279 = property on="DISC 03" class="Bool (strict)"() -> ("Value"=w3669:bool)  [unwired: 2 in, 2 out]
            n1280 = Select(t="Run", s=w3669, f="Stop") -> (s? t:f=w3670:string)
            n1281 = Get Date/Time In Seconds() -> (seconds since 1Jan1904=w3666:timestamp)
            n1282 = Format Date/Time String(time format string (%c)="%Y/%m/%d", seconds (now)=w3666) -> (date/time string=w3667:string)  [unwired: 1 in]
            n1283 = Format Date/Time String(time format string (%c)="%H:%M:%S", seconds (now)=w3666) -> (date/time string=w3668:string)  [unwired: 1 in]
            n1284 = Index Array(array=w3645, index #1=0 ("index")) -> (element #1=w3658:dbl, element #2=w3659:dbl, element #3=w3660:dbl, element #4=w3661:dbl, element #5=w3662:dbl, element #6=w3663:dbl, element #7=w3664:dbl, element #8=w3665:dbl)  [unwired: 7 in]
            n1285 = shared-variable ".\\Setting Lib.lvlib\\database refresh period"() -> (w3644:i32, error out=w3643:errorcluster)  [unwired: 1 in]
            n1286 = Bundle("date/time string"=w3667, "date/time string"=w3668, w3658, w3659, w3660, w3661, w3662, w3663, w3664, w3665, "f"=w3670, "f"=w3672, "time format string (%c)"=w3674, "time format string (%c)"=w3676) -> (w3646:T36)  [unwired: 1 in]
            n1287 = Unbundle(w3646) -> ("date/time string"=w3690:string, "date/time string"=w3689:string, w3688:dbl, w3685:dbl, w3684:dbl, w3687:dbl, "f"=w3682:string, "f"=w3681:string, "time format string (%c)"=w3680:string, "time format string (%c)"=w3679:string)  [unwired: 4 out]
            n1288 = Add(x=w3685, y=w3684) -> (x+y=w3683:dbl)
            n1289 = Compound Arithmetic op=ADD(w3688, w3685, w3684, w3687) -> (w3686:dbl)
            n1290 = To Variant(anything=w3646) -> (Variant=w3691:variant)
            n1291 = call "Database.vi"("Maximum Row"=w3644, "Enum"=w3640, "Delete row?"=TRUE, "Data"=w3691, "Error in"=w3643, "Auto Increment ID?"=TRUE, "Table"="grading_disc_03", "Connection"="dsgs") -> ("Error out"=w3642:errorcluster)  [unwired: 3 in]
            n1292 = Bundle("date/time string"=w3690, "date/time string"=w3689, w3686, w3683, "f"=w3682, "f"=w3681, "time format string (%c)"=w3680, "time format string (%c)"=w3679) -> (w3678:T37)  [unwired: 1 in]
            n1293 = shared-variable ".\\Maintenance.lvlib\\error_36"(w3642) -> ()  [unwired: 1 in, 1 out]
            n1294 = To Variant(anything=w3678) -> (Variant=w3677:variant)
            n1295 = call "Database.vi"("Maximum Row"=w3644, "Enum"=w3640, "Delete row?"=TRUE, "Data"=w3677, "Auto Increment ID?"=TRUE, "Table"="main_grading_group_disc_03", "Connection"="dsgs") -> ("Error out"=w3641:errorcluster)  [unwired: 4 in]
            n1296 = shared-variable ".\\Maintenance.lvlib\\error_37"(w3641) -> ()  [unwired: 1 in, 1 out]
          }
        }
        n1297 = shared-variable ".\\D03.lvlib\\SaveD03"(error in=w3593) -> (w3599:bool, error out=w3596:errorcluster)
        n1298 = Index Array(array=w3594, index (col)=2 ("disabled index (col)")) -> (element=w3602:dbl[])  [unwired: 1 in]
        n1299 = Boolean To (0,1)(Boolean=w3599) -> (0, 1=w3600:i16)
        n1300 = Build Array(w3600) -> (w3601:i16[])
        n1301 = call-poly <vilib>:"Basic Level Trigger Detection.vi"("signal in"=w3601, "level"=0.5, "error in (no error)"=w3596) -> ("trigger detected?"=w3604:bool, "error out"=w3595:errorcluster)  [unwired: 10 in, 1 out]
        n1302 = case shown="True" w3604 {
          selector: w3604 -> [_ w3635]
          tunnel: [FALSE w3635] -> w3603
          tunnel: w3602 -> [_ w3630]
          tunnel: w3595 -> [w3621 w3623]
          tunnel: [w3621 w3622] -> w3592
          frame False {
          }
          frame True {
            n1303 = Array To Spreadsheet String(array=w3630, 3:"%.2f" ("format string")) -> (spreadsheet string=w3634:string)  [unwired: 1 in]
            n1304 = Get Date/Time In Seconds() -> (seconds since 1Jan1904=w3631:timestamp)
            n1305 = Format Date/Time String(time format string (%c)="%H:%M:%S", seconds (now)=w3631) -> (date/time string=w3633:string)  [unwired: 1 in]
            n1306 = Format Date/Time String(time format string (%c)="%Y/%m/%d", seconds (now)=w3631) -> (date/time string=w3632:string)  [unwired: 1 in]
            n1307 = Bundle("date/time string"=w3632, "date/time string"=w3633, "disc 03", "spreadsheet string"=w3634) -> (w3625:T38)  [unwired: 1 in]
            n1308 = To Variant(anything=w3625) -> (Variant=w3624:variant)
            n1309 = call "Database.vi"("Delete row?"=FALSE, "Data"=w3624, "Error in"=w3623, "Auto Increment ID?"=TRUE, "Table"="thresholds_calibration_table", "Connection"="dsgs") -> ("Error out"=w3622:errorcluster)  [unwired: 5 in]
          }
        }
        n1310 = shared-variable ".\\D03.lvlib\\SaveD03Ok"(w3603, error in=w3592) -> ()  [unwired: 1 out]
        n1311 = shared-variable ".\\Maintenance.lvlib\\error_44"(w3592) -> ()  [unwired: 1 in, 1 out]
      }
      frame #16 {
        n1312 = shared-variable ".\\D03.lvlib\\SaveD03"(FALSE ("SaveD28"), error in=w3709) -> (error out=w3708:errorcluster)
        n1313 = case shown="4" "speed disc 28" {
          tunnel: "Error in 18" -> [w3728 w3730 w3746 w3762 w3778]
          tunnel: [w3728 w3729 w3745 w3761 w3777] -> w3711
          frame 0, Default {
          }
          frame 1 {
            n1314 = Get Date/Time In Seconds() -> (seconds since 1Jan1904=w3744:timestamp)
            n1315 = Format Date/Time String(time format string (%c)="%Y/%m/%d", seconds (now)=w3744) -> (date/time string=w3743:string)  [unwired: 1 in]
            n1316 = Format Date/Time String(time format string (%c)="%H:%M:%S", seconds (now)=w3744) -> (date/time string=w3742:string)  [unwired: 1 in]
            n1317 = Bundle("60001", "date/time string"=w3743, "date/time string"=w3742, "Speed signal is changed and applied in disc 28") -> (w3741:T19)  [unwired: 1 in]
            n1318 = To Variant(anything=w3741) -> (Variant=w3740:variant)
            n1319 = call "Database.vi"("Maximum Row"=u64 0 ("Storage Time (Day)"), "Delete row?"=FALSE, "Data"=w3740, "Error in"=w3730, "Auto Increment ID?"=TRUE, "Table"="log_table", "Connection"="dsgs") -> ("Error out"=w3729:errorcluster)  [unwired: 4 in]
          }
          frame 2 {
            n1320 = Get Date/Time In Seconds() -> (seconds since 1Jan1904=w3760:timestamp)
            n1321 = Format Date/Time String(time format string (%c)="%Y/%m/%d", seconds (now)=w3760) -> (date/time string=w3759:string)  [unwired: 1 in]
            n1322 = Format Date/Time String(time format string (%c)="%H:%M:%S", seconds (now)=w3760) -> (date/time string=w3758:string)  [unwired: 1 in]
            n1323 = Bundle("60002", "date/time string"=w3759, "date/time string"=w3758, "Speed signal is changed and applied in disc 28") -> (w3757:T19)  [unwired: 1 in]
            n1324 = To Variant(anything=w3757) -> (Variant=w3756:variant)
            n1325 = call "Database.vi"("Maximum Row"=u64 0 ("Storage Time (Day)"), "Delete row?"=FALSE, "Data"=w3756, "Error in"=w3746, "Auto Increment ID?"=TRUE, "Table"="log_table", "Connection"="dsgs") -> ("Error out"=w3745:errorcluster)  [unwired: 4 in]
          }
          frame 4 {
            n1326 = Get Date/Time In Seconds() -> (seconds since 1Jan1904=w3776:timestamp)
            n1327 = Format Date/Time String(time format string (%c)="%Y/%m/%d", seconds (now)=w3776) -> (date/time string=w3775:string)  [unwired: 1 in]
            n1328 = Format Date/Time String(time format string (%c)="%H:%M:%S", seconds (now)=w3776) -> (date/time string=w3774:string)  [unwired: 1 in]
            n1329 = Bundle("60003", "date/time string"=w3775, "date/time string"=w3774, "Speed signal is changed but not applied in disc 28") -> (w3773:T19)  [unwired: 1 in]
            n1330 = To Variant(anything=w3773) -> (Variant=w3772:variant)
            n1331 = call "Database.vi"("Maximum Row"=u64 0 ("Storage Time (Day)"), "Delete row?"=FALSE, "Data"=w3772, "Error in"=w3762, "Auto Increment ID?"=TRUE, "Table"="log_table", "Connection"="dsgs") -> ("Error out"=w3761:errorcluster)  [unwired: 4 in]
          }
          frame 8 {
            n1332 = Get Date/Time In Seconds() -> (seconds since 1Jan1904=w3792:timestamp)
            n1333 = Format Date/Time String(time format string (%c)="%Y/%m/%d", seconds (now)=w3792) -> (date/time string=w3791:string)  [unwired: 1 in]
            n1334 = Format Date/Time String(time format string (%c)="%H:%M:%S", seconds (now)=w3792) -> (date/time string=w3790:string)  [unwired: 1 in]
            n1335 = Bundle("60004", "date/time string"=w3791, "date/time string"=w3790, "Speed signal is changed but not applied in disc 28") -> (w3789:T19)  [unwired: 1 in]
            n1336 = To Variant(anything=w3789) -> (Variant=w3788:variant)
            n1337 = call "Database.vi"("Maximum Row"=u64 0 ("Storage Time (Day)"), "Delete row?"=FALSE, "Data"=w3788, "Error in"=w3778, "Auto Increment ID?"=TRUE, "Table"="log_table", "Connection"="dsgs") -> ("Error out"=w3777:errorcluster)  [unwired: 4 in]
          }
        }
        n1338 = shared-variable ".\\control setting.lvlib\\bias"() -> (w3701:dbl[])  [unwired: 1 in, 1 out]
        n1339 = Index Array(array=w3701, index=3) -> (element=w3703:dbl)
        n1340 = shared-variable ".\\Maintenance.lvlib\\error_49"(w3711) -> ()  [unwired: 1 in, 1 out]
        n1341 = To Byte Integer(number=w3703) -> (8bit integer=w3700:i8)
      }
      frame #17 {
        n1342 = shared-variable ".\\Setting Lib.lvlib\\processing file path"(error in=w3799) -> (w3795:path, error out=w3805:errorcluster)
        n1343 = shared-variable ".\\D04.lvlib\\LiveViewD04"() -> (w3810:refnum<image>, error out=w3809:errorcluster)  [unwired: 1 in]
        n1344 = shared-variable ".\\D04.lvlib\\GradingThrD04"() -> (w3802:dbl[], error out=w3801:errorcluster)  [unwired: 1 in]
        n1345 = property on="DISC 04" class="Bool (strict)"() -> ("Value"=w3800:bool)  [unwired: 2 in, 2 out]
        n1346 = call "IMAQ Copy"("error in (no error)"=w3809, "Image Dst"=w3811, "Image Src"=w3810) -> ("error out"=w3806:errorcluster, "Image Dst Out"=w3794:T9)  [unwired: 3 in]
        n1347 = call "find and draw circles.vi"("Image Src"=w3794, "module path"=w3795, "function name"="get_circels", "initialized array"=w3823, "Image Dst"=w3818, "error in (no error)"=w3805, "session in"=w3826, "Run/Stop"=w3800, "grading Thr"=w3802, "bias"=w3793) -> ("session out"=w3825:refnum<k35>, "circle info"=w3821:dbl[][], "Image Out"=w3827:T9, "error out"=w3803:errorcluster, "pellet detected?"=w3807:bool)  [unwired: 5 in]
        n1348 = shared-variable ".\\Maintenance.lvlib\\error_20"(w3806) -> ()  [unwired: 1 in, 1 out]
        n1349 = shared-variable ".\\Maintenance.lvlib\\error_25"(w3803) -> ()  [unwired: 1 in, 1 out]
        n1350 = shared-variable ".\\D04.lvlib\\PelletDetectedD04"(w3827, error in=w3801) -> (error out=w3804:errorcluster)
      }
      frame #18 {
        n1351 = shared-variable ".\\Calibration Lib.lvlib\\calibration matrix D04"() -> (w3845:dbl[], error out=w3841:errorcluster)  [unwired: 1 in]
        n1352 = Matrix Size(0:w3838) -> (1:w3836:i32)  [unwired: 1 out]
        n1353 = property on="DISC 04" class="Bool (strict)"() -> ("Value"=w3834:bool)  [unwired: 2 in, 2 out]
        n1354 = shared-variable ".\\Calibration Lib.lvlib\\Method Selection"(error in=w3841) -> (w3846:enum32{"Method 1", "Method 2"}, error out=w3842:errorcluster)
        n1355 = Select(t=w3836, s=w3834, f=0) -> (s? t:f=w3835:i32)
        n1356 = shared-variable ".\\D04.lvlib\\number of pellet 04"(w3835) -> ()  [unwired: 1 in, 1 out]
        n1357 = case shown="\"Method 1\", Default" w3846 {
          tunnel: w3845 -> [_ w3867]
          tunnel: w3838 -> [w3861 w3866]
          tunnel: [w3861 w3864] -> w3844
          tunnel: w3830 -> [w3860 w3865]
          tunnel: [w3860 w3863] -> w3840
          tunnel: w3842 -> [w3859 w3862]
          tunnel: [w3859 w3862] -> w3839
          frame "Method 1", Default {
          }
          frame "Method 2" {
            n1358 = call "pixel2milimetr.vi"("1*3 Transform Matrix"=w3867, "circle array"=w3866, "Error in"=w3865) -> ("calibrated circles"=w3864:dbl[][], "Error out"=w3863:errorcluster)  [unwired: 11 in]
          }
        }
        n1359 = shared-variable ".\\Maintenance.lvlib\\error_30"(w3840, error in=w3839) -> ()  [unwired: 1 out]
      }
      frame #19 {
        n1360 = case shown="True" w3872 {
          tunnel: w3887 -> [_ w3956]
          tunnel: w3886 -> [w3893 w3952]
          tunnel: [w3893 w3951] -> w3885
          tunnel: w3884 -> [w3892 w3947]
          tunnel: [w3892 w3946] -> w3883
          tunnel: w3882 -> [w3894 w3942]
          tunnel: [w3894 w3941] -> w3881
          tunnel: [dbl[] [0.0, 0.0, 0.0, 0.0, 0.0, 0.0, 0.0, 0.0] w3907] -> w3873
          tunnel: [errorcluster {"status"=FALSE, "code"=0, "source"=""} ("error IO") w3926] -> w3871
          frame False {
          }
          frame True {
            w3898 = dbl[] [250.047, 512.0, 857.375, 1331.0, 2048.0, 2744.0, 4096.0]  # fixed threshoulds
            n1361 = shared-variable ".\\Calibration Lib.lvlib\\Method Selection"() -> (w3932:enum32{"Method 1", "Method 2"}, error out=w3929:errorcluster)  [unwired: 1 in]
            n1362 = Index Array(array=w3956, index (col)=2 ("disabled index (col)")) -> (element=w3944:dbl[])  [unwired: 1 in]
            n1363 = property on="avg grading array size" class="DigNum (strict)"() -> ("Value"=w3935:i32)  [unwired: 2 in, 2 out]
            n1364 = property on="live grading array size" class="DigNum (strict)"() -> ("Value"=w3936:i32)  [unwired: 2 in, 2 out]
            n1365 = Array Size(array=w3944) -> (size(s)=w3945:i32)
            n1366 = shared-variable ".\\D04.lvlib\\GradingThrD04"(error in=w3929) -> (w3930:dbl[], error out=w3928:errorcluster)
            n1367 = Subtract(x=w3936, y=w3945) -> (x-y=w3954:i32)
            n1368 = Subtract(x=w3935, y=w3945) -> (x-y=w3948:i32)
            n1369 = Multiply(x=w3898, y=0.125) -> (x*y=w3897:dbl[])
            n1370 = Equal?(x=w3932, y=enum32{"Method 1", "Method 2"}."Method 1" ("Method Selection")) -> (x = y?=w3933:bool)
            n1371 = call "array managment.vi"("2D array in"=w3952, "col sel"=3, "cir num"=w3945, "index"=w3954, "subarray"=w3944) -> ("2D array out"=w3951:dbl[][], "1D array out"=w3953:dbl[])  [unwired: 13 in]
            n1372 = call "array managment.vi"("2D array in"=w3947, "col sel"=3, "cir num"=w3945, "index"=w3948, "subarray"=w3944) -> ("2D array out"=w3946:dbl[][], "1D array out"=w3950:dbl[])  [unwired: 13 in]
            n1373 = property on="DISC 04" class="Bool (strict)"() -> ("Value"=w3922:bool)  [unwired: 2 in, 2 out]
            n1374 = Select(t=w3930, s=w3933, f=w3897) -> (s? t:f=w3931:dbl[])
            n1375 = property on="DISC 04" class="Bool (strict)"() -> ("Value"=w3921:bool)  [unwired: 2 in, 2 out]
            n1376 = call "pelletpercents.vi"("Run/Stop"=w3922, "grading threshoulds"=w3931, "Sorted data"=w3953) -> ("Percentage"=w3937:dbl[])  [unwired: 8 in]
            n1377 = call "pelletpercents.vi"("Run/Stop"=w3921, "grading threshoulds"=w3931, "Sorted data"=w3950) -> ("Percentage"=w3923:dbl[])  [unwired: 8 in]
            n1378 = Number To Fractional String(number=w3937, precision (6)=i16 2) -> (F-format string=w3938:string[])  [unwired: 2 in]
            n1379 = Number To Fractional String(number=w3923, precision (6)=i16 2) -> (F-format string=w3925:string[])  [unwired: 2 in]
            n1380 = Fract/Exp String To Number(string=w3938) -> (number=w3907:dbl[])  [unwired: 3 in, 1 out]
            n1381 = property on="DISC 04" class="Bool (strict)"() -> ("Value"=w3903:bool)  [unwired: 2 in, 2 out]
            n1382 = Fract/Exp String To Number(string=w3925) -> (number=w3896:dbl[])  [unwired: 3 in, 1 out]
            n1383 = call "grading average.vi"("input array"=w3896) -> ("avg"=w3904:dbl)  [unwired: 10 in]
            "AVG 04" <- w3904
            n1384 = Not A Number/Path/Refnum?(number/path/refnum=w3904) -> (NaN/Path/Refnum?=w3901:bool)
            n1385 = shared-variable ".\\D04.lvlib\\AvgResultD04"(w3896, error in=w3928) -> (error out=w3927:errorcluster)
            n1386 = Index Array(array=w3907, index #1=3 ("index")) -> (element #1=w3920:dbl, element #2=w3917:dbl, element #3=w3918:dbl, element #4=w3919:dbl)  [unwired: 3 in]
            n1387 = Not(x=w3901) -> (.not. x?=w3900:bool)
            n1388 = And(x=w3903, y=w3900) -> (x .and. y?=w3902:bool)
            n1389 = Add(x=w3920, y=w3917) -> (x+y=w3909:dbl)
            "9.5-12.7 04" <- w3909
            n1390 = Add(x=w3918, y=w3919) -> (x+y=w3910:dbl)
            "12.7-16 04" <- w3910
            n1391 = Add(x=w3917, y=w3918) -> (x+y=w3912:dbl)
            "10-14 04" <- w3912
            n1392 = Select(t=w3904, s=w3902, f=12.0) -> (s? t:f=w3905:dbl)
            n1393 = shared-variable ".\\D04.lvlib\\LiveResultD04"(w3907, error in=w3927) -> (error out=w3926:errorcluster)
            n1394 = Add(x=w3910, y=w3909) -> (x+y=→"8-16mm 04":dbl)
            n1395 = call "dif array management.vi"("2D array in"=w3942, "col sel"=3, "new element/subarray"=w3905) -> ("2D array out"=w3941:dbl[][])  [unwired: 15 in, 1 out]
            n1396 = Greater Or Equal?(x=w3912, y=70.0) -> (x >= y?=w3915:bool)
            n1397 = Select(t=u32 65282 ("Fill Color"), s=w3915, f=u32 4018019 ("Fill Color")) -> (s? t:f=w3911:u32)
            n1398 = property on="10-14 04" class="Slide (strict)"("Fill Color"=w3911) -> ()  [unwired: 2 in, 2 out]
          }
        }
      }
      frame #20 {
        n1399 = case shown="True" w3982 {
          tunnel: w3975 -> [_ w4013]
          frame False {
          }
          frame True {
            w4008 = enum16{"ID Delete", "Time Delete"}."Time Delete" ("Enum")
            n1400 = property on="projector 04" class="Bool (strict)"() -> ("Value"=w4043:bool)  [unwired: 2 in, 2 out]
            n1401 = Select(t="ON" ("time format string (%c)"), s=w4043, f="OFF" ("time format string (%c)")) -> (s? t:f=w4044:string)
            n1402 = property on="cam 04" class="Bool (strict)"() -> ("Value"=w4041:bool)  [unwired: 2 in, 2 out]
            n1403 = Select(t="ON" ("time format string (%c)"), s=w4041, f="OFF" ("time format string (%c)")) -> (s? t:f=w4042:string)
            n1404 = property on="AUTO/MAN 04" class="Bool (strict)"() -> ("Value"=w4039:bool)  [unwired: 2 in, 2 out]
            n1405 = Select(t="Auto", s=w4039, f="Manual") -> (s? t:f=w4040:string)
            n1406 = property on="DISC 04" class="Bool (strict)"() -> ("Value"=w4037:bool)  [unwired: 2 in, 2 out]
            n1407 = Select(t="Run", s=w4037, f="Stop") -> (s? t:f=w4038:string)
            n1408 = Get Date/Time In Seconds() -> (seconds since 1Jan1904=w4034:timestamp)
            n1409 = Format Date/Time String(time format string (%c)="%Y/%m/%d", seconds (now)=w4034) -> (date/time string=w4035:string)  [unwired: 1 in]
            n1410 = Format Date/Time String(time format string (%c)="%H:%M:%S", seconds (now)=w4034) -> (date/time string=w4036:string)  [unwired: 1 in]
            n1411 = Index Array(array=w4013, index #1=0 ("index")) -> (element #1=w4026:dbl, element #2=w4027:dbl, element #3=w4028:dbl, element #4=w4029:dbl, element #5=w4030:dbl, element #6=w4031:dbl, element #7=w4032:dbl, element #8=w4033:dbl)  [unwired: 7 in]
            n1412 = Bundle("date/time string"=w4035, "date/time string"=w4036, w4026, w4027, w4028, w4029, w4030, w4031, w4032, w4033, "f"=w4038, "f"=w4040, "time format string (%c)"=w4042, "time format string (%c)"=w4044) -> (w4014:T36)  [unwired: 1 in]
            n1413 = shared-variable ".\\Setting Lib.lvlib\\database refresh period"() -> (w4012:i32, error out=w4011:errorcluster)  [unwired: 1 in]
            n1414 = Unbundle(w4014) -> ("date/time string"=w4058:string, "date/time string"=w4057:string, w4056:dbl, w4053:dbl, w4052:dbl, w4055:dbl, "f"=w4050:string, "f"=w4049:string, "time format string (%c)"=w4048:string, "time format string (%c)"=w4047:string)  [unwired: 4 out]
            n1415 = Add(x=w4053, y=w4052) -> (x+y=w4051:dbl)
            n1416 = Compound Arithmetic op=ADD(w4056, w4053, w4052, w4055) -> (w4054:dbl)
            n1417 = To Variant(anything=w4014) -> (Variant=w4059:variant)
            n1418 = call "Database.vi"("Maximum Row"=w4012, "Enum"=w4008, "Delete row?"=TRUE, "Data"=w4059, "Error in"=w4011, "Auto Increment ID?"=TRUE, "Table"="grading_disc_04", "Connection"="dsgs") -> ("Error out"=w4010:errorcluster)  [unwired: 3 in]
            n1419 = Bundle("date/time string"=w4058, "date/time string"=w4057, w4054, w4051, "f"=w4050, "f"=w4049, "time format string (%c)"=w4048, "time format string (%c)"=w4047) -> (w4046:T37)  [unwired: 1 in]
            n1420 = shared-variable ".\\Maintenance.lvlib\\error_38"(w4010) -> ()  [unwired: 1 in, 1 out]
            n1421 = To Variant(anything=w4046) -> (Variant=w4045:variant)
            n1422 = call "Database.vi"("Maximum Row"=w4012, "Enum"=w4008, "Delete row?"=TRUE, "Data"=w4045, "Auto Increment ID?"=TRUE, "Table"="main_grading_group_disc_04", "Connection"="dsgs") -> ("Error out"=w4009:errorcluster)  [unwired: 4 in]
            n1423 = shared-variable ".\\Maintenance.lvlib\\error_39"(w4009) -> ()  [unwired: 1 in, 1 out]
          }
        }
        n1424 = shared-variable ".\\D04.lvlib\\SaveD04"(error in=w3963) -> (w3969:bool, error out=w3966:errorcluster)
        n1425 = Index Array(array=w3964, index (col)=3 ("disabled index (col)")) -> (element=w3972:dbl[])  [unwired: 1 in]
        n1426 = Boolean To (0,1)(Boolean=w3969) -> (0, 1=w3970:i16)
        n1427 = Build Array(w3970) -> (w3971:i16[])
        n1428 = call-poly <vilib>:"Basic Level Trigger Detection.vi"("signal in"=w3971, "level"=0.5, "error in (no error)"=w3966) -> ("trigger detected?"=w3974:bool, "error out"=w3965:errorcluster)  [unwired: 10 in, 1 out]
        n1429 = case shown="True" w3974 {
          selector: w3974 -> [_ w4003]
          tunnel: [FALSE w4003] -> w3973
          tunnel: w3972 -> [_ w3998]
          tunnel: w3965 -> [w3989 w3991]
          tunnel: [w3989 w3990] -> w3961
          frame False {
          }
          frame True {
            n1430 = Array To Spreadsheet String(array=w3998, 3:"%.2f" ("format string")) -> (spreadsheet string=w4002:string)  [unwired: 1 in]
            n1431 = Get Date/Time In Seconds() -> (seconds since 1Jan1904=w3999:timestamp)
            n1432 = Format Date/Time String(time format string (%c)="%H:%M:%S", seconds (now)=w3999) -> (date/time string=w4001:string)  [unwired: 1 in]
            n1433 = Format Date/Time String(time format string (%c)="%Y/%m/%d", seconds (now)=w3999) -> (date/time string=w4000:string)  [unwired: 1 in]
            n1434 = Bundle("date/time string"=w4000, "date/time string"=w4001, "disc 04", "spreadsheet string"=w4002) -> (w3993:T38)  [unwired: 1 in]
            n1435 = To Variant(anything=w3993) -> (Variant=w3992:variant)
            n1436 = call "Database.vi"("Delete row?"=FALSE, "Data"=w3992, "Error in"=w3991, "Auto Increment ID?"=TRUE, "Table"="thresholds_calibration_table", "Connection"="dsgs") -> ("Error out"=w3990:errorcluster)  [unwired: 5 in]
          }
        }
        n1437 = shared-variable ".\\D04.lvlib\\SaveD04Ok"(w3973) -> (error out=w3962:errorcluster)  [unwired: 1 in]
        n1438 = shared-variable ".\\Maintenance.lvlib\\error_45"(w3961) -> ()  [unwired: 1 in, 1 out]
      }
      frame #21 {
        n1439 = shared-variable ".\\D04.lvlib\\SaveD04"(FALSE ("SaveD29"), error in=w4075) -> (error out=w4074:errorcluster)
        n1440 = case shown="4" "speed disc 29" {
          tunnel: w4074 -> [w4091 w4093 w4109 w4125 w4141]
          tunnel: [w4091 w4092 w4108 w4124 w4140] -> w4077
          frame 0, Default {
          }
          frame 1 {
            n1441 = Get Date/Time In Seconds() -> (seconds since 1Jan1904=w4107:timestamp)
            n1442 = Format Date/Time String(time format string (%c)="%Y/%m/%d", seconds (now)=w4107) -> (date/time string=w4106:string)  [unwired: 1 in]
            n1443 = Format Date/Time String(time format string (%c)="%H:%M:%S", seconds (now)=w4107) -> (date/time string=w4105:string)  [unwired: 1 in]
            n1444 = Bundle("60001", "date/time string"=w4106, "date/time string"=w4105, "Speed signal is changed and applied in disc 29") -> (w4104:T19)  [unwired: 1 in]
            n1445 = To Variant(anything=w4104) -> (Variant=w4103:variant)
            n1446 = call "Database.vi"("Maximum Row"=u64 0 ("Storage Time (Day)"), "Delete row?"=FALSE, "Data"=w4103, "Error in"=w4093, "Auto Increment ID?"=TRUE, "Table"="log_table", "Connection"="dsgs") -> ("Error out"=w4092:errorcluster)  [unwired: 4 in]
          }
          frame 2 {
            n1447 = Get Date/Time In Seconds() -> (seconds since 1Jan1904=w4123:timestamp)
            n1448 = Format Date/Time String(time format string (%c)="%Y/%m/%d", seconds (now)=w4123) -> (date/time string=w4122:string)  [unwired: 1 in]
            n1449 = Format Date/Time String(time format string (%c)="%H:%M:%S", seconds (now)=w4123) -> (date/time string=w4121:string)  [unwired: 1 in]
            n1450 = Bundle("60002", "date/time string"=w4122, "date/time string"=w4121, "Speed signal is changed and applied in disc 29") -> (w4120:T19)  [unwired: 1 in]
            n1451 = To Variant(anything=w4120) -> (Variant=w4119:variant)
            n1452 = call "Database.vi"("Maximum Row"=u64 0 ("Storage Time (Day)"), "Delete row?"=FALSE, "Data"=w4119, "Error in"=w4109, "Auto Increment ID?"=TRUE, "Table"="log_table", "Connection"="dsgs") -> ("Error out"=w4108:errorcluster)  [unwired: 4 in]
          }
          frame 4 {
            n1453 = Get Date/Time In Seconds() -> (seconds since 1Jan1904=w4139:timestamp)
            n1454 = Format Date/Time String(time format string (%c)="%Y/%m/%d", seconds (now)=w4139) -> (date/time string=w4138:string)  [unwired: 1 in]
            n1455 = Format Date/Time String(time format string (%c)="%H:%M:%S", seconds (now)=w4139) -> (date/time string=w4137:string)  [unwired: 1 in]
            n1456 = Bundle("60003", "date/time string"=w4138, "date/time string"=w4137, "Speed signal is changed but not applied in disc 29") -> (w4136:T19)  [unwired: 1 in]
            n1457 = To Variant(anything=w4136) -> (Variant=w4135:variant)
            n1458 = call "Database.vi"("Maximum Row"=u64 0 ("Storage Time (Day)"), "Delete row?"=FALSE, "Data"=w4135, "Error in"=w4125, "Auto Increment ID?"=TRUE, "Table"="log_table", "Connection"="dsgs") -> ("Error out"=w4124:errorcluster)  [unwired: 4 in]
          }
          frame 8 {
            n1459 = Get Date/Time In Seconds() -> (seconds since 1Jan1904=w4155:timestamp)
            n1460 = Format Date/Time String(time format string (%c)="%Y/%m/%d", seconds (now)=w4155) -> (date/time string=w4154:string)  [unwired: 1 in]
            n1461 = Format Date/Time String(time format string (%c)="%H:%M:%S", seconds (now)=w4155) -> (date/time string=w4153:string)  [unwired: 1 in]
            n1462 = Bundle("60004", "date/time string"=w4154, "date/time string"=w4153, "Speed signal is changed but not applied in disc 29") -> (w4152:T19)  [unwired: 1 in]
            n1463 = To Variant(anything=w4152) -> (Variant=w4151:variant)
            n1464 = call "Database.vi"("Maximum Row"=u64 0 ("Storage Time (Day)"), "Delete row?"=FALSE, "Data"=w4151, "Error in"=w4141, "Auto Increment ID?"=TRUE, "Table"="log_table", "Connection"="dsgs") -> ("Error out"=w4140:errorcluster)  [unwired: 4 in]
          }
        }
        n1465 = shared-variable ".\\Setting Lib.lvlib\\processing file path"() -> (w4069:path, error out=w4070:errorcluster)  [unwired: 1 in]
        n1466 = shared-variable ".\\Maintenance.lvlib\\error_50"(w4077) -> ()  [unwired: 1 in, 1 out]
      }
      frame #22 {
        n1467 = shared-variable ".\\D05.lvlib\\LiveViewD05"() -> (w4175:refnum<image>, error out=w4174:errorcluster)  [unwired: 1 in]
        n1468 = shared-variable ".\\control setting.lvlib\\bias"() -> (w4157:dbl[])  [unwired: 1 in, 1 out]
        n1469 = Index Array(array=w4157, index=4) -> (element=w4159:dbl)
        n1470 = shared-variable ".\\D05.lvlib\\GradingThrD05"() -> (w4169:dbl[], error out=w4168:errorcluster)  [unwired: 1 in]
        n1471 = call "IMAQ Copy"("error in (no error)"=w4174, "Image Dst"=w4176, "Image Src"=w4175) -> ("error out"=w4172:errorcluster, "Image Dst Out"=w4160:T9)  [unwired: 3 in]
        n1472 = To Byte Integer(number=w4159) -> (8bit integer=w4156:i8)
        n1473 = property on="DISC 05" class="Bool (strict)"() -> ("Value"=w4167:bool)  [unwired: 2 in, 2 out]
        n1474 = call "find and draw circles.vi"("Image Src"=w4160, "module path"=w4161, "function name"="get_circels", "initialized array"=w4164, "Image Dst"=w4183, "error in (no error)"=w4162, "session in"=w4189, "Run/Stop"=w4167, "grading Thr"=w4169, "bias"=w4156) -> ("session out"=w4188:refnum<k35>, "circle info"=w4186:dbl[][], "Image Out"=w4191:T9, "error out"=w4170:errorcluster, "pellet detected?"=w4173:bool)  [unwired: 5 in]
        n1475 = shared-variable ".\\Maintenance.lvlib\\error_21"(w4172) -> ()  [unwired: 1 in, 1 out]
        n1476 = shared-variable ".\\Maintenance.lvlib\\error_26"(w4170) -> ()  [unwired: 1 in, 1 out]
        n1477 = shared-variable ".\\D05.lvlib\\PelletDetectedD05"(w4191, error in=w4168) -> (error out=w4171:errorcluster)
      }
      frame #23 {
        n1478 = shared-variable ".\\Calibration Lib.lvlib\\calibration matrix D05"() -> (w4209:dbl[], error out=w4206:errorcluster)  [unwired: 1 in]
        n1479 = Matrix Size(0:w4202) -> (1:w4201:i32)  [unwired: 1 out]
        n1480 = property on="DISC 05" class="Bool (strict)"() -> ("Value"=w4199:bool)  [unwired: 2 in, 2 out]
        n1481 = Select(t=w4201, s=w4199, f=0) -> (s? t:f=w4200:i32)
        n1482 = shared-variable ".\\Calibration Lib.lvlib\\Method Selection"(error in=w4206) -> (w4210:enum32{"Method 1", "Method 2"}, error out=w4205:errorcluster)
        n1483 = shared-variable ".\\D05.lvlib\\number of pellet 05"(w4200) -> ()  [unwired: 1 in, 1 out]
        n1484 = case shown="\"Method 1\", Default" w4210 {
          tunnel: w4209 -> [_ w4228]
          tunnel: w4202 -> [w4222 w4227]
          tunnel: [w4222 w4225] -> w4208
          tunnel: w4193 -> [w4221 w4226]
          tunnel: [w4221 w4224] -> w4204
          tunnel: w4205 -> [w4220 w4223]
          tunnel: [w4220 w4223] -> w4203
          frame "Method 1", Default {
          }
          frame "Method 2" {
            n1485 = call "pixel2milimetr.vi"("1*3 Transform Matrix"=w4228, "circle array"=w4227, "Error in"=w4226) -> ("calibrated circles"=w4225:dbl[][], "Error out"=w4224:errorcluster)  [unwired: 11 in]
          }
        }
        n1486 = shared-variable ".\\Maintenance.lvlib\\error_31"(w4204, error in=w4203) -> ()  [unwired: 1 out]
      }
      frame #24 {
        n1487 = case shown="True" w4234 {
          tunnel: w4248 -> [_ w4316]
          tunnel: w4247 -> [w4253 w4311]
          tunnel: [w4253 w4310] -> w4246
          tunnel: w4245 -> [w4254 w4306]
          tunnel: [w4254 w4304] -> w4244
          tunnel: w4243 -> [w4252 w4301]
          tunnel: [w4252 w4300] -> w4242
          tunnel: [dbl[] [0.0, 0.0, 0.0, 0.0, 0.0, 0.0, 0.0, 0.0] w4264] -> w4235
          tunnel: [errorcluster {"status"=FALSE, "code"=0, "source"=""} ("error IO") w4285] -> w4233
          frame False {
          }
          frame True {
            w4256 = dbl[] [250.047, 512.0, 857.375, 1331.0, 2048.0, 2744.0, 4096.0]  # fixed threshoulds
            n1488 = shared-variable ".\\D05.lvlib\\GradingThrD05"() -> (w4290:dbl[], error out=w4287:errorcluster)  [unwired: 1 in]
            n1489 = Index Array(array=w4316, index (col)=2 ("disabled index (col)")) -> (element=w4303:dbl[])  [unwired: 1 in]
            n1490 = property on="avg grading array size" class="DigNum (strict)"() -> ("Value"=w4294:i32)  [unwired: 2 in, 2 out]
            n1491 = shared-variable ".\\Calibration Lib.lvlib\\Method Selection"(error in=w4287) -> (w4291:enum32{"Method 1", "Method 2"}, error out=w4286:errorcluster)
            n1492 = property on="live grading array size" class="DigNum (strict)"() -> ("Value"=w4295:i32)  [unwired: 2 in, 2 out]
            n1493 = Array Size(array=w4303) -> (size(s)=w4305:i32)
            n1494 = Subtract(x=w4295, y=w4305) -> (x-y=w4314:i32)
            n1495 = Subtract(x=w4294, y=w4305) -> (x-y=w4309:i32)
            n1496 = Multiply(x=w4256, y=0.125) -> (x*y=w4283:dbl[])
            n1497 = Equal?(x=w4291, y=enum32{"Method 1", "Method 2"}."Method 1" ("Method Selection")) -> (x = y?=w4292:bool)
            n1498 = call "array managment.vi"("2D array in"=w4311, "col sel"=4, "cir num"=w4305, "index"=w4314, "subarray"=w4303) -> ("2D array out"=w4310:dbl[][], "1D array out"=w4312:dbl[])  [unwired: 13 in]
            n1499 = call "array managment.vi"("2D array in"=w4306, "col sel"=4, "cir num"=w4305, "index"=w4309, "subarray"=w4303) -> ("2D array out"=w4304:dbl[][], "1D array out"=w4307:dbl[])  [unwired: 13 in]
            n1500 = Select(t=w4290, s=w4292, f=w4283) -> (s? t:f=w4289:dbl[])
            n1501 = property on="DISC 05" class="Bool (strict)"() -> ("Value"=w4279:bool)  [unwired: 2 in, 2 out]
            n1502 = property on="DISC 05" class="Bool (strict)"() -> ("Value"=w4278:bool)  [unwired: 2 in, 2 out]
            n1503 = call "pelletpercents.vi"("Run/Stop"=w4279, "grading threshoulds"=w4289, "Sorted data"=w4312) -> ("Percentage"=w4296:dbl[])  [unwired: 8 in]
            n1504 = call "pelletpercents.vi"("Run/Stop"=w4278, "grading threshoulds"=w4289, "Sorted data"=w4307) -> ("Percentage"=w4280:dbl[])  [unwired: 8 in]
            n1505 = Number To Fractional String(number=w4296, precision (6)=i16 2) -> (F-format string=w4297:string[])  [unwired: 2 in]
            n1506 = Number To Fractional String(number=w4280, precision (6)=i16 2) -> (F-format string=w4282:string[])  [unwired: 2 in]
            n1507 = Fract/Exp String To Number(string=w4297) -> (number=w4264:dbl[])  [unwired: 3 in, 1 out]
            n1508 = property on="DISC 05" class="Bool (strict)"() -> ("Value"=w4261:bool)  [unwired: 2 in, 2 out]
            n1509 = Fract/Exp String To Number(string=w4282) -> (number=w4255:dbl[])  [unwired: 3 in, 1 out]
            n1510 = call "grading average.vi"("input array"=w4255) -> ("avg"=w4260:dbl)  [unwired: 10 in]
            "AVG 05" <- w4260
            n1511 = shared-variable ".\\D05.lvlib\\AvgResultD05"(w4255, error in=w4286) -> (error out=w4288:errorcluster)
            n1512 = Not A Number/Path/Refnum?(number/path/refnum=w4260) -> (NaN/Path/Refnum?=w4258:bool)
            n1513 = Not(x=w4258) -> (.not. x?=w4257:bool)
            n1514 = Index Array(array=w4264, index #1=3 ("index")) -> (element #1=w4277:dbl, element #2=w4274:dbl, element #3=w4275:dbl, element #4=w4276:dbl)  [unwired: 3 in]
            n1515 = And(x=w4261, y=w4257) -> (x .and. y?=w4259:bool)
            n1516 = Add(x=w4277, y=w4274) -> (x+y=w4266:dbl)
            "9.5-12.7 05" <- w4266
            n1517 = Add(x=w4275, y=w4276) -> (x+y=w4267:dbl)
            "12.7-16 05" <- w4267
            n1518 = Add(x=w4274, y=w4275) -> (x+y=w4269:dbl)
            "10-14 05" <- w4269
            n1519 = shared-variable ".\\D05.lvlib\\LiveResultD05"(w4264, error in=w4288) -> (error out=w4285:errorcluster)
            n1520 = Add(x=w4267, y=w4266) -> (x+y=→"8-16mm 05":dbl)
            n1521 = Select(t=w4260, s=w4259, f=12.0) -> (s? t:f=w4262:dbl)
            n1522 = call "dif array management.vi"("2D array in"=w4301, "col sel"=4, "new element/subarray"=w4262) -> ("2D array out"=w4300:dbl[][])  [unwired: 15 in, 1 out]
            n1523 = Greater Or Equal?(x=w4269, y=70.0) -> (x >= y?=w4272:bool)
            n1524 = Select(t=u32 65282 ("Fill Color"), s=w4272, f=u32 4018019 ("Fill Color")) -> (s? t:f=w4268:u32)
            n1525 = property on="10-14 05" class="Slide (strict)"("Fill Color"=w4268) -> ()  [unwired: 2 in, 2 out]
          }
        }
      }
      frame #25 {
        n1526 = case shown="True" w4317 {
          tunnel: w4336 -> [_ w4370]
          frame False {
          }
          frame True {
            w4365 = enum16{"ID Delete", "Time Delete"}."Time Delete" ("Enum")
            n1527 = property on="projector 05" class="Bool (strict)"() -> ("Value"=w4400:bool)  [unwired: 2 in, 2 out]
            n1528 = Select(t="ON" ("time format string (%c)"), s=w4400, f="OFF" ("time format string (%c)")) -> (s? t:f=w4401:string)
            n1529 = property on="cam 05" class="Bool (strict)"() -> ("Value"=w4398:bool)  [unwired: 2 in, 2 out]
            n1530 = Select(t="ON" ("time format string (%c)"), s=w4398, f="OFF" ("time format string (%c)")) -> (s? t:f=w4399:string)
            n1531 = property on="AUTO/MAN 05" class="Bool (strict)"() -> ("Value"=w4396:bool)  [unwired: 2 in, 2 out]
            n1532 = Select(t="Auto", s=w4396, f="Manual") -> (s? t:f=w4397:string)
            n1533 = property on="DISC 05" class="Bool (strict)"() -> ("Value"=w4394:bool)  [unwired: 2 in, 2 out]
            n1534 = Select(t="Run", s=w4394, f="Stop") -> (s? t:f=w4395:string)
            n1535 = Get Date/Time In Seconds() -> (seconds since 1Jan1904=w4391:timestamp)
            n1536 = Format Date/Time String(time format string (%c)="%Y/%m/%d", seconds (now)=w4391) -> (date/time string=w4392:string)  [unwired: 1 in]
            n1537 = Format Date/Time String(time format string (%c)="%H:%M:%S", seconds (now)=w4391) -> (date/time string=w4393:string)  [unwired: 1 in]
            n1538 = Index Array(array=w4370, index #1=0 ("index")) -> (element #1=w4383:dbl, element #2=w4384:dbl, element #3=w4385:dbl, element #4=w4386:dbl, element #5=w4387:dbl, element #6=w4388:dbl, element #7=w4389:dbl, element #8=w4390:dbl)  [unwired: 7 in]
            n1539 = Bundle("date/time string"=w4392, "date/time string"=w4393, w4383, w4384, w4385, w4386, w4387, w4388, w4389, w4390, "f"=w4395, "f"=w4397, "time format string (%c)"=w4399, "time format string (%c)"=w4401) -> (w4371:T36)  [unwired: 1 in]
            n1540 = shared-variable ".\\Setting Lib.lvlib\\database refresh period"() -> (w4369:i32, error out=w4368:errorcluster)  [unwired: 1 in]
            n1541 = Unbundle(w4371) -> ("date/time string"=w4415:string, "date/time string"=w4414:string, w4413:dbl, w4410:dbl, w4409:dbl, w4412:dbl, "f"=w4407:string, "f"=w4406:string, "time format string (%c)"=w4405:string, "time format string (%c)"=w4404:string)  [unwired: 4 out]
            n1542 = Add(x=w4410, y=w4409) -> (x+y=w4408:dbl)
            n1543 = Compound Arithmetic op=ADD(w4413, w4410, w4409, w4412) -> (w4411:dbl)
            n1544 = To Variant(anything=w4371) -> (Variant=w4416:variant)
            n1545 = call "Database.vi"("Maximum Row"=w4369, "Enum"=w4365, "Delete row?"=TRUE, "Data"=w4416, "Error in"=w4368, "Auto Increment ID?"=TRUE, "Table"="grading_disc_05", "Connection"="dsgs") -> ("Error out"=w4366:errorcluster)  [unwired: 3 in]
            n1546 = Bundle("date/time string"=w4415, "date/time string"=w4414, w4411, w4408, "f"=w4407, "f"=w4406, "time format string (%c)"=w4405, "time format string (%c)"=w4404) -> (w4403:T37)  [unwired: 1 in]
            n1547 = shared-variable ".\\Maintenance.lvlib\\error_40"(w4366) -> ()  [unwired: 1 in, 1 out]
            n1548 = To Variant(anything=w4403) -> (Variant=w4402:variant)
            n1549 = call "Database.vi"("Maximum Row"=w4369, "Enum"=w4365, "Delete row?"=TRUE, "Data"=w4402, "Auto Increment ID?"=TRUE, "Table"="main_grading_group_disc_05", "Connection"="dsgs") -> ("Error out"=w4367:errorcluster)  [unwired: 4 in]
            n1550 = shared-variable ".\\Maintenance.lvlib\\error_41"(w4367) -> ()  [unwired: 1 in, 1 out]
          }
        }
        n1551 = shared-variable ".\\D05.lvlib\\SaveD05"(error in=w4324) -> (w4330:bool, error out=w4327:errorcluster)
        n1552 = Index Array(array=w4325, index (col)=4 ("disabled index (col)")) -> (element=w4333:dbl[])  [unwired: 1 in]
        n1553 = Boolean To (0,1)(Boolean=w4330) -> (0, 1=w4331:i16)
        n1554 = Build Array(w4331) -> (w4332:i16[])
        n1555 = call-poly <vilib>:"Basic Level Trigger Detection.vi"("signal in"=w4332, "level"=0.5, "error in (no error)"=w4327) -> ("trigger detected?"=w4335:bool, "error out"=w4326:errorcluster)  [unwired: 10 in, 1 out]
        n1556 = case shown="True" w4335 {
          selector: w4335 -> [_ w4360]
          tunnel: [FALSE w4360] -> w4334
          tunnel: w4333 -> [_ w4355]
          tunnel: w4326 -> [w4346 w4348]
          tunnel: [w4346 w4347] -> w4322
          frame False {
          }
          frame True {
            n1557 = Array To Spreadsheet String(array=w4355, 3:"%.2f" ("format string")) -> (spreadsheet string=w4359:string)  [unwired: 1 in]
            n1558 = Get Date/Time In Seconds() -> (seconds since 1Jan1904=w4356:timestamp)
            n1559 = Format Date/Time String(time format string (%c)="%H:%M:%S", seconds (now)=w4356) -> (date/time string=w4358:string)  [unwired: 1 in]
            n1560 = Format Date/Time String(time format string (%c)="%Y/%m/%d", seconds (now)=w4356) -> (date/time string=w4357:string)  [unwired: 1 in]
            n1561 = Bundle("date/time string"=w4357, "date/time string"=w4358, "disc 05", "spreadsheet string"=w4359) -> (w4350:T38)  [unwired: 1 in]
            n1562 = To Variant(anything=w4350) -> (Variant=w4349:variant)
            n1563 = call "Database.vi"("Delete row?"=FALSE, "Data"=w4349, "Error in"=w4348, "Auto Increment ID?"=TRUE, "Table"="thresholds_calibration_table", "Connection"="dsgs") -> ("Error out"=w4347:errorcluster)  [unwired: 5 in]
          }
        }
        n1564 = shared-variable ".\\D05.lvlib\\SaveD05Ok"(w4334, error in=w4322) -> (error out=w4323:errorcluster)
        n1565 = shared-variable ".\\Maintenance.lvlib\\error_46"(w4322) -> ()  [unwired: 1 in, 1 out]
      }
      frame #26 {
        n1566 = shared-variable ".\\D05.lvlib\\SaveD05"(FALSE ("SaveD30"), error in=w4433) -> (error out=w4432:errorcluster)
        n1567 = case shown="4" "speed disc 30" {
          tunnel: w4432 -> [w4446 w4448 w4464 w4480 w4496]
          tunnel: [w4446 w4447 w4463 w4479 w4495] -> w4435
          frame 0, Default {
          }
          frame 1 {
            n1568 = Get Date/Time In Seconds() -> (seconds since 1Jan1904=w4462:timestamp)
            n1569 = Format Date/Time String(time format string (%c)="%Y/%m/%d", seconds (now)=w4462) -> (date/time string=w4461:string)  [unwired: 1 in]
            n1570 = Format Date/Time String(time format string (%c)="%H:%M:%S", seconds (now)=w4462) -> (date/time string=w4460:string)  [unwired: 1 in]
            n1571 = Bundle("60001", "date/time string"=w4461, "date/time string"=w4460, "Speed signal is changed and applied in disc 30") -> (w4459:T19)  [unwired: 1 in]
            n1572 = To Variant(anything=w4459) -> (Variant=w4458:variant)
            n1573 = call "Database.vi"("Maximum Row"=u64 0 ("Storage Time (Day)"), "Delete row?"=FALSE, "Data"=w4458, "Error in"=w4448, "Auto Increment ID?"=TRUE, "Table"="log_table", "Connection"="dsgs") -> ("Error out"=w4447:errorcluster)  [unwired: 4 in]
          }
          frame 2 {
            n1574 = Get Date/Time In Seconds() -> (seconds since 1Jan1904=w4478:timestamp)
            n1575 = Format Date/Time String(time format string (%c)="%Y/%m/%d", seconds (now)=w4478) -> (date/time string=w4477:string)  [unwired: 1 in]
            n1576 = Format Date/Time String(time format string (%c)="%H:%M:%S", seconds (now)=w4478) -> (date/time string=w4476:string)  [unwired: 1 in]
            n1577 = Bundle("60002", "date/time string"=w4477, "date/time string"=w4476, "Speed signal is changed and applied in disc 30") -> (w4475:T19)  [unwired: 1 in]
            n1578 = To Variant(anything=w4475) -> (Variant=w4474:variant)
            n1579 = call "Database.vi"("Maximum Row"=u64 0 ("Storage Time (Day)"), "Delete row?"=FALSE, "Data"=w4474, "Error in"=w4464, "Auto Increment ID?"=TRUE, "Table"="log_table", "Connection"="dsgs") -> ("Error out"=w4463:errorcluster)  [unwired: 4 in]
          }
          frame 4 {
            n1580 = Get Date/Time In Seconds() -> (seconds since 1Jan1904=w4494:timestamp)
            n1581 = Format Date/Time String(time format string (%c)="%Y/%m/%d", seconds (now)=w4494) -> (date/time string=w4493:string)  [unwired: 1 in]
            n1582 = Format Date/Time String(time format string (%c)="%H:%M:%S", seconds (now)=w4494) -> (date/time string=w4492:string)  [unwired: 1 in]
            n1583 = Bundle("60003", "date/time string"=w4493, "date/time string"=w4492, "Speed signal is changed but not applied in disc 30") -> (w4491:T19)  [unwired: 1 in]
            n1584 = To Variant(anything=w4491) -> (Variant=w4490:variant)
            n1585 = call "Database.vi"("Maximum Row"=u64 0 ("Storage Time (Day)"), "Delete row?"=FALSE, "Data"=w4490, "Error in"=w4480, "Auto Increment ID?"=TRUE, "Table"="log_table", "Connection"="dsgs") -> ("Error out"=w4479:errorcluster)  [unwired: 4 in]
          }
          frame 8 {
            n1586 = Get Date/Time In Seconds() -> (seconds since 1Jan1904=w4509:timestamp)
            n1587 = Format Date/Time String(time format string (%c)="%Y/%m/%d", seconds (now)=w4509) -> (date/time string=w4508:string)  [unwired: 1 in]
            n1588 = Format Date/Time String(time format string (%c)="%H:%M:%S", seconds (now)=w4509) -> (date/time string=w4507:string)  [unwired: 1 in]
            n1589 = Bundle("60004", "date/time string"=w4508, "date/time string"=w4507, "Speed signal is changed but not applied in disc 30") -> (w4506:T19)  [unwired: 1 in]
            n1590 = To Variant(anything=w4506) -> (Variant=w4505:variant)
            n1591 = call "Database.vi"("Delete row?"=FALSE, "Data"=w4505, "Error in"=w4496, "Auto Increment ID?"=TRUE, "Table"="log_table", "Connection"="dsgs") -> ("Error out"=w4495:errorcluster)  [unwired: 5 in]
          }
        }
        n1592 = shared-variable ".\\Setting Lib.lvlib\\processing file path"() -> (w4426:path, error out=w4428:errorcluster)  [unwired: 1 in]
        n1593 = shared-variable ".\\Maintenance.lvlib\\error_51"(w4435) -> ()  [unwired: 1 in, 1 out]
      }
      frame #27 {
        n1594 = shared-variable ".\\control setting.lvlib\\bias"() -> (w4513:dbl[])  [unwired: 1 in, 1 out]
        n1595 = shared-variable ".\\D06.lvlib\\LiveViewD06"() -> (w4516:refnum<image>, error out=w4517:errorcluster)  [unwired: 1 in]
        n1596 = Index Array(array=w4513, index=5) -> (element=w4511:dbl)
        n1597 = To Byte Integer(number=w4511) -> (8bit integer=w4510:i8)
        n1598 = shared-variable ".\\D06.lvlib\\GradingThrD06"() -> (w4533:dbl[], error out=w4534:errorcluster)  [unwired: 1 in]
        n1599 = call "IMAQ Copy"("error in (no error)"=w4517, "Image Dst"=w4529, "Image Src"=w4516) -> ("error out"=w4531:errorcluster, "Image Dst Out"=w4515:T9)  [unwired: 3 in]
        n1600 = property on="DISC 06" class="Bool (strict)"() -> ("Value"=w4526:bool)  [unwired: 2 in, 2 out]
        n1601 = call "find and draw circles.vi"("Image Src"=w4515, "module path"=w4520, "function name"="get_circels", "initialized array"=w4527, "Image Dst"=w4528, "error in (no error)"=w4521, "session in"=w4519, "Run/Stop"=w4526, "grading Thr"=w4533, "bias"=w4510) -> ("session out"=w4524:refnum<k35>, "circle info"=w4525:dbl[][], "Image Out"=w4530:T9, "error out"=w4532:errorcluster, "pellet detected?"=w4523:bool)  [unwired: 5 in]
        n1602 = shared-variable ".\\Maintenance.lvlib\\error_21"(w4531) -> ()  [unwired: 1 in, 1 out]
        n1603 = shared-variable ".\\Maintenance.lvlib\\error_26"(w4532) -> ()  [unwired: 1 in, 1 out]
        n1604 = shared-variable ".\\D06.lvlib\\PelletDetectedD06"(w4530, error in=w4534) -> ()  [unwired: 1 out]
      }
      frame #28 {
        n1605 = shared-variable ".\\Calibration Lib.lvlib\\calibration matrix D06"() -> (w4560:dbl[], error out=w4558:errorcluster)  [unwired: 1 in]
        n1606 = shared-variable ".\\Calibration Lib.lvlib\\calibration factor D06"() -> (w4559:sgl, error out=w4557:errorcluster)  [unwired: 1 in]
        n1607 = Matrix Size(0:w4549) -> (1:w4553:i32)  [unwired: 1 out]
        n1608 = Select(t=w4553, s=w4550, f=0) -> (s? t:f=w4552:i32)
        n1609 = shared-variable ".\\Calibration Lib.lvlib\\Method Selection"(error in=w4558) -> (w4561:enum32{"Method 1", "Method 2"}, error out=w4556:errorcluster)
        n1610 = shared-variable ".\\D06.lvlib\\number of pellet 06"(w4552) -> ()  [unwired: 1 in, 1 out]
        n1611 = case shown="\"Method 2\"" w4561 {
          tunnel: w4548 -> [w4571 w4575]
          tunnel: w4560 -> [_ w4580]
          tunnel: w4559 -> [_ _]
          tunnel: w4549 -> [w4573 w4579]
          tunnel: [w4573 w4577] -> w4547
          tunnel: w4557 -> [w4572 w4578]
          tunnel: [w4572 w4576] -> w4555
          tunnel: [w4571 w4575] -> w4544
          tunnel: w4556 -> [w4570 w4574]
          tunnel: [w4570 w4574] -> w4554
          frame "Method 1", Default {
          }
          frame "Method 2" {
            n1612 = call "pixel2milimetr.vi"("1*3 Transform Matrix"=w4580, "circle array"=w4579, "Error in"=w4578) -> ("calibrated circles"=w4577:dbl[][], "Error out"=w4576:errorcluster)  [unwired: 11 in]
          }
        }
        n1613 = shared-variable ".\\Maintenance.lvlib\\error_31"(w4555, error in=w4554) -> ()  [unwired: 1 out]
      }
      frame #29 {
        n1614 = case shown="True" w4586 {
          tunnel: w4589 -> [_ w4665]
          tunnel: w4591 -> [w4602 w4660]
          tunnel: [w4602 w4659] -> w4590
          tunnel: w4588 -> [w4603 w4655]
          tunnel: [w4603 w4653] -> w4587
          tunnel: w4593 -> [w4601 w4613]
          tunnel: [w4601 w4650] -> w4592
          tunnel: [dbl[] [0.0, 0.0, 0.0, 0.0, 0.0, 0.0, 0.0, 0.0] w4619] -> w4582
          tunnel: [errorcluster {"status"=FALSE, "code"=0, "source"=""} ("error IO") w4637] -> w4583
          frame False {
          }
          frame True {
            w4634 = dbl[] [250.047, 512.0, 857.375, 1331.0, 2048.0, 2744.0, 4096.0]  # fixed threshoulds
            n1615 = shared-variable ".\\D06.lvlib\\GradingThrD06"() -> (w4642:dbl[], error out=w4639:errorcluster)  [unwired: 1 in]
            n1616 = property on="avg grading array size" class="DigNum (strict)"() -> ("Value"=w4611:i32)  [unwired: 2 in, 2 out]
            n1617 = property on="live grading array size" class="DigNum (strict)"() -> ("Value"=w4612:i32)  [unwired: 2 in, 2 out]
            n1618 = Index Array(array=w4665, index (col)=2 ("disabled index (col)")) -> (element=w4652:dbl[])  [unwired: 1 in]
            n1619 = shared-variable ".\\Calibration Lib.lvlib\\Method Selection"(error in=w4639) -> (w4643:enum32{"Method 1", "Method 2"}, error out=w4638:errorcluster)
            n1620 = Array Size(array=w4652) -> (size(s)=w4654:i32)
            n1621 = Subtract(x=w4612, y=w4654) -> (x-y=w4663:i32)
            n1622 = Subtract(x=w4611, y=w4654) -> (x-y=w4658:i32)
            n1623 = Multiply(x=w4634, y=0.125) -> (x*y=w4635:dbl[])
            n1624 = Equal?(x=w4643, y=enum32{"Method 1", "Method 2"}."Method 1" ("Method Selection")) -> (x = y?=w4644:bool)
            n1625 = call "array managment.vi"("2D array in"=w4660, "col sel"=5, "cir num"=w4654, "index"=w4663, "subarray"=w4652) -> ("2D array out"=w4659:dbl[][], "1D array out"=w4661:dbl[])  [unwired: 13 in]
            n1626 = call "array managment.vi"("2D array in"=w4655, "col sel"=5, "cir num"=w4654, "index"=w4658, "subarray"=w4652) -> ("2D array out"=w4653:dbl[][], "1D array out"=w4656:dbl[])  [unwired: 13 in]
            n1627 = Select(t=w4642, s=w4644, f=w4635) -> (s? t:f=w4641:dbl[])
            n1628 = property on="DISC 06" class="Bool (strict)"() -> ("Value"=w4610:bool)  [unwired: 2 in, 2 out]
            n1629 = property on="DISC 06" class="Bool (strict)"() -> ("Value"=w4609:bool)  [unwired: 2 in, 2 out]
            n1630 = call "pelletpercents.vi"("Run/Stop"=w4610, "grading threshoulds"=w4641, "Sorted data"=w4661) -> ("Percentage"=w4646:dbl[])  [unwired: 8 in]
            n1631 = call "pelletpercents.vi"("Run/Stop"=w4609, "grading threshoulds"=w4641, "Sorted data"=w4656) -> ("Percentage"=w4631:dbl[])  [unwired: 8 in]
            n1632 = Number To Fractional String(number=w4646, precision (6)=i16 2) -> (F-format string=w4647:string[])  [unwired: 2 in]
            n1633 = Number To Fractional String(number=w4631, precision (6)=i16 2) -> (F-format string=w4633:string[])  [unwired: 2 in]
            n1634 = property on="DISC 06" class="Bool (strict)"() -> ("Value"=w4608:bool)  [unwired: 2 in, 2 out]
            n1635 = Fract/Exp String To Number(string=w4647) -> (number=w4619:dbl[])  [unwired: 3 in, 1 out]
            n1636 = Fract/Exp String To Number(string=w4633) -> (number=w4604:dbl[])  [unwired: 3 in, 1 out]
            n1637 = call "grading average.vi"("input array"=w4604) -> ("avg"=w4605:dbl)  [unwired: 10 in]
            "AVG 06" <- w4605
            n1638 = shared-variable ".\\D06.lvlib\\AvgResultD06"(w4604, error in=w4638) -> (error out=w4640:errorcluster)
            n1639 = Not A Number/Path/Refnum?(number/path/refnum=w4605) -> (NaN/Path/Refnum?=w4615:bool)
            n1640 = Not(x=w4615) -> (.not. x?=w4614:bool)
            n1641 = Index Array(array=w4619, index #1=3 ("index")) -> (element #1=w4630:dbl, element #2=w4627:dbl, element #3=w4628:dbl, element #4=w4629:dbl)  [unwired: 3 in]
            n1642 = And(x=w4608, y=w4614) -> (x .and. y?=w4616:bool)
            n1643 = Add(x=w4630, y=w4627) -> (x+y=w4607:dbl)
            "9.5-12.7 06" <- w4607
            n1644 = Add(x=w4628, y=w4629) -> (x+y=w4606:dbl)
            "12.7-16 06" <- w4606
            n1645 = Add(x=w4627, y=w4628) -> (x+y=w4622:dbl)
            "10-14 6" <- w4622
            n1646 = shared-variable ".\\D06.lvlib\\LiveResultD06"(w4619, error in=w4640) -> (error out=w4637:errorcluster)
            n1647 = Add(x=w4606, y=w4607) -> (x+y=→"8-16mm 6":dbl)
            n1648 = Select(t=w4605, s=w4616, f=12.0) -> (s? t:f=w4617:dbl)
            n1649 = call "dif array management.vi"("2D array in"=w4613, "col sel"=5, "new element/subarray"=w4617) -> ("2D array out"=w4650:dbl[][])  [unwired: 15 in, 1 out]
            n1650 = Greater Or Equal?(x=w4622, y=70.0) -> (x >= y?=w4625:bool)
            n1651 = Select(t=u32 65282 ("Fill Color"), s=w4625, f=u32 4018019 ("Fill Color")) -> (s? t:f=w4621:u32)
            n1652 = property on="10-14 6" class="Slide (strict)"("Fill Color"=w4621) -> ()  [unwired: 2 in, 2 out]
          }
        }
      }
      frame #30 {
        n1653 = shared-variable ".\\D06.lvlib\\SaveD06"(error in=w4668) -> (w4675:bool, error out=w4678:errorcluster)
        n1654 = Index Array(array=w4669, index (col)=5 ("disabled index (col)")) -> (element=w4672:dbl[])  [unwired: 1 in]
        n1655 = Boolean To (0,1)(Boolean=w4675) -> (0, 1=w4674:i16)
        n1656 = case shown="True" w4666 {
          tunnel: w4667 -> [_ w4695]
          frame False {
          }
          frame True {
            w4690 = enum16{"ID Delete", "Time Delete"}."Time Delete" ("Enum")
            n1657 = property on="projector 06" class="Bool (strict)"() -> ("Value"=w4725:bool)  [unwired: 2 in, 2 out]
            n1658 = Select(t="ON" ("time format string (%c)"), s=w4725, f="OFF" ("time format string (%c)")) -> (s? t:f=w4726:string)
            n1659 = property on="cam 06" class="Bool (strict)"() -> ("Value"=w4723:bool)  [unwired: 2 in, 2 out]
            n1660 = Select(t="ON" ("time format string (%c)"), s=w4723, f="OFF" ("time format string (%c)")) -> (s? t:f=w4724:string)
            n1661 = property on="AUTO/MAN 06" class="Bool (strict)"() -> ("Value"=w4721:bool)  [unwired: 2 in, 2 out]
            n1662 = Select(t="Auto", s=w4721, f="Manual") -> (s? t:f=w4722:string)
            n1663 = property on="DISC 06" class="Bool (strict)"() -> ("Value"=w4719:bool)  [unwired: 2 in, 2 out]
            n1664 = Select(t="Run", s=w4719, f="Stop") -> (s? t:f=w4720:string)
            n1665 = Get Date/Time In Seconds() -> (seconds since 1Jan1904=w4716:timestamp)
            n1666 = Format Date/Time String(time format string (%c)="%Y/%m/%d", seconds (now)=w4716) -> (date/time string=w4717:string)  [unwired: 1 in]
            n1667 = Format Date/Time String(time format string (%c)="%H:%M:%S", seconds (now)=w4716) -> (date/time string=w4718:string)  [unwired: 1 in]
            n1668 = Index Array(array=w4695, index #1=0 ("index")) -> (element #1=w4708:dbl, element #2=w4709:dbl, element #3=w4710:dbl, element #4=w4711:dbl, element #5=w4712:dbl, element #6=w4713:dbl, element #7=w4714:dbl, element #8=w4715:dbl)  [unwired: 7 in]
            n1669 = Bundle("date/time string"=w4717, "date/time string"=w4718, w4708, w4709, w4710, w4711, w4712, w4713, w4714, w4715, "f"=w4720, "f"=w4722, "time format string (%c)"=w4724, "time format string (%c)"=w4726) -> (w4696:T36)  [unwired: 1 in]
            n1670 = shared-variable ".\\Setting Lib.lvlib\\database refresh period"() -> (w4694:i32, error out=w4693:errorcluster)  [unwired: 1 in]
            n1671 = Unbundle(w4696) -> ("date/time string"=w4740:string, "date/time string"=w4739:string, w4738:dbl, w4735:dbl, w4734:dbl, w4737:dbl, "f"=w4732:string, "f"=w4731:string, "time format string (%c)"=w4730:string, "time format string (%c)"=w4729:string)  [unwired: 4 out]
            n1672 = Add(x=w4735, y=w4734) -> (x+y=w4733:dbl)
            n1673 = Compound Arithmetic op=ADD(w4738, w4735, w4734, w4737) -> (w4736:dbl)
            n1674 = To Variant(anything=w4696) -> (Variant=w4741:variant)
            n1675 = call "Database.vi"("Maximum Row"=w4694, "Enum"=w4690, "Delete row?"=TRUE, "Data"=w4741, "Error in"=w4693, "Auto Increment ID?"=TRUE, "Table"="grading_disc_06", "Connection"="dsgs") -> ("Error out"=w4691:errorcluster)  [unwired: 3 in]
            n1676 = Bundle("date/time string"=w4740, "date/time string"=w4739, w4736, w4733, "f"=w4732, "f"=w4731, "time format string (%c)"=w4730, "time format string (%c)"=w4729) -> (w4728:T37)  [unwired: 1 in]
            n1677 = shared-variable ".\\Maintenance.lvlib\\error_40"(w4691) -> ()  [unwired: 1 in, 1 out]
            n1678 = To Variant(anything=w4728) -> (Variant=w4727:variant)
            n1679 = call "Database.vi"("Maximum Row"=w4694, "Enum"=w4690, "Delete row?"=TRUE, "Data"=w4727, "Auto Increment ID?"=TRUE, "Table"="main_grading_group_disc_06", "Connection"="dsgs") -> ("Error out"=w4692:errorcluster)  [unwired: 4 in]
            n1680 = shared-variable ".\\Maintenance.lvlib\\error_41"(w4692) -> ()  [unwired: 1 in, 1 out]
          }
        }
        n1681 = Build Array(w4674) -> (w4673:i16[])
        n1682 = call-poly <vilib>:"Basic Level Trigger Detection.vi"("signal in"=w4673, "level"=0.5, "error in (no error)"=w4678) -> ("trigger detected?"=w4670:bool, "error out"=w4679:errorcluster)  [unwired: 10 in, 1 out]
        n1683 = case shown="True" w4670 {
          selector: w4670 -> [_ w4765]
          tunnel: [FALSE w4765] -> w4671
          tunnel: w4672 -> [_ w4760]
          tunnel: w4679 -> [w4751 w4753]
          tunnel: [w4751 w4752] -> w4680
          frame False {
          }
          frame True {
            n1684 = Array To Spreadsheet String(array=w4760, 3:"%.2f" ("format string")) -> (spreadsheet string=w4764:string)  [unwired: 1 in]
            n1685 = Get Date/Time In Seconds() -> (seconds since 1Jan1904=w4761:timestamp)
            n1686 = Format Date/Time String(time format string (%c)="%H:%M:%S", seconds (now)=w4761) -> (date/time string=w4763:string)  [unwired: 1 in]
            n1687 = Format Date/Time String(time format string (%c)="%Y/%m/%d", seconds (now)=w4761) -> (date/time string=w4762:string)  [unwired: 1 in]
            n1688 = Bundle("date/time string"=w4762, "date/time string"=w4763, "disc 06", "spreadsheet string"=w4764) -> (w4755:T38)  [unwired: 1 in]
            n1689 = To Variant(anything=w4755) -> (Variant=w4754:variant)
            n1690 = call "Database.vi"("Delete row?"=FALSE, "Data"=w4754, "Error in"=w4753, "Auto Increment ID?"=TRUE, "Table"="thresholds_calibration_table", "Connection"="dsgs") -> ("Error out"=w4752:errorcluster)  [unwired: 5 in]
          }
        }
        n1691 = shared-variable ".\\D06.lvlib\\SaveD06Ok"(w4671, error in=w4680) -> ()  [unwired: 1 out]
        n1692 = shared-variable ".\\Maintenance.lvlib\\error_46"(w4680) -> ()  [unwired: 1 in, 1 out]
      }
      frame #31 {
        n1693 = shared-variable ".\\D06.lvlib\\LiveResultD06"() -> (w4811:dbl[])  [unwired: 1 in, 1 out]
        n1694 = shared-variable ".\\D05.lvlib\\LiveResultD05"() -> (w4855:dbl[])  [unwired: 1 in, 1 out]
        n1695 = shared-variable ".\\D02.lvlib\\LiveResultD02"() -> (w4861:dbl[])  [unwired: 1 in, 1 out]
        n1696 = shared-variable ".\\D01.lvlib\\liveResultArray"() -> (w4864:dbl[])  [unwired: 1 in, 1 out]
        n1697 = shared-variable ".\\D04.lvlib\\LiveResultD04"() -> (w4860:dbl[])  [unwired: 1 in, 1 out]
        n1698 = shared-variable ".\\D03.lvlib\\LiveResultD03"() -> (w4857:dbl[])  [unwired: 1 in, 1 out]
        n1699 = shared-variable ".\\D06.lvlib\\LiveResultD06"() -> (w4788:dbl[])  [unwired: 1 in, 1 out]
        n1700 = shared-variable ".\\D05.lvlib\\LiveResultD05"() -> (w4854:dbl[])  [unwired: 1 in, 1 out]
        n1701 = shared-variable ".\\D04.lvlib\\LiveResultD04"() -> (w4849:dbl[])  [unwired: 1 in, 1 out]
        n1702 = shared-variable ".\\D03.lvlib\\LiveResultD03"() -> (w4852:dbl[])  [unwired: 1 in, 1 out]
        n1703 = shared-variable ".\\D02.lvlib\\LiveResultD02"() -> (w4848:dbl[])  [unwired: 1 in, 1 out]
        n1704 = shared-variable ".\\D01.lvlib\\liveResultArray"() -> (w4845:dbl[])  [unwired: 1 in, 1 out]
        n1705 = property on="9.5-12.7 01" class="Slide (strict)"() -> ("Value"=w4890:dbl)  [unwired: 2 in, 2 out]
        n1706 = property on="9.5-12.7 02" class="Slide (strict)"() -> ("Value"=w4889:dbl)  [unwired: 2 in, 2 out]
        n1707 = property on="9.5-12.7 03" class="Slide (strict)"() -> ("Value"=w4888:dbl)  [unwired: 2 in, 2 out]
        n1708 = property on="9.5-12.7 04" class="Slide (strict)"() -> ("Value"=w4887:dbl)  [unwired: 2 in, 2 out]
        n1709 = property on="9.5-12.7 05" class="Slide (strict)"() -> ("Value"=w4886:dbl)  [unwired: 2 in, 2 out]
        n1710 = property on="12.7-16 06" class="Slide (strict)"() -> ("Value"=w4780:dbl)  [unwired: 2 in, 2 out]
        n1711 = property on="9.5-12.7 06" class="Slide (strict)"() -> ("Value"=w4777:dbl)  [unwired: 2 in, 2 out]
        n1712 = property on="12.7-16 01" class="Slide (strict)"() -> ("Value"=w4877:dbl)  [unwired: 2 in, 2 out]
        n1713 = property on="12.7-16 02" class="Slide (strict)"() -> ("Value"=w4876:dbl)  [unwired: 2 in, 2 out]
        n1714 = property on="12.7-16 03" class="Slide (strict)"() -> ("Value"=w4875:dbl)  [unwired: 2 in, 2 out]
        n1715 = property on="12.7-16 04" class="Slide (strict)"() -> ("Value"=w4874:dbl)  [unwired: 2 in, 2 out]
        n1716 = property on="12.7-16 05" class="Slide (strict)"() -> ("Value"=w4873:dbl)  [unwired: 2 in, 2 out]
        n1717 = property on="AVG 04" class="DigNum (strict)"() -> ("Value"=w4827:dbl)  [unwired: 2 in, 2 out]
        n1718 = property on="AVG 02" class="DigNum (strict)"() -> ("Value"=w4829:dbl)  [unwired: 2 in, 2 out]
        n1719 = property on="AVG 03" class="DigNum (strict)"() -> ("Value"=w4828:dbl)  [unwired: 2 in, 2 out]
        n1720 = property on="AVG 06" class="DigNum (strict)"() -> ("Value"=w4774:dbl)  [unwired: 2 in, 2 out]
        n1721 = property on="AVG 01" class="DigNum (strict)"() -> ("Value"=w4830:dbl)  [unwired: 2 in, 2 out]
        n1722 = property on="AVG 05" class="DigNum (strict)"() -> ("Value"=w4826:dbl)  [unwired: 2 in, 2 out]
        n1723 = property on="DISC 06" class="Bool (strict)"() -> ("Value"=w4797:bool)  [unwired: 2 in, 2 out]
        n1724 = property on="DISC 01" class="Bool (strict)"() -> ("Value"=w4895:bool)  [unwired: 2 in, 2 out]
        n1725 = property on="DISC 02" class="Bool (strict)"() -> ("Value"=w4893:bool)  [unwired: 2 in, 2 out]
        n1726 = property on="DISC 03" class="Bool (strict)"() -> ("Value"=w4892:bool)  [unwired: 2 in, 2 out]
        n1727 = property on="DISC 04" class="Bool (strict)"() -> ("Value"=w4891:bool)  [unwired: 2 in, 2 out]
        n1728 = property on="DISC 05" class="Bool (strict)"() -> ("Value"=w4894:bool)  [unwired: 2 in, 2 out]
        n1729 = Boolean To (0,1)(Boolean=w4895) -> (0, 1=w4822:i16)
        n1730 = Boolean To (0,1)(Boolean=w4893) -> (0, 1=w4821:i16)
        n1731 = Boolean To (0,1)(Boolean=w4892) -> (0, 1=w4820:i16)
        n1732 = Boolean To (0,1)(Boolean=w4891) -> (0, 1=w4819:i16)
        n1733 = Boolean To (0,1)(Boolean=w4894) -> (0, 1=w4818:i16)
        n1734 = Boolean To (0,1)(Boolean=w4797) -> (0, 1=w4776:i16)
        n1735 = Index Array(array=w4811, index #1=0 ("index")) -> (element #1=w4812:dbl, element #2=w4813:dbl, element #3=w4773:dbl)  [unwired: 2 in]
        n1736 = Index Array(array=w4855, index #1=0 ("index")) -> (element #1=w4816:dbl, element #2=w4815:dbl, element #3=w4814:dbl)  [unwired: 2 in]
        n1737 = Index Array(array=w4861, index #1=0 ("index")) -> (element #1=w4803:dbl, element #2=w4802:dbl, element #3=w4801:dbl)  [unwired: 2 in]
        n1738 = Index Array(array=w4864, index #1=0 ("index")) -> (element #1=w4800:dbl, element #2=w4799:dbl, element #3=w4798:dbl)  [unwired: 2 in]
        n1739 = Index Array(array=w4860, index #1=0 ("index")) -> (element #1=w4808:dbl, element #2=w4807:dbl, element #3=w4809:dbl)  [unwired: 2 in]
        n1740 = Index Array(array=w4857, index #1=0 ("index")) -> (element #1=w4806:dbl, element #2=w4805:dbl, element #3=w4804:dbl)  [unwired: 2 in]
        n1741 = Index Array(array=w4788, index=7) -> (element=w4787:dbl)
        n1742 = Index Array(array=w4854, index=7) -> (element=w4786:dbl)
        n1743 = Index Array(array=w4849, index=7) -> (element=w4785:dbl)
        n1744 = Index Array(array=w4852, index=7) -> (element=w4784:dbl)
        n1745 = Index Array(array=w4848, index=7) -> (element=w4783:dbl)
        n1746 = Index Array(array=w4845, index=7) -> (element=w4782:dbl)
        n1747 = Compound Arithmetic op=ADD(w4812, w4813, w4773) -> (w4796:dbl)
        n1748 = Compound Arithmetic op=ADD(w4816, w4815, w4814) -> (w4795:dbl)
        n1749 = Compound Arithmetic op=ADD(w4808, w4807, w4809) -> (w4794:dbl)
        n1750 = Compound Arithmetic op=ADD(w4806, w4805, w4804) -> (w4793:dbl)
        n1751 = Compound Arithmetic op=ADD(w4803, w4802, w4801) -> (w4792:dbl)
        n1752 = Compound Arithmetic op=ADD(w4800, w4799, w4798) -> (w4791:dbl)
        n1753 = shared-variable ".\\control setting.lvlib\\Error2DArray"(w4770) -> ()  [unwired: 1 in, 1 out]
        n1754 = Multiply(x=w4796, y=w4776) -> (x*y=w4790:dbl)
        n1755 = Multiply(x=w4780, y=w4776) -> (x*y=w4779:dbl)
        n1756 = Multiply(x=w4795, y=w4818) -> (x*y=w4844:dbl)
        n1757 = Multiply(x=w4794, y=w4819) -> (x*y=w4843:dbl)
        n1758 = Multiply(x=w4793, y=w4820) -> (x*y=w4842:dbl)
        n1759 = Multiply(x=w4792, y=w4821) -> (x*y=w4841:dbl)
        n1760 = Multiply(x=w4791, y=w4822) -> (x*y=w4840:dbl)
        n1761 = Multiply(x=w4877, y=w4822) -> (x*y=w4871:dbl)
        n1762 = Multiply(x=w4876, y=w4821) -> (x*y=w4869:dbl)
        n1763 = Multiply(x=w4875, y=w4820) -> (x*y=w4872:dbl)
        n1764 = Multiply(x=w4874, y=w4819) -> (x*y=w4870:dbl)
        n1765 = Multiply(x=w4873, y=w4818) -> (x*y=w4781:dbl)
        n1766 = Multiply(x=w4890, y=w4822) -> (x*y=w4880:dbl)
        n1767 = Multiply(x=w4889, y=w4821) -> (x*y=w4881:dbl)
        n1768 = Multiply(x=w4888, y=w4820) -> (x*y=w4882:dbl)
        n1769 = Multiply(x=w4887, y=w4819) -> (x*y=w4878:dbl)
        n1770 = Multiply(x=w4886, y=w4818) -> (x*y=w4879:dbl)
        n1771 = Multiply(x=w4777, y=w4776) -> (x*y=w4775:dbl)
        n1772 = Compound Arithmetic op=ADD(w4822, w4821, w4820, w4819, w4818, w4776) -> (w4884:i16)
        n1773 = Multiply(x=w4787, y=w4776) -> (x*y=w4772:dbl)
        n1774 = Compound Arithmetic op=ADD(w4830, w4829, w4828, w4827, w4826, w4774) -> (w4825:dbl)
        n1775 = Multiply(x=w4786, y=w4818) -> (x*y=w4839:dbl)
        n1776 = Multiply(x=w4785, y=w4819) -> (x*y=w4838:dbl)
        n1777 = Multiply(x=w4784, y=w4820) -> (x*y=w4837:dbl)
        n1778 = Multiply(x=w4783, y=w4821) -> (x*y=w4836:dbl)
        n1779 = Multiply(x=w4782, y=w4822) -> (x*y=w4835:dbl)
        n1780 = Equal To 0?(x=w4884) -> (x = 0?=w4885:bool)
        n1781 = Compound Arithmetic op=ADD(w4790, w4844, w4843, w4842, w4841, w4840) -> (w4834:dbl)
        n1782 = Compound Arithmetic op=ADD(w4772, w4839, w4838, w4837, w4836, w4835) -> (w4833:dbl)
        n1783 = Select(t=i16 1, s=w4885, f=w4884) -> (s? t:f=w4824:i16)
        n1784 = Compound Arithmetic op=ADD(w4871, w4869, w4872, w4870, w4781, w4779) -> (w4867:dbl)
        n1785 = Compound Arithmetic op=ADD(w4880, w4881, w4882, w4878, w4879, w4775) -> (w4868:dbl)
        n1786 = Divide(x=w4834, y=w4824) -> (x/y=→"Under Size":dbl)
        n1787 = Divide(x=w4867, y=w4824) -> (x/y=w4866:dbl)
        "12.7-16 total" <- w4866
        n1788 = Divide(x=w4833, y=w4824) -> (x/y=→"Over Size":dbl)
        n1789 = Divide(x=w4868, y=w4824) -> (x/y=w4865:dbl)
        "9.5-12.7 total" <- w4865
        n1790 = Divide(x=w4825, y=w4824) -> (x/y=→"AVG":dbl)
        n1791 = Add(x=w4866, y=w4865) -> (x+y=→"In Range":dbl)
        "2D array out" <- w4770
      }
    }
  }
  n1792 = call <userlib>:"DAQNavi Stop Task.vi"("error in (no error)"=w3, "task in"=w5) -> ("error out"=w2:errorcluster)  [unwired: 1 out]
  n1793 = call <userlib>:"DAQNavi Stop Task.vi"("error in (no error)"=w2, "task in"=w4) -> ("error out"=→"error out 2":errorcluster)  [unwired: 1 out]
  n1794 = Close Python Session(session in=w117) -> (11:w55:errorcluster)  [unwired: 1 in]
  n1795 = shared-variable ".\\Maintenance.lvlib\\error_52"(w55) -> ()  [unwired: 1 in, 1 out]
  "live grading array size" <- w105
  "avg grading array size" <- w100
  "disc name 06" <- "DISC 06" ("disc name 06")
  "disc name 07" <- "DISC 07" ("disc name 07")
  "Software name" <- "DORSA Smart Grading System (DSGS)" ("time format string (%c)")
  "disc name 01" <- "DISC 01" ("disc 26 name")
  "disc name 02" <- "DISC 02" ("disc name 27")
  "disc name 03" <- "DISC 03" ("disc name 28")
  "disc name 04" <- "DISC 04" ("disc name 29")
  "disc name 05" <- "DISC 05" ("disc name 30")
  "overal result" <- "Overal Result" ("overal result")
